vi "SpectrometerSpinCoater_v14.vi"() -> ()   [LabVIEW 2020]
uses:
  TypDef/TabControl_InSitu_Type.ctl
  <instrlib>/Classes/CCD/Abstract_CCD/Abstract_CCD.lvclass
  <instrlib>/Classes/SpinCoater/SpinCoater.lvclass
  TypDef/Preset_Save_v14_1.ctl
  TypDef/DeviceQueue_TypeDef.ctl
  TypDef/DeviceQueue_Action.ctl
  TypDef/TabControl.ctl
  TypDef/DataQueue_TypeDef.ctl
  TypDef/DataQueue_Action.ctl
  <vilib>/Utility/error.llb/DialogType.ctl
  <instrlib>/Classes/CCD/Avantes/Avantes.lvclass
  C:/Program Files/National Instruments/LabVIEW 2020/instr.lib/Classes/CCD/Abstract_CCD/Abstract_CCD.lvclass
  <vilib>/Analysis/baseanly.llb/A x Vector.vi
  <vilib>/Utility/xml.llb/Write to XML File(string).vi
  <vilib>/Utility/xml.llb/Read From XML File(string).vi
  <vilib>/Analysis/NI_AALBase.lvlib
panel:
  out "fName_Temp":string
  out "x-y":dbl
  in  "Reference\nValue":dbl=1.0
  out "WL-Det\nPos":i32
  in  "Motor_ShortStop":bool
  out "UpperWLLimit":i32=1065
  out "LowerWLLimit":i32=149
  out "Nr After Spin":u16
  out "Action":string="TimeOut"
  out "Time.spin":refnum<file>
  out "Meas.spin":refnum<file>
  in  "Abort Button":bool
  in  "Stop Button":bool=TRUE
  in  "Tab Control":T1(tab)=enum."Settings"
  in  "MeasureOpenPreset":bool
  in  "MeasureSavePreset":bool
  in  "Cell":string
  in  "TrimSpec":bool=TRUE caption="Trim\nSpec"
  in  "WlUp":dbl[unit]=9.102385253906251e-07 caption="Wl \nUp"
  in  "WlLow":dbl[unit]=3.7998095703125003e-07 caption="Wl \nLow"
  in  "Frames for Ref/Dark":dbl=10000.0
  in  "Shutter Toggle":bool
  in  "Program Spin Coater":T2(array[cluster])=[{"Speed (rpm)"=1430.0, "Time (s)"=45.0, "Acc (rpm/s)"=0.0}]
  in  "Spectra Count":u16
  in  "Measure_MeasureSpectrum":bool
  out "Overall Time":dbl=47.0
  in  "Frames":i32=123685
  in  "StartMeasurement_Button":bool
  in  "Measure_Preview":bool
  out "Measure_Graph":T3(graph) caption="XY Graph"
  in  "Measure_FramesSpectrometer":dbl=200.0 caption="Frames for Spectrometer"
  in  "StartSpin_Button":bool
  in  "Record RefSpec":bool
  in  "Measure:\nRecord_Darkspec":bool
  in  "Measure_Comments":string="Just for testing" caption="Comments"
  in  "Measure_FileName":string="Testing" caption="File Name"
  in  "Measure_SavePath":path=path "C:/Users/Cerberus/Desktop/Test/v12Test" caption="Save Path"
  out "Measure_FrameRate":dbl[unit]=2631.5791015625 caption="Frame Rate"
  in  "Measure_IntegrationTime":dbl[unit]=3e-05 caption="Integration Time"
  in  "Tab Control SpinType":T4
  in  "Seconds after Spin":dbl[unit]=1.0
  in  "Calculate Frames_Normal":bool=TRUE caption="Calculate Frames"
  in  "periodic time":dbl[unit]=2.0
  in  "Duration after":dbl[unit]
  in  "Spin at end":bool
  in  "Seconds to Spin_Normal":dbl[unit]=1.0 caption="Seconds to Spin"
  in  "Threshold":dbl=0.3
  in  "Time Detect":dbl[unit]=2.0
  in  "Seconds to Spin_Short":dbl[unit]=1.0 caption="Seconds to Spin"
  in  "Spin Time":dbl[unit]=2.0
  in  "Calculate Frames_Short":bool=TRUE caption="Calculate Frames"
  in  "Wavelenght Detect":dbl[unit]=6.000000000000001e-07
  out "SS_StepsLeft":dbl
  out "SS_TimePrediction":dbl[unit]=-6.0
  out "Horizontal Progress Bar":u8(slide) scale=0.0..100.0
  in  "SpectralStability:\nRecord_Darkspec":bool
  in  "SpectralStability_Record":bool
  in  "SpectralStability_\nMeasurementNumber":u32 caption="Measurement Number"
  in  "SpectralStability_Duration":dbl[unit] caption="Duration"
  in  "Duration/Times":bool
  in  "SpectralStability_\nPeriodicTime":dbl[unit] caption="Periodic Time"
  in  "SpectralStability_MeasureSpectrum":bool
  in  "SpectralStability_Preview":bool
  out "SpectralStability_Graph":T3(graph) caption="XY Graph"
  in  "SpectralStability_FramesSpectrometer":dbl=200.0 caption="Frames for Spectrometer"
  in  "SpectralStability_Comments":string="Just for testing" caption="Comments"
  in  "SpectralStability_FileName":string="TestingAfter" caption="File Name"
  in  "SpectralStability_SavePath":path=path "C:/Users/Timo/Desktop/Test/180824" caption="Save Path"
  out "SpectralStability_FrameRate":dbl[unit]=2631.5791015625 caption="Frame Rate"
  in  "SpectralStability_IntegrationTime":dbl[unit]=3e-05 caption="Integration Time"
  in  "Shutter Close":bool
  in  "Shutter Open":bool
  in  "SHUTTER DEBUG":bool
  in  "Shutter Position":u16=1000
  in  "Dividider Get Spectra":u32=1 min=1
  in  "Automatically \nadjust count":bool=TRUE
  in  "Reset Count\nafter Spin Coating":bool=TRUE
  in  "ESC_Speed":dbl
  in  "ESC_Milliseconds":dbl
  in  "ESC DEBUG":bool
  in  "Port Arduino":refnum<visa-resource-name>="COM7"
  out "Error Arduino":bool caption="Error"
  in  "Init_Arduino":bool caption="Init"
  out "Caption_Settings_Arduino":string="Arduino"
  out "Caption_Settings_NKT":string="NKT Laser"
  out "Error_Spectromter":bool caption="Error"
  in  "Init_Spectrometer":bool caption="Init"
  out "Caption_Settings_Spectrometer":string="Spectromter"
  out "Arduino":bool
  out "NKT":bool
  out "Spectromter":bool
  # "Speed (rpm)   Time (s)        Acceleration \n                                               (rpm/s)"
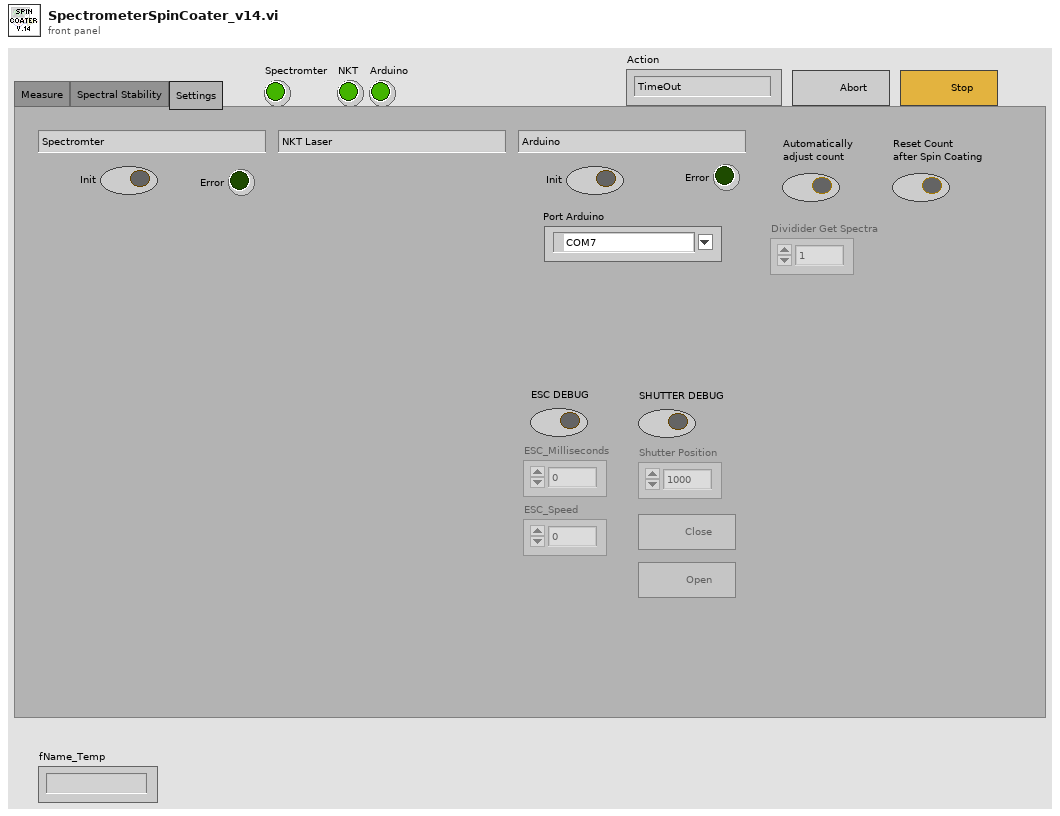
[diagram p1: front panel]
types:
  T1 = enum32{"Measure", "Spectral Stability", "Settings"}
  T2 = cluster{"Speed (rpm)":dbl, "Time (s)":dbl, "Acc (rpm/s)":dbl}[]
  T3 = cluster{"Wavlength":dbl[unit][], "Image":dbl[]}[]
  T4 = typedef "TabControl_InSitu_Type.ctl" = enum32{"Normal", "Short"}
  T5 = cluster{"Dark":cluster{"Image":dbl[][][], "Frame Size":cluster{"F":i32, "Y":i32, "X":i32}}[], "Ref":cluster{"Image":dbl[][][], "Frame Size":cluster{"F":i32, "Y":i32, "X":i32}}[], "Wavlength":dbl[unit][], "Wavlength Trim":dbl[unit][], "spec":dbl[][]}
  T6 = cluster{"Abstract_CCD.lvclass":refnum<class "Abstract_CCD.lvclass">, "SpinCoater.lvclass":refnum<class "SpinCoater.lvclass">}
  T7 = enum8{"Enabled", "Disabled", "Disabled and Grayed Out"}
  T8 = typedef "DataQueue_TypeDef.ctl" = cluster{"QueueAction":T9, "Data":cluster{"Image":dbl[][][], "Frame Size":cluster{"F":i32, "Y":i32, "X":i32}}[], "Data_Raw":cluster{"Image":dbl[][][], "Frame Size":cluster{"F":i32, "Y":i32, "X":i32}}[], "Data_Dark":cluster{"Image":dbl[][][], "Frame Size":cluster{"F":i32, "Y":i32, "X":i32}}[], "Data_Ref":cluster{"Image":dbl[][][], "Frame Size":cluster{"F":i32, "Y":i32, "X":i32}}[], "Device Information":string[], "Numeric Control":dbl, "Boolean":bool, "Wavelength":dbl[unit][], "Time":dbl[], "Time Stamp":timestamp, "Numeric Control 2":dbl, "TabControl":T10, "Numeric Control 3":dbl}
  T9 = typedef "DataQueue_Action.ctl" = enum16{"TimeOut", "Close_Program", "Abort", "Stop_Measurement", "Measure_InSituSpinCoating", "Measure_InSituSpinCoating_Short", "Measure_Spectrum", "Measure_SpectrumAdvanced", "Measure_SpectralStability", "Save_InSitu", "Save_SpectralStability", "Set_Ref", "Set_Dark", "Set_Wavelength", "Spectrometer_Measure", "Spectrometer_Preview", "Transfer_Settings", "Change_TrimSettings"}
  T10 = typedef "TabControl.ctl" = enum16{"Measure", "Spectral Stability", "Settings"}
  T11 = typedef "DeviceQueue_TypeDef.ctl" = cluster{"QueueAction":T12, "Numeric 1":dbl, "Numeric 2":dbl, "Boolean 1":bool, "Boolean 2":bool, "Spin Program":dbl[][], "Spin Prg v07":cluster{"Speed (rpm)":dbl, "Time (s)":dbl, "Acc (rpm/s)":dbl}[], "Time Stamp":timestamp, "TabControl":T10}
  T12 = typedef "DeviceQueue_Action.ctl" = enum16{"TimeOut", "Wait", "Close_Program", "Abort", "Spectrometer_Init", "Spectrometer_Close", "Spectrometer_DeviceInformation", "Spectrometer_Measure", "Spectrometer_MeasureAdvanced", "Spectrometer_Preview", "Spectrometer_Abort", "Spectrometer_StartMeasurement", "Spectrometer_GetData", "Spectrometer_GetData_Short", "Spectrometer_StopMeasurement", "Spectrometer_SetIntegrationTime", "Spectrometer_SetFrames", "Spectrometer_SetDarkspec", "Spectrometer_SetReference", "Spectrometer_SetTriggerMode", "Laser_Init", "Laser_Close", "Arduino_Init", "Arduino_Close", "Arduino_LoadProgram", "Arduino_StartProgram", "Arduino_SetSpeed", "Arduino_SetMillis", "Arduino_StopSpin", "Arduino_ShortStop", "Arduino_Shutter_SetPosition", "Arduino_Shutter_Close", "Arduino_Shutter_Open", "Measure_InSitu", "Measure_Spectrum", "Measure_InSituAdvanced", "Measure_InSituAdvanced_Short", "Measure_SpectralStability", "Measure_Stop"}
  T13 = enum16{"open", "replace", "create", "open or create", "replace or create", "replace or create with confirmation"}
  T14 = cluster{"Image":dbl[][][], "Frame Size":cluster{"F":i32, "Y":i32, "X":i32}}[]
  T15 = cluster{"Image":dbl[][][], "Frame Size":cluster{"F":i32, "Y":i32, "X":i32}}
  T16 = cluster{"Wavlength":dbl[unit][], "A x Vector":dbl[]}
  T17 = cluster{"Wavlength":dbl[unit][], "A x Vector":dbl[]}[]
  T18 = cluster{u16[][][], u16[][][], dbl[], "Numeric Control":dbl, "Numeric Control 2":dbl}
  T19 = typedef "DialogType.ctl" = u16
  T20 = typedef "Preset_Save_v14_1.ctl" = cluster{"Measure_IntegrationTime":dbl, "Measure_FramesSpec":dbl, "Frames_ForRef/Dark":dbl, "Program Spin Coater":cluster{"Speed (rpm)":dbl, "Time (s)":dbl, "Acc (rpm/s)":dbl}[], "TabControlSpinType":u32, "Seconds2Spin_Norm":dbl, "SecondsAftSpin_Norm":dbl, "CalcFrames_Norm":bool, "PeriodicTime":dbl, "DurationAfter":dbl, "SpinAtEnd":bool, "Seconds2Spin_Short":dbl, "SpinTime":dbl, "CalculateFrames_Short":bool, "TimeDetect":dbl, "WavelengthDetect":dbl, "Threshold":dbl, "WlLow":dbl, "WlUp":dbl, "TrimSpec":bool}
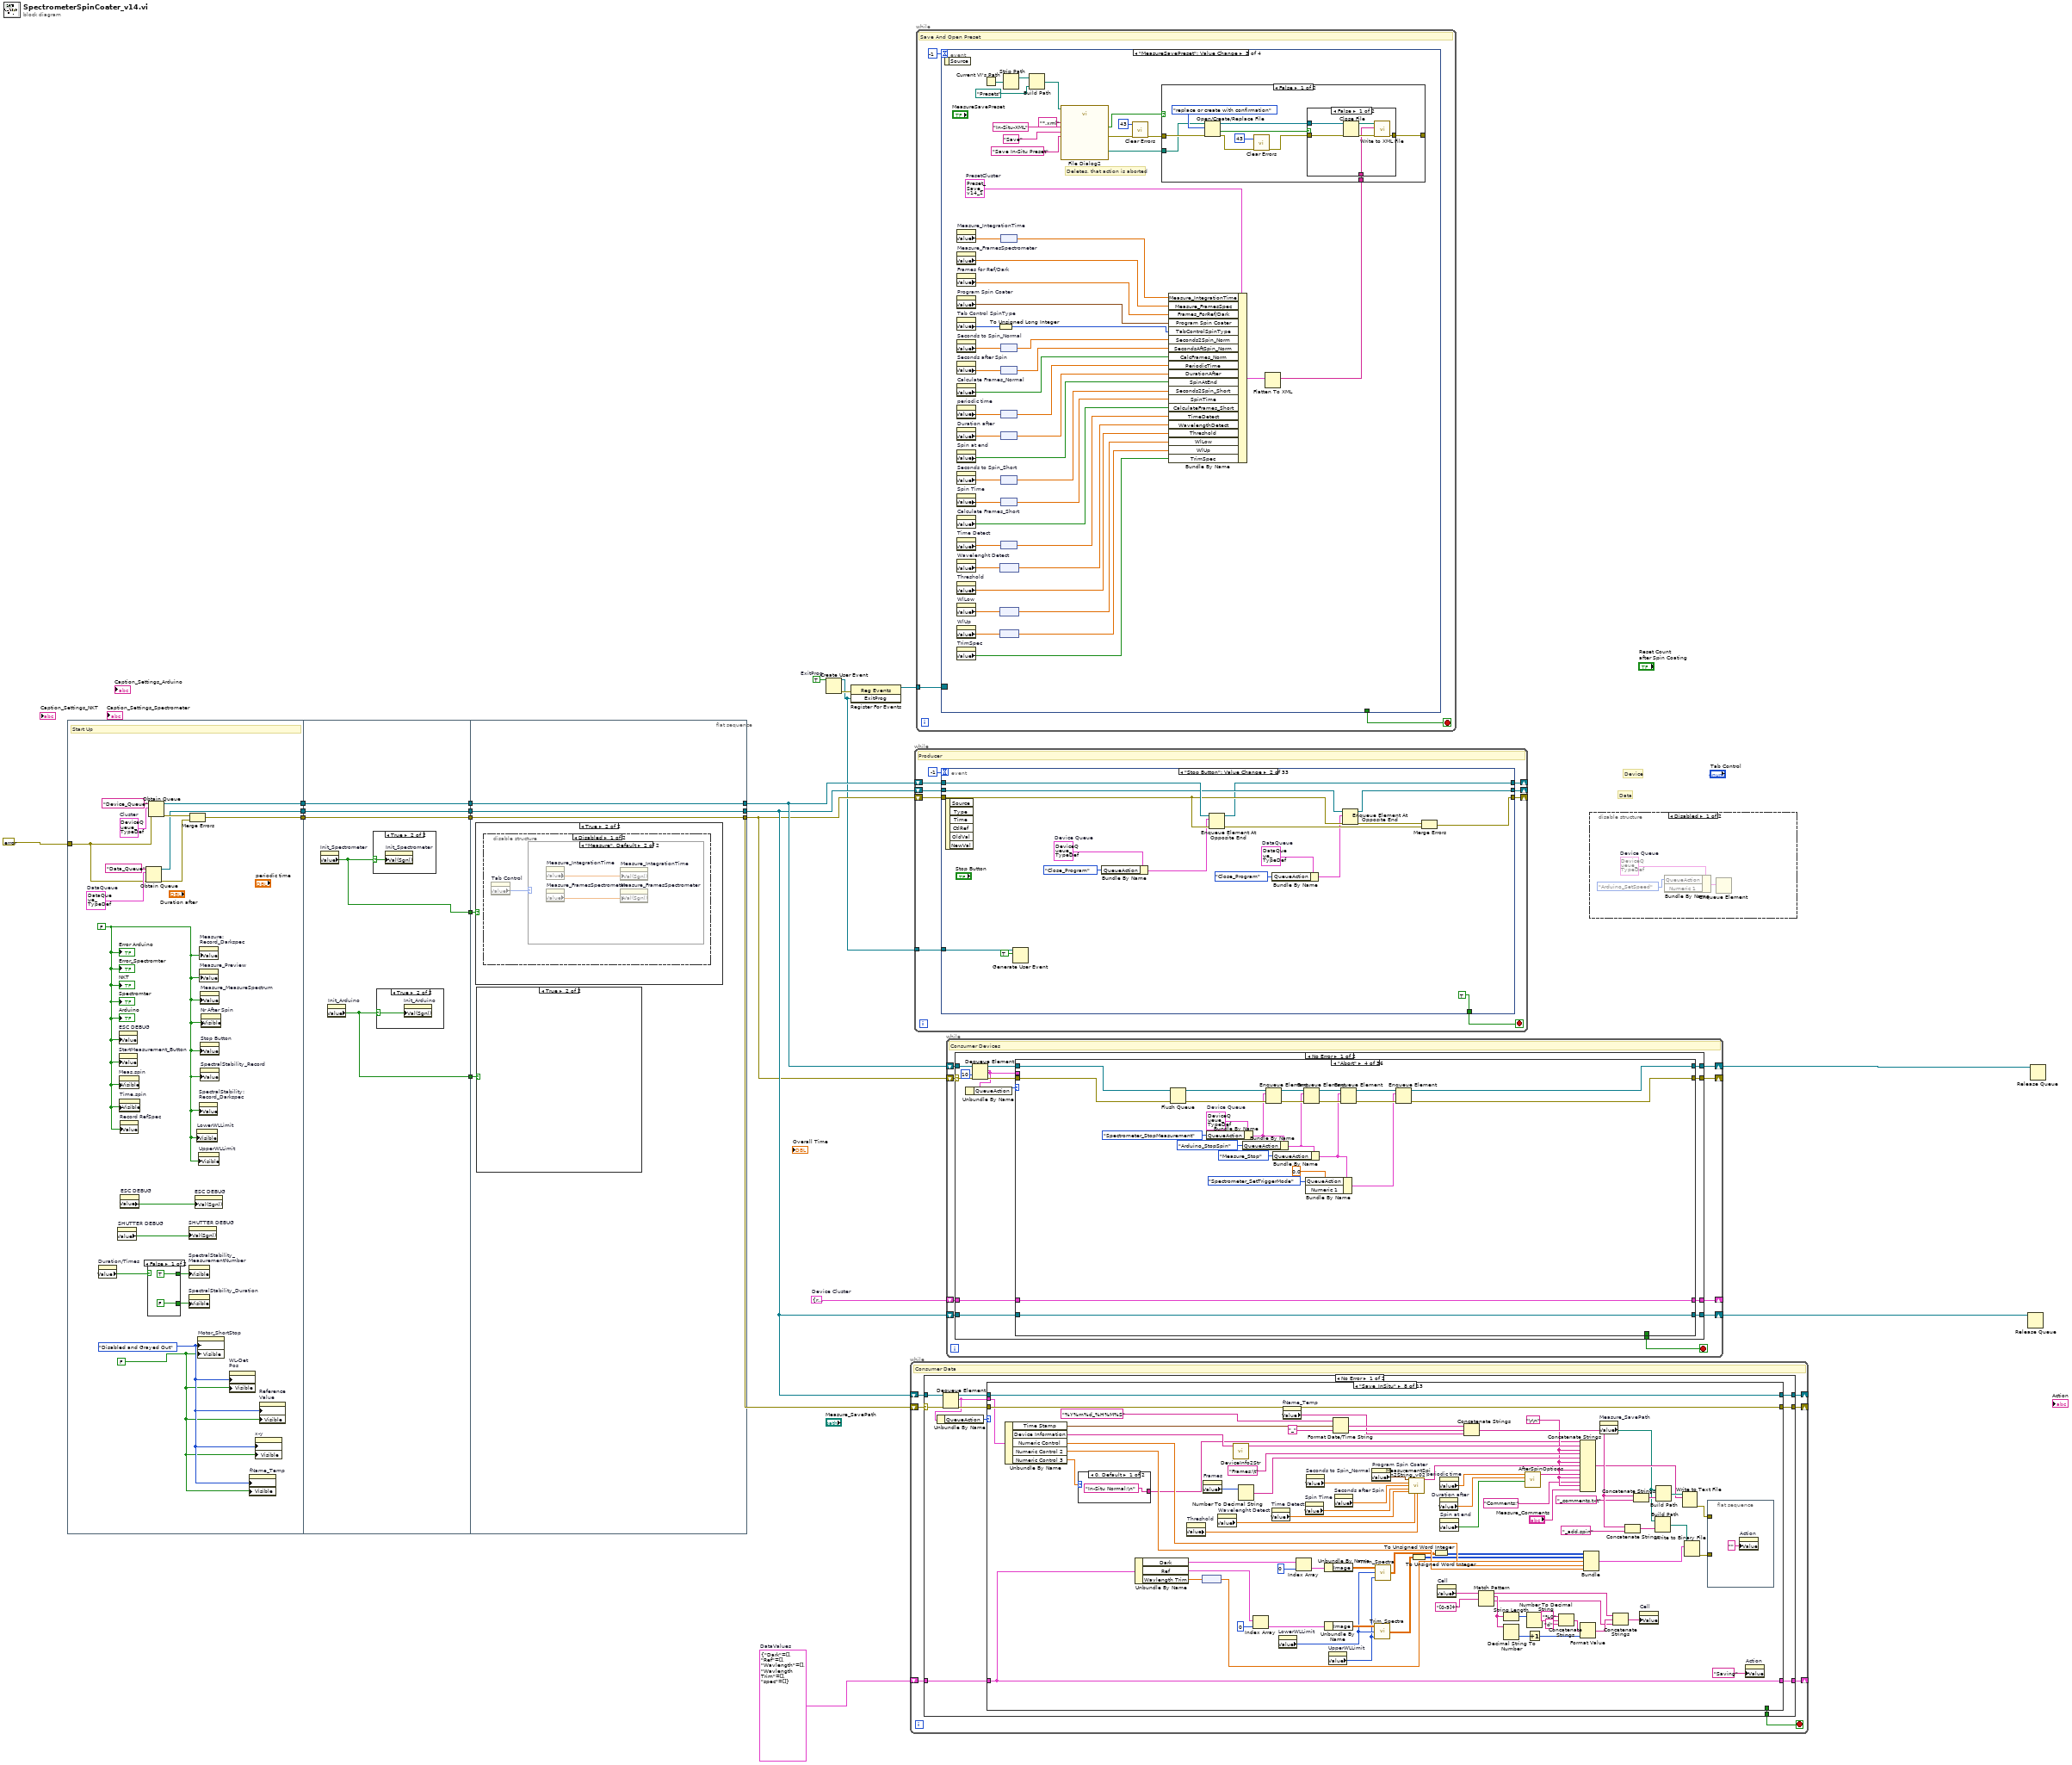
[diagram p0: block diagram]
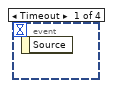
[diagram p2: hidden frame]
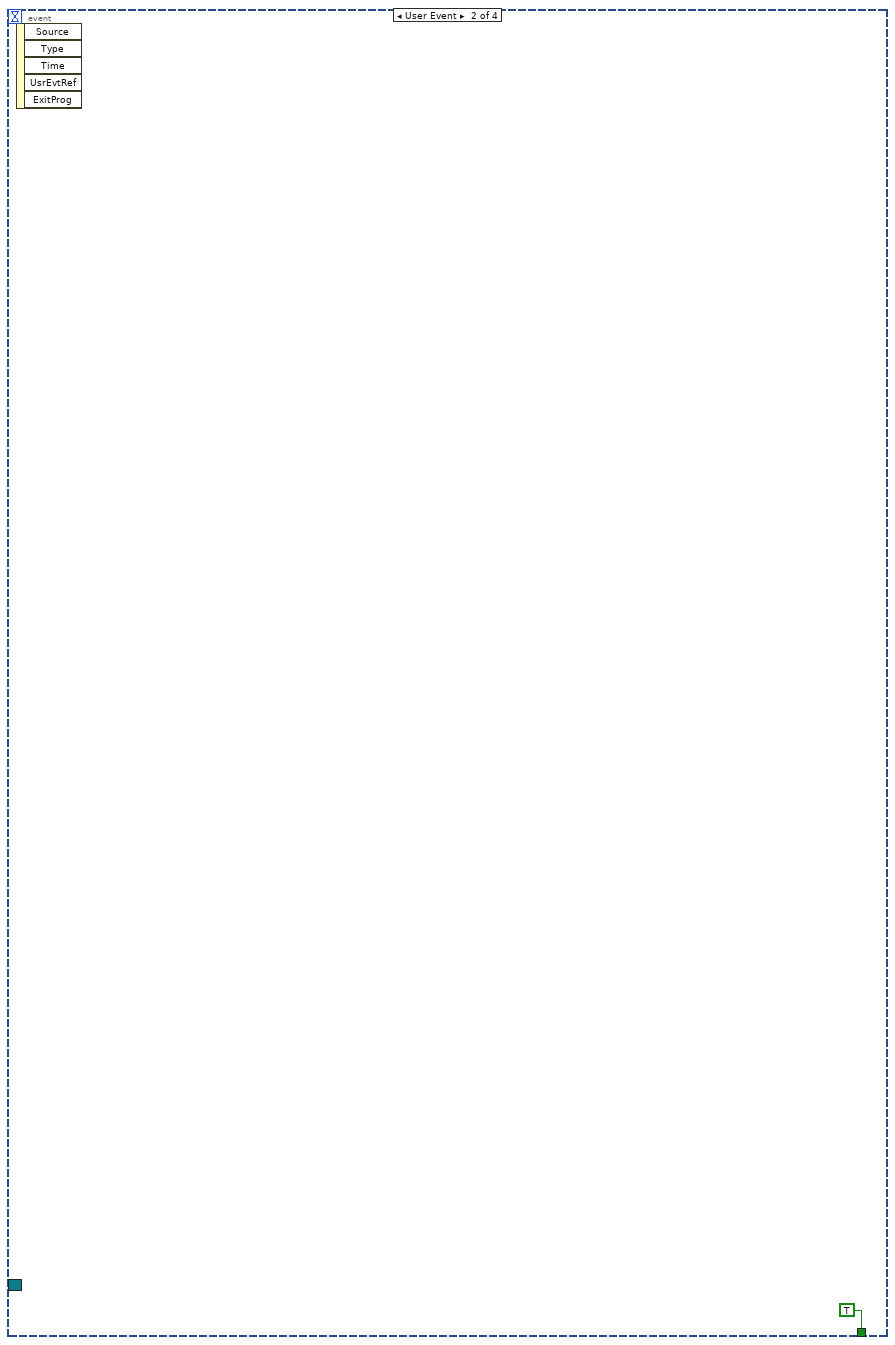
[diagram p3: hidden frame]
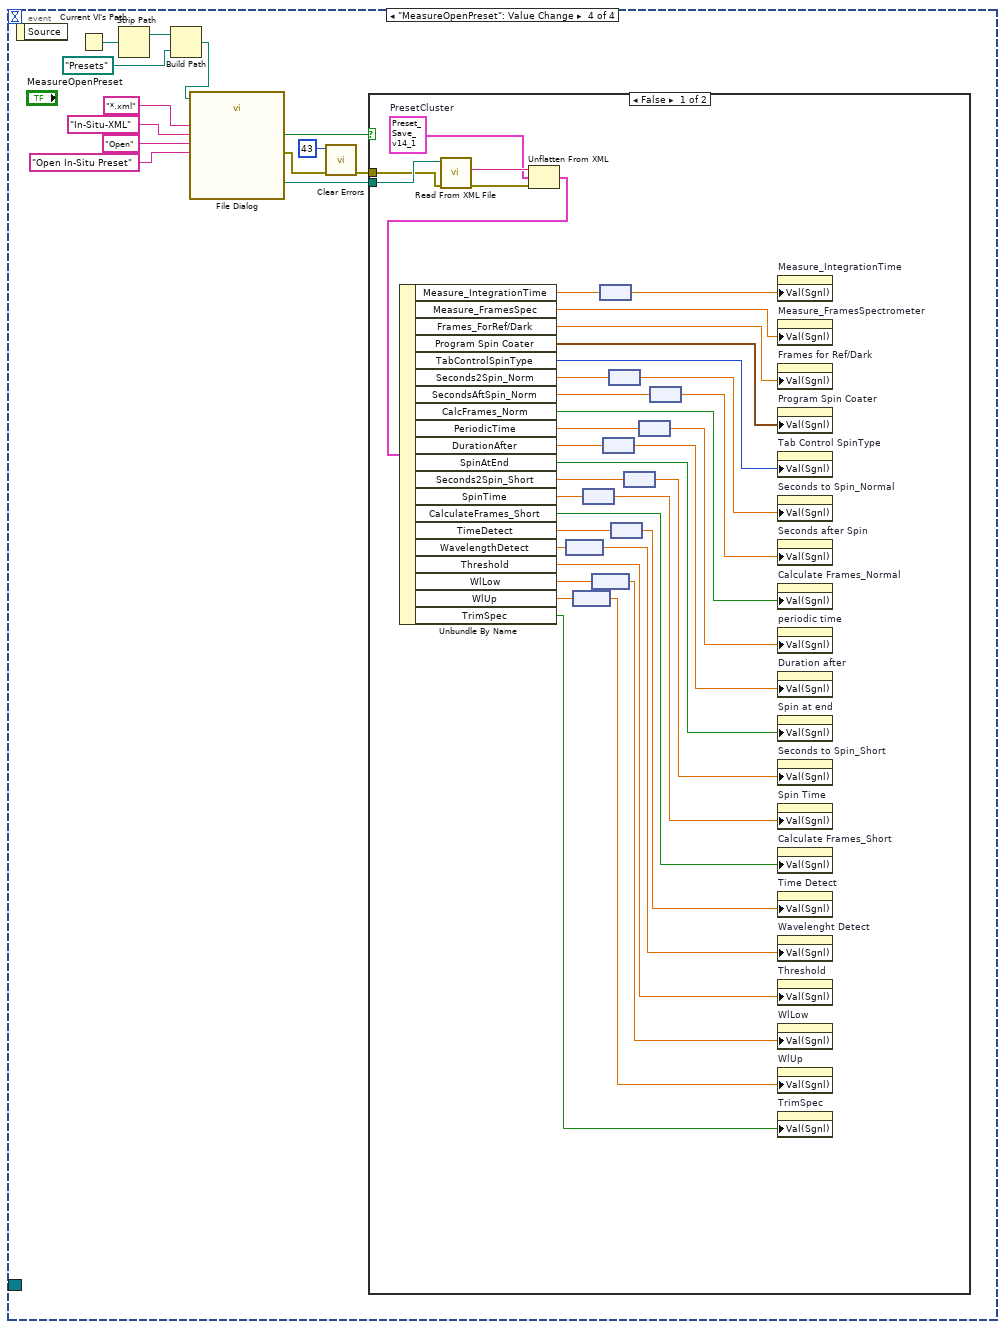
[diagram p6: hidden frame]
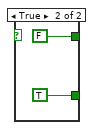
[diagram p9: hidden frame]
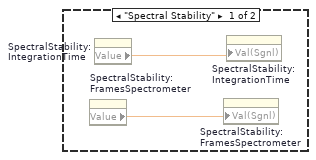
[diagram p14: hidden frame]
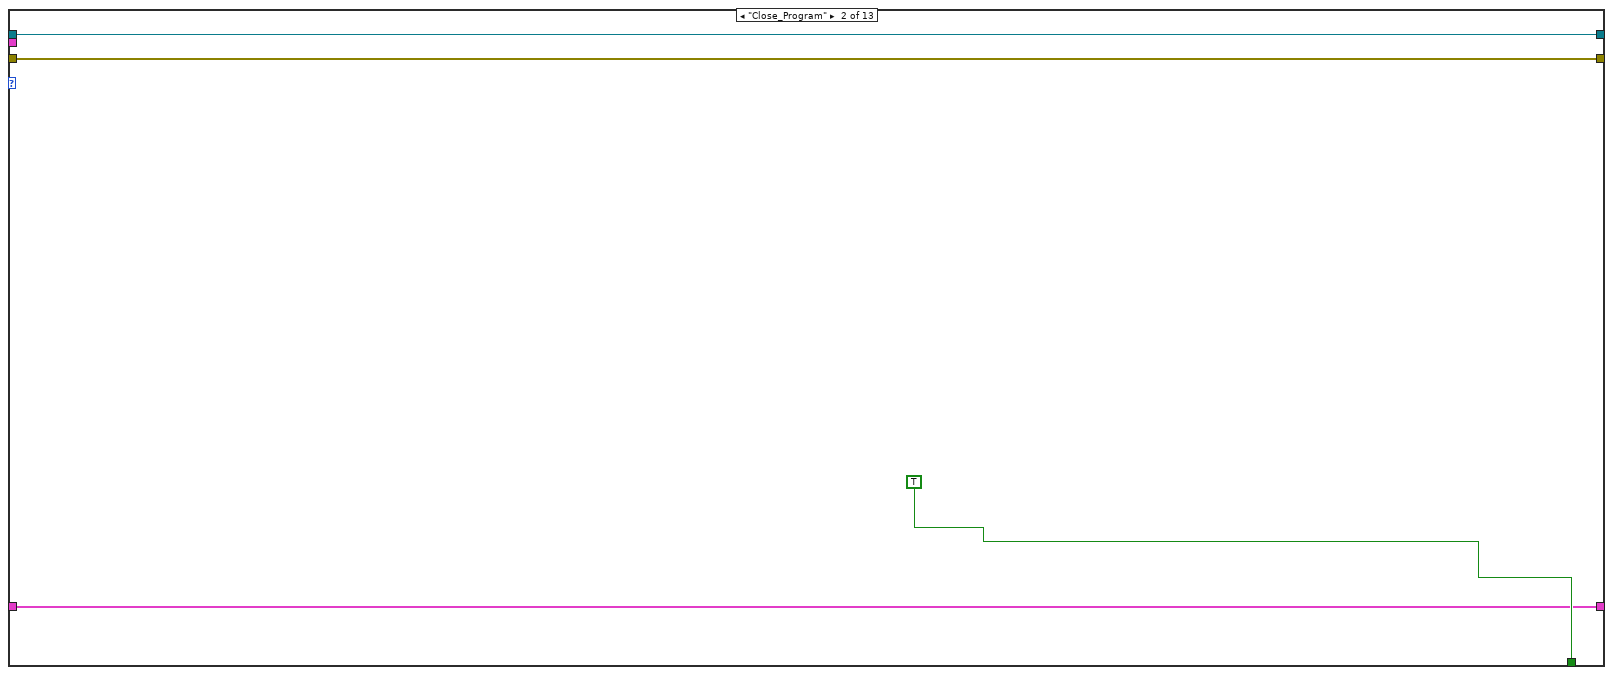
[diagram p17: hidden frame]
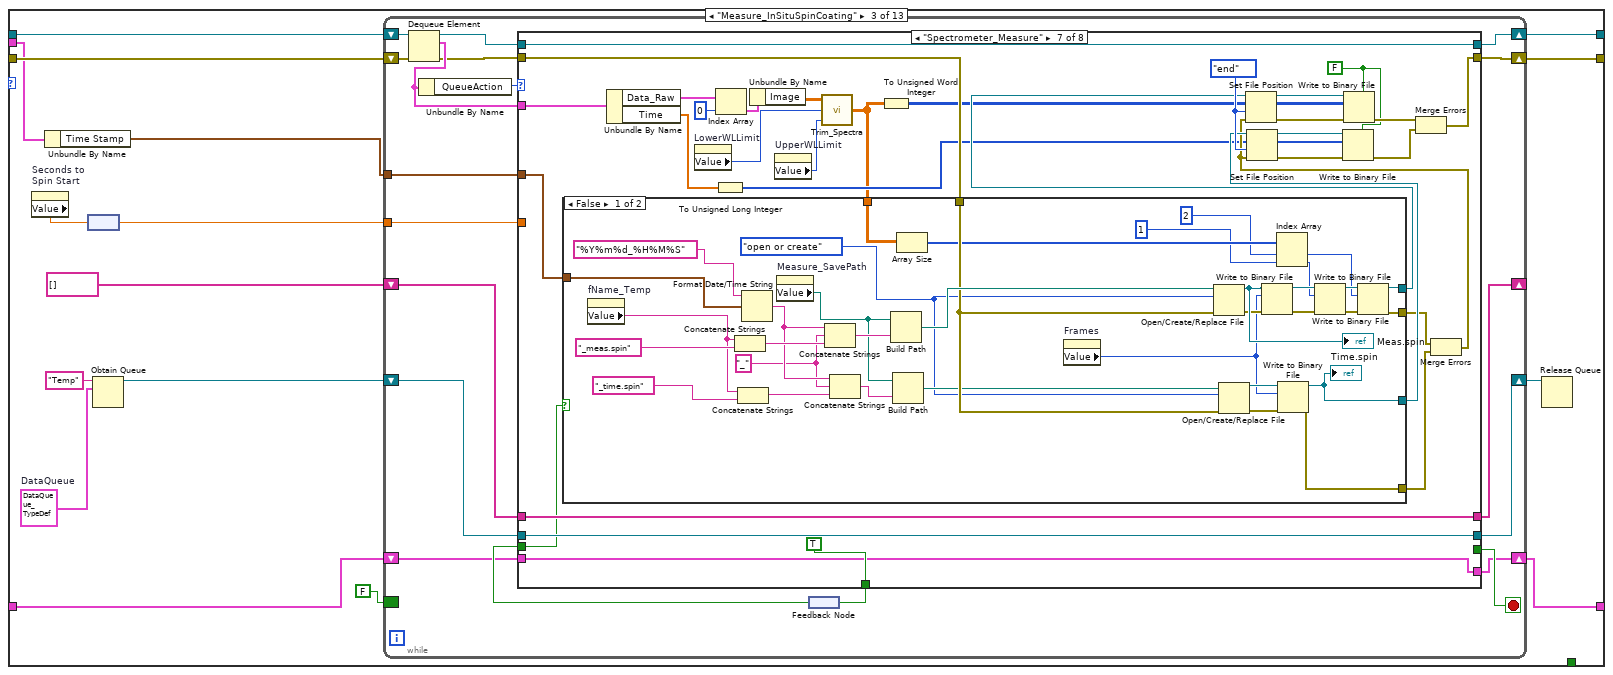
[diagram p18: hidden frame]
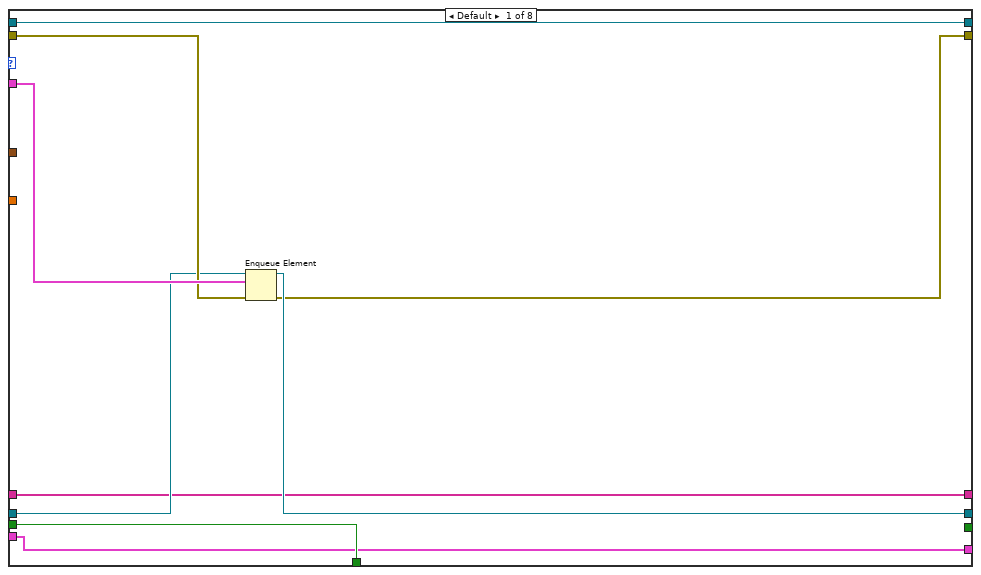
[diagram p19: hidden frame]
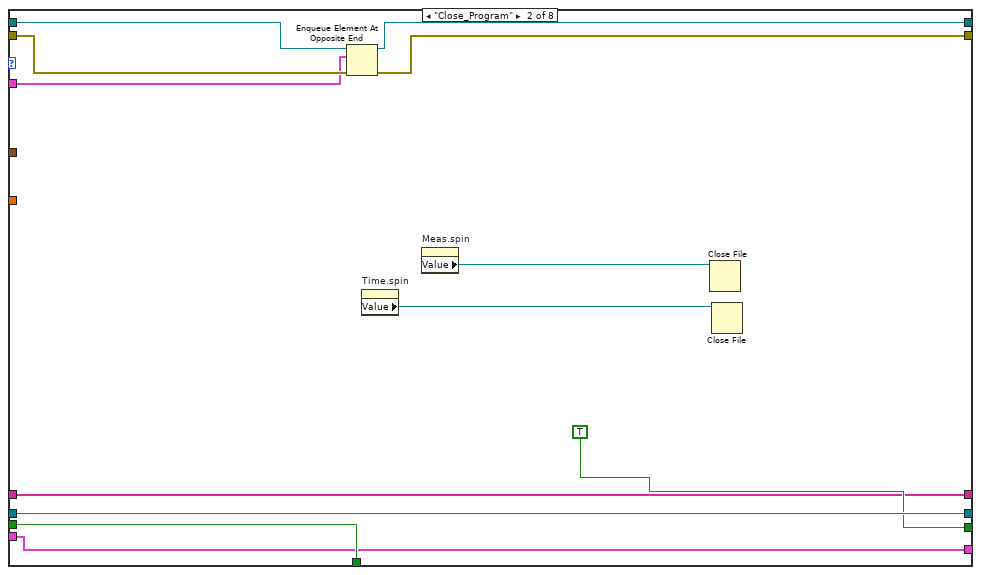
[diagram p20: hidden frame]
diagram:
  w4 = TRUE  # ExitProg
  w11 = T5 {"Dark"=[], "Ref"=[], "Wavlength"=[], "Wavlength Trim"=[], "spec"=[]}  # DataValues
  w15 = T6 {"Abstract_CCD.lvclass"=refnum, "SpinCoater.lvclass"=refnum}  # Device Cluster
  # "Data"
  # "Device"
  n1 = flat-sequence {
    tunnel: errorcluster {"status"=FALSE, "code"=0, "source"=""} ("error constant") -> [w33]
    tunnel: [w36] -> w19
    tunnel: [w30] -> w18
    tunnel: [w29] -> w17
    tunnel: w19 -> [w47]
    tunnel: w18 -> [w46]
    tunnel: w17 -> [w45]
    tunnel: [w47] -> w10
    tunnel: [w46] -> w9
    tunnel: [w45] -> w8
    tunnel: [w44] -> w7
    tunnel: [w43] -> w6
    tunnel: [w52] -> w5
    tunnel: [w53] -> w12
    tunnel: [w54] -> w16
    tunnel: w10 -> [w54]
    tunnel: w9 -> [w53]
    tunnel: w8 -> [w52]
    tunnel: w7 -> [w51]
    tunnel: w6 -> [w50]
    frame #0 {
      w22 = T7."Disabled and Grayed Out" ("Disabled")
      w21 = FALSE ("Visible")
      w34 = T8 {"QueueAction"=enum."TimeOut", "Data"=[], "Data_Raw"=[], "Data_Dark"=[], "Data_Ref"=[], "Device Information"=[], "Numeric Control"=0.0, "Boolean"=FALSE, "Wavelength"=[], "Time"=[], "Time Stamp"=timestamp(0 s since 1904-01-01), "Numeric Control 2"=0.0, "TabControl"=enum."Measure", "Numeric Control 3"=0.0}  # DataQueue
      w37 = T11 {"QueueAction"=enum."TimeOut", "Numeric 1"=0.0, "Numeric 2"=0.0, "Boolean 1"=FALSE, "Boolean 2"=FALSE, "Spin Program"=[], "Spin Prg v07"=[], "Time Stamp"=timestamp(0 s since 1904-01-01), "TabControl"=enum."Measure"}  # Cluster
      w23 = FALSE ("Error Arduino")
      # "Start Up"
      n2 = property on="Duration/Times" class="Bool (strict)"() -> ("Value"=w25:bool)  [unwired: 2 in, 2 out]
      n3 = property on="SHUTTER DEBUG" class="Bool (strict)"() -> ("Value"=w24:bool)  [unwired: 2 in, 2 out]
      n4 = property on="ESC DEBUG" class="Bool (strict)"("Value"=w23) -> ()  [unwired: 2 in, 2 out]
      n5 = property on="StartMeasurement_Button" class="Bool (strict)"("Value"=w23) -> ()  [unwired: 2 in, 2 out]
      n6 = property on="Meas.spin" class="Ref (strict)"("Visible"=w23) -> ()  [unwired: 2 in, 2 out]
      n7 = property on="Time.spin" class="Ref (strict)"("Visible"=w23) -> ()  [unwired: 2 in, 2 out]
      n8 = property on="Record RefSpec" class="Bool (strict)"("Value"=w23) -> ()  [unwired: 2 in, 2 out]
      n9 = property on="ESC DEBUG" class="Bool (strict)"() -> ("Value"=w28:bool)  [unwired: 2 in, 2 out]
      n10 = Obtain Queue(name (unnamed)="Data_Queue", element data type=w34, error in (no error)=w33) -> (queue out=w30:refnum<queue>, error out=w31:errorcluster)  [unwired: 2 in, 1 out]
      n11 = case shown="False" w25 {
        tunnel: [FALSE TRUE] -> w27
        tunnel: [TRUE FALSE] -> w26
        frame False {
        }
        frame True {
        }
      }
      n12 = Obtain Queue(name (unnamed)="Device_Queue", element data type=w37, error in (no error)=w33) -> (queue out=w36:refnum<queue>, error out=w32:errorcluster)  [unwired: 2 in, 1 out]
      n13 = property on="SHUTTER DEBUG" class="Bool (strict)"("Val(Sgnl)"=w24) -> ()  [unwired: 2 in, 2 out]
      n14 = property on="SpectralStability_\nMeasurementNumber" class="DigNum (strict)"("Visible"=w26) -> ()  [unwired: 2 in, 2 out]
      n15 = property on="SpectralStability_Duration" class="DigNum (strict)"("Visible"=w27) -> ()  [unwired: 2 in, 2 out]
      n16 = Merge Errors(w32, w31) -> (w29:errorcluster)
      n17 = property on="ESC DEBUG" class="Bool (strict)"("Val(Sgnl)"=w28) -> ()  [unwired: 2 in, 2 out]
      n18 = property on="LowerWLLimit" class="DigNum (strict)"("Visible"=w23) -> ()  [unwired: 2 in, 2 out]
      n19 = property on="Motor_ShortStop" class="Bool (strict)"("DisabledEnum"=w22, "Visible"=w21) -> ()  [unwired: 2 in, 2 out]
      n20 = property on="UpperWLLimit" class="DigNum (strict)"("Visible"=w23) -> ()  [unwired: 2 in, 2 out]
      n21 = property on="SpectralStability:\nRecord_Darkspec" class="Bool (strict)"("Value"=w23) -> ()  [unwired: 2 in, 2 out]
      n22 = property on="Measure:\nRecord_Darkspec" class="Bool (strict)"("Value"=w23) -> ()  [unwired: 2 in, 2 out]
      n23 = property on="Measure_Preview" class="Bool (strict)"("Value"=w23) -> ()  [unwired: 2 in, 2 out]
      n24 = property on="Measure_MeasureSpectrum" class="Bool (strict)"("Value"=w23) -> ()  [unwired: 2 in, 2 out]
      n25 = property on="Stop Button" class="Bool (strict)"("Value"=w23) -> ()  [unwired: 2 in, 2 out]
      n26 = property on="SpectralStability_Record" class="Bool (strict)"("Value"=w23) -> ()  [unwired: 2 in, 2 out]
      n27 = property on="Nr After Spin" class="DigNum (strict)"("Visible"=w23) -> ()  [unwired: 2 in, 2 out]
      n28 = property on="WL-Det\nPos" class="DigNum (strict)"("DisabledEnum"=w22, "Visible"=w21) -> ()  [unwired: 2 in, 2 out]
      n29 = property on="fName_Temp" class="Str"("DisabledEnum"=w22, "Visible"=w21) -> ()  [unwired: 2 in, 2 out]
      n30 = property on="x-y" class="DigNum (strict)"("DisabledEnum"=w22, "Visible"=w21) -> ()  [unwired: 2 in, 2 out]
      n31 = property on="Reference\nValue" class="DigNum (strict)"("DisabledEnum"=w22, "Visible"=w21) -> ()  [unwired: 2 in, 2 out]
      "Error_Spectromter" <- w23
      "Error Arduino" <- w23
      "Spectromter" <- w23
      "NKT" <- w23
      "Arduino" <- w23
    }
    frame #1 {
      n32 = property on="Init_Spectrometer" class="Bool (strict)"() -> ("Value"=w44:bool)  [unwired: 2 in, 2 out]
      n33 = property on="Init_Arduino" class="Bool (strict)"() -> ("Value"=w43:bool)  [unwired: 2 in, 2 out]
      n34 = case shown="True" w44 {
        selector: w44 -> [_ w49]
        frame False {
        }
        frame True {
          n35 = property on="Init_Spectrometer" class="Bool (strict)"("Val(Sgnl)"=w49) -> ()  [unwired: 2 in, 2 out]
        }
      }
      n36 = case shown="True" w43 {
        selector: w43 -> [_ w48]
        frame False {
        }
        frame True {
          n37 = property on="Init_Arduino" class="Bool (strict)"("Val(Sgnl)"=w48) -> ()  [unwired: 2 in, 2 out]
        }
      }
    }
    frame #2 {
      n38 = case shown="True" w51 {
        frame False {
        }
        frame True {
          n39 = disable-structure shown="Disabled" {
            frame Disabled {
              n40 = property on="Tab Control" class="TabCtl (strict)"() -> ("Value"=w55:T1)  [unwired: 2 in, 2 out]
              n41 = case shown="\"Measure\", Default" w55 {
                frame "Spectral Stability" {
                  n42 = property on="SpectralStability:\nFramesSpectrometer" class="DigNum (strict)"() -> ("Value"=w56:dbl)  [unwired: 2 in, 2 out]
                  n43 = property on="SpectralStability:\nIntegrationTime" class="DigNum (strict)"() -> ("Value"=w57:dbl[unit])  [unwired: 2 in, 2 out]
                  n44 = property on="SpectralStability:\nFramesSpectrometer" class="DigNum (strict)"("Val(Sgnl)"=w56) -> ()  [unwired: 2 in, 2 out]
                  n45 = property on="SpectralStability:\nIntegrationTime" class="DigNum (strict)"("Val(Sgnl)"=w57) -> ()  [unwired: 2 in, 2 out]
                }
                frame "Measure", Default {
                  n46 = property on="Measure_IntegrationTime" class="DigNum (strict)"() -> ("Value"=w58:dbl[unit])  [unwired: 2 in, 2 out]
                  n47 = property on="Measure_FramesSpectrometer" class="DigNum (strict)"() -> ("Value"=w59:dbl)  [unwired: 2 in, 2 out]
                  n48 = property on="Measure_IntegrationTime" class="DigNum (strict)"("Val(Sgnl)"=w58) -> ()  [unwired: 2 in, 2 out]
                  n49 = property on="Measure_FramesSpectrometer" class="DigNum (strict)"("Val(Sgnl)"=w59) -> ()  [unwired: 2 in, 2 out]
                }
              }
            }
            frame Enabled {
            }
          }
        }
      }
      n50 = case shown="True" w50 {
        frame False {
        }
        frame True {
        }
      }
    }
  }
  n51 = Create User Event(user event datatype=w4) -> (user event=w2:refnum<user-event>, error out=w3:errorcluster)  [unwired: 1 in]
  n52 = register-events(error in=w3, w2) -> (reference out=w1:refnum<event-registration>)  [unwired: 1 in, 1 out]
  n53 = while {
    shift-right: [w60] -> _
    shift-left: w5 -> [w66]
    shift-right: [w61] -> _
    shift-left: w12 -> [w65]
    shift-right: [w62] -> _
    shift-left: w11 -> [w64]
    stop <- w63 stop-if-true
    # "Consumer Data"
    n54 = case shown="No Error" w66 {
      selector: w66 -> [w77 w1071]
      tunnel: w65 -> [w76 w1072]
      tunnel: w64 -> [w74 w1069]
      tunnel: [w73 _] -> w63
      tunnel: [w72 w1069] -> w62
      tunnel: [w71 w1072] -> w61
      tunnel: [w69 w1070] -> w60
      frame No Error {
        n55 = Dequeue Element(queue=w76, error in (no error)=w77) -> (queue out=w70:refnum<queue>, element=w67:T8, error out=w68:errorcluster)  [unwired: 1 in, 1 out]
        n56 = Unbundle By Name(w67) -> ("QueueAction"=w75:T9)
        n57 = case shown="\"Save_InSitu\"" w75 {
          tunnel: w74 -> [w78 w83 w85 w298 w506 w613 w717 w950 w987 w996 w1019 w1032 w1039]
          tunnel: [_ TRUE _ _ _ _ _ _ _ _ _ _ _] -> w73
          tunnel: [w78 w83 w87 w300 w506 w613 w708 w950 w991 w1010 w1018 w1032 w1038] -> w72
          tunnel: [w80 w82 w100 w313 w512 w619 w701 w972 w992 w1011 w1015 w1034 w1045] -> w71
          tunnel: w70 -> [w80 w82 w98 w311 w513 w620 w712 w972 w992 w1011 w1015 w1034 w1045]
          tunnel: [w79 w81 w99 w312 w511 w618 w702 w971 w993 w1012 w1016 w1033 w1042] -> w69
          tunnel: w68 -> [w79 w81 w97 w310 w514 w621 w711 w971 w993 w1012 w1016 w1033 w1042]
          tunnel: w67 -> [_ _ w92 w305 _ _ w704 w962 w994 w1013 w1017 w1023 w1044]
          frame "TimeOut", Default {
          }
          frame "Close_Program" {
          }
          frame "Measure_InSituSpinCoating" {
            w95 = T8 {"QueueAction"=enum."TimeOut", "Data"=[], "Data_Raw"=[], "Data_Dark"=[], "Data_Ref"=[], "Device Information"=[], "Numeric Control"=0.0, "Boolean"=FALSE, "Wavelength"=[], "Time"=[], "Time Stamp"=timestamp(0 s since 1904-01-01), "Numeric Control 2"=0.0, "TabControl"=enum."Measure", "Numeric Control 3"=0.0}  # DataQueue
            n58 = property on="Seconds to\nSpin Start" class="DigNum (strict)"() -> ("Value"=w89:dbl[unit])  [unwired: 2 in, 2 out]
            n59 = Unbundle By Name(w92) -> ("Time Stamp"=w91:timestamp)
            n60 = node(w89) -> (w88:dbl)
            n61 = Obtain Queue(name (unnamed)="Temp", element data type=w95) -> (queue out=w94:refnum<queue>)  [unwired: 3 in, 2 out]
            n62 = while {
              shift-right: [w110] -> w100
              shift-left: w98 -> [w119]
              shift-right: [w111] -> w99
              shift-left: w97 -> [w118]
              shift-right: [w112] -> w93
              shift-left: w94 -> [w113]
              tunnel: w91 -> [w106]
              shift-right: [w107] -> _
              shift-left: string[] [] ("Device Information") -> [w108]
              border: FALSE -> [_]
              tunnel: w88 -> [w103]
              shift-right: [w101] -> w87
              shift-left: w85 -> [w102]
              stop <- w109 stop-if-true
              n63 = Dequeue Element(queue=w119, error in (no error)=w118) -> (queue out=w114:refnum<queue>, element=w116:T8, error out=w115:errorcluster)  [unwired: 1 in, 1 out]
              n64 = Unbundle By Name(w116) -> ("QueueAction"=w117:T9)
              n65 = feedback #1() -> (w105:bool)
              n66 = case shown="\"Spectrometer_Measure\"" w117 {
                tunnel: w116 -> [w128 w138 _ w187 w205 w214 w246 w291]
                tunnel: w115 -> [w127 w139 w146 w184 w203 w212 w237 w288]
                tunnel: w114 -> [w123 w140 w145 w183 w204 w213 w245 w289]
                tunnel: w113 -> [w126 w135 w147 w178 w201 w210 w234 w292]
                tunnel: [w125 w135 w142 w175 w201 w210 w234 w292] -> w112
                tunnel: [w124 w136 w144 w174 w203 w212 w235 w288] -> w111
                tunnel: [w123 w137 w143 w173 w204 w213 w245 w289] -> w110
                tunnel: [_ TRUE TRUE TRUE _ _ _ _] -> w109
                tunnel: w108 -> [w122 w133 w154 w185 w202 w211 w232 _]
                tunnel: [w122 w133 w154 w185 w202 w211 w232 w290] -> w107
                tunnel: w106 -> [_ _ _ w186 _ _ w247 _]
                tunnel: w105 -> [w121 w132 w153 w172 w197 w206 w230 w287]
                tunnel: [w121 w132 w153 w172 w197 w206 TRUE w287] -> w104
                tunnel: w103 -> [_ _ _ w169 _ _ _ _]
                tunnel: w102 -> [w120 w129 w141 w164 w200 w209 w215 w286]
                tunnel: [w120 w129 w141 w164 w198 w207 w215 w286] -> w101
                frame Default {
                  n67 = Enqueue Element(queue=w126, element=w128, error in (no error)=w127) -> (queue out=w125:refnum<queue>, error out=w124:errorcluster)  [unwired: 1 in, 1 out]
                }
                frame "Close_Program" {
                  n68 = Enqueue Element At Opposite End(queue=w140, element=w138, error in (no error)=w139) -> (queue out=w137:refnum<queue>, error out=w136:errorcluster)  [unwired: 1 in, 1 out]
                  n69 = property on="Time.spin" class="Ref (strict)"() -> ("Value"=w130:refnum<file>)  [unwired: 2 in, 2 out]
                  n70 = property on="Meas.spin" class="Ref (strict)"() -> ("Value"=w131:refnum<file>)  [unwired: 2 in, 2 out]
                  n71 = Close File(refnum=w131) -> ()  [unwired: 1 in, 2 out]
                  n72 = Close File(refnum=w130) -> ()  [unwired: 1 in, 2 out]
                }
                frame "Abort" {
                  n73 = property on="Time.spin" class="Ref (strict)"() -> ("Value"=w151:refnum<file>)  [unwired: 2 in, 2 out]
                  n74 = Get Queue Status(queue=w147) -> (queue out=w148:refnum<queue>, # elements in queue=w149:i32)  [unwired: 2 in, 6 out]
                  n75 = property on="Meas.spin" class="Ref (strict)"() -> ("Value"=w152:refnum<file>)  [unwired: 2 in, 2 out]
                  n76 = Close File(refnum=w152) -> ()  [unwired: 1 in, 2 out]
                  n77 = Close File(refnum=w151) -> ()  [unwired: 1 in, 2 out]
                  n78 = for {
                    N: w149 -> [_]
                    shift-right: [w161] -> w142
                    shift-left: w148 -> [w162]
                    shift-right: [w158] -> w143
                    shift-left: w145 -> [w159]
                    shift-right: [w156] -> w144
                    shift-left: w146 -> [w157]
                    n79 = Dequeue Element(queue=w162) -> (queue out=w161:refnum<queue>, element=w160:T8)  [unwired: 2 in, 2 out]
                    n80 = Enqueue Element(queue=w159, element=w160, error in (no error)=w157) -> (queue out=w158:refnum<queue>, error out=w156:errorcluster)  [unwired: 1 in, 1 out]
                  }
                  n81 = property on="StartMeasurement_Button" class="Bool (strict)"("Value"=FALSE ("StartMeasurement_Button")) -> ()  [unwired: 2 in, 2 out]
                }
                frame "Stop_Measurement" {
                  n82 = property on="Automatically \nadjust count" class="Bool (strict)"() -> ("Value"=w166:bool)  [unwired: 2 in, 2 out]
                  n83 = property on="Reset Count\nafter Spin Coating" class="Bool (strict)"() -> ("Value"=w167:bool)  [unwired: 2 in, 2 out]
                  n84 = Or(x=w166, y=w167) -> (x .or. y?=w165:bool)
                  n85 = Bundle By Name(cluster=w187, "QueueAction"=DataQueue_Action."Save_InSitu", "Time Stamp"=w186, "Device Information"=w185, "Numeric Control"=w169, "Numeric Control 3"=0.0) -> (w182:T8)
                  n86 = case shown="True" w165 {
                    frame False {
                    }
                    frame True {
                      n87 = property on="Spectra \nCount" class="DigNum (strict)"("Value"=u16 0 ("Spectra Count")) -> ()  [unwired: 2 in, 2 out]
                    }
                  }
                  n88 = Enqueue Element(queue=w183, element=w182, error in (no error)=w184) -> (queue out=w180:refnum<queue>, error out=w179:errorcluster)  [unwired: 1 in, 1 out]
                  n89 = Get Queue Status(queue=w178) -> (queue out=w176:refnum<queue>, # elements in queue=w177:i32)  [unwired: 2 in, 6 out]
                  n90 = property on="Time.spin" class="Ref (strict)"() -> ("Value"=w170:refnum<file>)  [unwired: 2 in, 2 out]
                  n91 = property on="StartMeasurement_Button" class="Bool (strict)"("Value"=FALSE ("StartMeasurement_Button")) -> ()  [unwired: 2 in, 2 out]
                  n92 = property on="Meas.spin" class="Ref (strict)"() -> ("Value"=w171:refnum<file>)  [unwired: 2 in, 2 out]
                  n93 = for {
                    N: w177 -> [_]
                    shift-right: [w195] -> w175
                    shift-left: w176 -> [w196]
                    shift-right: [w192] -> w173
                    shift-left: w180 -> [w193]
                    shift-right: [w190] -> w174
                    shift-left: w179 -> [w191]
                    n94 = Dequeue Element(queue=w196) -> (queue out=w195:refnum<queue>, element=w194:T8)  [unwired: 2 in, 2 out]
                    n95 = Enqueue Element(queue=w193, element=w194, error in (no error)=w191) -> (queue out=w192:refnum<queue>, error out=w190:errorcluster)  [unwired: 1 in, 1 out]
                  }
                  n96 = Close File(refnum=w171) -> ()  [unwired: 1 in, 2 out]
                  n97 = Close File(refnum=w170) -> ()  [unwired: 1 in, 2 out]
                }
                frame "Set_Ref" {
                  n98 = Unbundle By Name(w205) -> ("Data_Ref"=w199:T14)
                  n99 = Bundle By Name(cluster=w200, "Ref"=w199) -> (w198:T5)
                }
                frame "Set_Dark" {
                  n100 = Unbundle By Name(w214) -> ("Data_Dark"=w208:T14)
                  n101 = Bundle By Name(cluster=w209, "Dark"=w208) -> (w207:T5)
                }
                frame "Spectrometer_Measure" {
                  w220 = FALSE ("prepend array or string size? (T)")
                  w233 = enum16{"start", "end", "current"}."end" ("from (0:start)")
                  n102 = Unbundle By Name(w246) -> ("Data_Raw"=w242:T14, "Time"=w236:dbl[])
                  n103 = property on="LowerWLLimit" class="DigNum (strict)"() -> ("Value"=w217:i32)  [unwired: 2 in, 2 out]
                  n104 = To Unsigned Long Integer(number=w236) -> (unsigned 32bit integer=w222:u32[])
                  n105 = Index Array(array=w242, index=0) -> (element=w241:T15)
                  n106 = Unbundle By Name(w241) -> ("Image"=w219:dbl[][][])
                  n107 = property on="UpperWLLimit" class="DigNum (strict)"() -> ("Value"=w216:i32)  [unwired: 2 in, 2 out]
                  n108 = call "Trim_Spectra.vi"("WL_UpperIndex"=w216, "WL_LowerIndex"=w217, "Image"=w219) -> ("ImageCut"=w218:dbl[][][])
                  n109 = case shown="False" w230 {
                    tunnel: w247 -> [w279 _]
                    tunnel: w237 -> [w275 w283]
                    tunnel: [w261 w283] -> w224
                    tunnel: [w249 _] -> w225
                    tunnel: [w260 w285] -> w227
                    tunnel: [w250 w284] -> w226
                    tunnel: w218 -> [w258 _]
                    frame False {
                      w270 = T13."open or create" ("operation (0:open)")
                      w269 = "_" ("string")
                      n110 = property on="fName_Temp" class="Str"() -> ("Value"=w248:string)  [unwired: 2 in, 2 out]
                      n111 = Concatenate Strings(w248, "_meas.spin" ("string")) -> (w280:string)
                      n112 = Concatenate Strings(w248, "_time.spin" ("string")) -> (w273:string)
                      n113 = Format Date/Time String(time format string (%c)="%Y%m%d_%H%M%S", seconds (now)=w279) -> (date/time string=w274:string)  [unwired: 1 in]
                      n114 = property on="Measure_SavePath" class="Path"() -> ("Value"=w252:path)  [unwired: 2 in, 2 out]
                      n115 = Concatenate Strings(w274, w269, w280) -> (w278:string)
                      n116 = Concatenate Strings(w274, w269, w273) -> (w272:string)
                      n117 = Build Path(base path=w252, name or relative path=w278) -> (appended path=w276:path)
                      n118 = Build Path(base path=w252, name or relative path=w272) -> (appended path=w271:path)
                      n119 = Array Size(array=w258) -> (size(s)=w257:i32[])
                      n120 = property on="Frames" class="DigNum (strict)"() -> ("Value"=w251:i32)  [unwired: 2 in, 2 out]
                      n121 = Open/Create/Replace File(file path (use dialog)=w276, error in=w275, operation (0:open)=w270) -> (refnum out=w268:refnum<file>, error out=w267:errorcluster)  [unwired: 3 in, 1 out]
                      "Meas.spin" <- w268
                      n122 = Open/Create/Replace File(file path (use dialog)=w271, error in=w275, operation (0:open)=w270) -> (refnum out=w266:refnum<file>, error out=w265:errorcluster)  [unwired: 3 in, 1 out]
                      n123 = Write to Binary File(file (use dialog)=w268, data=w251, error in=w267) -> (refnum out=w264:refnum<file>, error out=w263:errorcluster)  [unwired: 3 in, 1 out]
                      n124 = Index Array(array=w257, index #1=2 ("index"), index #2=1 ("index")) -> (element #1=w253:i32, element #2=w254:i32)
                      n125 = Write to Binary File(file (use dialog)=w266, data=w251, error in=w265) -> (refnum out=w250:refnum<file>, error out=w249:errorcluster)  [unwired: 3 in, 1 out]
                      "Time.spin" <- w250
                      n126 = Write to Binary File(file (use dialog)=w264, data=w254, error in=w263) -> (refnum out=w259:refnum<file>, error out=w262:errorcluster)  [unwired: 3 in, 1 out]
                      n127 = Write to Binary File(file (use dialog)=w259, data=w253, error in=w262) -> (refnum out=w260:refnum<file>, error out=w261:errorcluster)  [unwired: 3 in, 1 out]
                    }
                    frame True {
                      n128 = property on="Time.spin" class="Ref (strict)"() -> ("Value"=w284:refnum<file>)  [unwired: 2 in, 2 out]
                      n129 = property on="Meas.spin" class="Ref (strict)"() -> ("Value"=w285:refnum<file>)  [unwired: 2 in, 2 out]
                    }
                  }
                  n130 = To Unsigned Word Integer(number=w218) -> (unsigned 16bit integer=w221:u16[][][])
                  n131 = Merge Errors(w224, w225) -> (w223:errorcluster)
                  n132 = Set File Position(refnum=w227, from (0:start)=w233, error in=w223) -> (refnum out=w239:refnum<file>, error out=w238:errorcluster)  [unwired: 1 in]
                  n133 = Set File Position(refnum=w226, from (0:start)=w233, error in=w223) -> (refnum out=w244:refnum<file>, error out=w243:errorcluster)  [unwired: 1 in]
                  n134 = Write to Binary File(file (use dialog)=w244, data=w222, error in=w243, 5:w220) -> (error out=w228:errorcluster)  [unwired: 2 in, 2 out]
                  n135 = Write to Binary File(file (use dialog)=w239, data=w221, error in=w238, 5:w220) -> (error out=w229:errorcluster)  [unwired: 2 in, 2 out]
                  n136 = Merge Errors(w229, w228) -> (w235:errorcluster)
                }
                frame "Transfer_Settings" {
                  n137 = Unbundle By Name(w291) -> ("Device Information"=w290:string[])
                }
              }
              n138 = feedback-in #1(w104) -> ()
            }
            n139 = Release Queue(queue=w93) -> ()  [unwired: 2 in, 3 out]
          }
          frame "Measure_InSituSpinCoating_Short" {
            w308 = T8 {"QueueAction"=enum."TimeOut", "Data"=[], "Data_Raw"=[], "Data_Dark"=[], "Data_Ref"=[], "Device Information"=[], "Numeric Control"=0.0, "Boolean"=FALSE, "Wavelength"=[], "Time"=[], "Time Stamp"=timestamp(0 s since 1904-01-01), "Numeric Control 2"=0.0, "TabControl"=enum."Measure", "Numeric Control 3"=0.0}  # DataQueue
            n140 = property on="Seconds to\nSpin Start" class="DigNum (strict)"() -> ("Value"=w302:dbl[unit])  [unwired: 2 in, 2 out]
            n141 = Unbundle By Name(w305) -> ("Time Stamp"=w304:timestamp)
            n142 = node(w302) -> (w301:dbl)
            n143 = Obtain Queue(name (unnamed)="Temp", element data type=w308) -> (queue out=w307:refnum<queue>)  [unwired: 3 in, 2 out]
            n144 = Unbundle By Name(w298) -> ("Wavlength"=w296:dbl[unit][])
            n145 = Subtract(x=w296, y="Wavelenght Detect") -> (x-y=w297:dbl[unit][])
            n146 = Absolute Value(x=w297) -> (abs(x)=w295:dbl[unit][])
            n147 = Array Max & Min(array=w295) -> (min index (indices)=→"WL-Det\nPos":i32)  [unwired: 3 out]
            n148 = while {
              shift-right: [w323] -> w313
              shift-left: w311 -> [w332]
              shift-right: [w324] -> w312
              shift-left: w310 -> [w331]
              shift-right: [w325] -> w306
              shift-left: w307 -> [w326]
              tunnel: w304 -> [w319]
              shift-right: [w320] -> _
              shift-left: string[] [] ("Device Information") -> [w321]
              border: FALSE -> [_]
              tunnel: w301 -> [w316]
              shift-right: [w314] -> w300
              shift-left: w298 -> [w315]
              stop <- w322 stop-if-true
              n149 = Dequeue Element(queue=w332, error in (no error)=w331) -> (queue out=w327:refnum<queue>, element=w329:T8, error out=w328:errorcluster)  [unwired: 1 in, 1 out]
              n150 = Unbundle By Name(w329) -> ("QueueAction"=w330:T9)
              n151 = feedback #2() -> (w318:bool)
              n152 = case shown="\"Spectrometer_Measure\"" w330 {
                tunnel: w329 -> [w341 w351 _ w400 w418 w427 w459 w504]
                tunnel: w328 -> [w340 w352 w361 w397 w416 w425 w450 w501]
                tunnel: w327 -> [w336 w353 w360 w396 w417 w426 w458 w502]
                tunnel: w326 -> [w339 w348 w362 w391 w414 w423 w447 w505]
                tunnel: [w338 w348 w357 w388 w414 w423 w447 w505] -> w325
                tunnel: [w337 w349 w359 w387 w416 w425 w448 w501] -> w324
                tunnel: [w336 w350 w358 w386 w417 w426 w458 w502] -> w323
                tunnel: [_ TRUE TRUE TRUE _ _ _ _] -> w322
                tunnel: w321 -> [w335 w346 w367 w398 w415 w424 w445 _]
                tunnel: [w335 w346 w367 w398 w415 w424 w445 w503] -> w320
                tunnel: w319 -> [_ _ _ w399 _ _ w460 _]
                tunnel: w318 -> [w334 w345 w366 w385 w410 w419 w443 w500]
                tunnel: [w334 w345 w366 w385 w410 w419 TRUE w500] -> w317
                tunnel: w316 -> [_ _ _ w384 _ _ _ _]
                tunnel: w315 -> [w333 w344 w356 w379 w413 w422 w428 w499]
                tunnel: [w333 w344 w356 w379 w411 w420 w428 w499] -> w314
                frame Default {
                  n153 = Enqueue Element(queue=w339, element=w341, error in (no error)=w340) -> (queue out=w338:refnum<queue>, error out=w337:errorcluster)  [unwired: 1 in, 1 out]
                }
                frame "Close_Program" {
                  n154 = property on="Meas.spin" class="Ref (strict)"() -> ("Value"=w343:refnum<file>)  [unwired: 2 in, 2 out]
                  n155 = property on="Time.spin" class="Ref (strict)"() -> ("Value"=w342:refnum<file>)  [unwired: 2 in, 2 out]
                  n156 = Enqueue Element At Opposite End(queue=w353, element=w351, error in (no error)=w352) -> (queue out=w350:refnum<queue>, error out=w349:errorcluster)  [unwired: 1 in, 1 out]
                  n157 = Close File(refnum=w343) -> ()  [unwired: 1 in, 2 out]
                  n158 = Close File(refnum=w342) -> ()  [unwired: 1 in, 2 out]
                }
                frame "Abort" {
                  n159 = property on="Time.spin" class="Ref (strict)"() -> ("Value"=w354:refnum<file>)  [unwired: 2 in, 2 out]
                  n160 = property on="Meas.spin" class="Ref (strict)"() -> ("Value"=w355:refnum<file>)  [unwired: 2 in, 2 out]
                  n161 = Get Queue Status(queue=w362) -> (queue out=w363:refnum<queue>, # elements in queue=w364:i32)  [unwired: 2 in, 6 out]
                  n162 = Close File(refnum=w355) -> ()  [unwired: 1 in, 2 out]
                  n163 = Close File(refnum=w354) -> ()  [unwired: 1 in, 2 out]
                  n164 = for {
                    N: w364 -> [_]
                    shift-right: [w374] -> w357
                    shift-left: w363 -> [w375]
                    shift-right: [w371] -> w358
                    shift-left: w360 -> [w372]
                    shift-right: [w369] -> w359
                    shift-left: w361 -> [w370]
                    n165 = Dequeue Element(queue=w375) -> (queue out=w374:refnum<queue>, element=w373:T8)  [unwired: 2 in, 2 out]
                    n166 = Enqueue Element(queue=w372, element=w373, error in (no error)=w370) -> (queue out=w371:refnum<queue>, error out=w369:errorcluster)  [unwired: 1 in, 1 out]
                  }
                  n167 = property on="StartMeasurement_Button" class="Bool (strict)"("Value"=FALSE ("StartMeasurement_Button")) -> ()  [unwired: 2 in, 2 out]
                }
                frame "Stop_Measurement" {
                  n168 = property on="Automatically \nadjust count" class="Bool (strict)"() -> ("Value"=w381:bool)  [unwired: 2 in, 2 out]
                  n169 = property on="Reset Count\nafter Spin Coating" class="Bool (strict)"() -> ("Value"=w382:bool)  [unwired: 2 in, 2 out]
                  n170 = Or(x=w381, y=w382) -> (x .or. y?=w380:bool)
                  n171 = Bundle By Name(cluster=w400, "QueueAction"=DataQueue_Action."Save_InSitu", "Time Stamp"=w399, "Device Information"=w398, "Numeric Control"=w384, "Numeric Control 3"=1.0) -> (w395:T8)
                  n172 = case shown="True" w380 {
                    frame False {
                    }
                    frame True {
                      n173 = property on="Spectra \nCount" class="DigNum (strict)"("Value"=u16 0 ("Spectra Count")) -> ()  [unwired: 2 in, 2 out]
                    }
                  }
                  n174 = Enqueue Element(queue=w396, element=w395, error in (no error)=w397) -> (queue out=w393:refnum<queue>, error out=w392:errorcluster)  [unwired: 1 in, 1 out]
                  n175 = Get Queue Status(queue=w391) -> (queue out=w389:refnum<queue>, # elements in queue=w390:i32)  [unwired: 2 in, 6 out]
                  n176 = property on="StartMeasurement_Button" class="Bool (strict)"("Value"=FALSE ("StartMeasurement_Button")) -> ()  [unwired: 2 in, 2 out]
                  n177 = property on="Time.spin" class="Ref (strict)"() -> ("Value"=w377:refnum<file>)  [unwired: 2 in, 2 out]
                  n178 = property on="Meas.spin" class="Ref (strict)"() -> ("Value"=w378:refnum<file>)  [unwired: 2 in, 2 out]
                  n179 = for {
                    N: w390 -> [_]
                    shift-right: [w408] -> w388
                    shift-left: w389 -> [w409]
                    shift-right: [w405] -> w386
                    shift-left: w393 -> [w406]
                    shift-right: [w403] -> w387
                    shift-left: w392 -> [w404]
                    n180 = Dequeue Element(queue=w409) -> (queue out=w408:refnum<queue>, element=w407:T8)  [unwired: 2 in, 2 out]
                    n181 = Enqueue Element(queue=w406, element=w407, error in (no error)=w404) -> (queue out=w405:refnum<queue>, error out=w403:errorcluster)  [unwired: 1 in, 1 out]
                  }
                  n182 = Close File(refnum=w378) -> ()  [unwired: 1 in, 2 out]
                  n183 = Close File(refnum=w377) -> ()  [unwired: 1 in, 2 out]
                }
                frame "Set_Ref" {
                  n184 = Unbundle By Name(w418) -> ("Data_Ref"=w412:T14)
                  n185 = Bundle By Name(cluster=w413, "Ref"=w412) -> (w411:T5)
                }
                frame "Set_Dark" {
                  n186 = Unbundle By Name(w427) -> ("Data_Dark"=w421:T14)
                  n187 = Bundle By Name(cluster=w422, "Dark"=w421) -> (w420:T5)
                }
                frame "Spectrometer_Measure" {
                  w433 = FALSE ("prepend array or string size? (T)")
                  w446 = enum16{"start", "end", "current"}."end" ("from (0:start)")
                  n188 = Unbundle By Name(w459) -> ("Data_Raw"=w455:T14, "Time"=w449:dbl[])
                  n189 = property on="LowerWLLimit" class="DigNum (strict)"() -> ("Value"=w430:i32)  [unwired: 2 in, 2 out]
                  n190 = To Unsigned Long Integer(number=w449) -> (unsigned 32bit integer=w435:u32[])
                  n191 = Index Array(array=w455, index=0) -> (element=w454:T15)
                  n192 = Unbundle By Name(w454) -> ("Image"=w432:dbl[][][])
                  n193 = property on="UpperWLLimit" class="DigNum (strict)"() -> ("Value"=w429:i32)  [unwired: 2 in, 2 out]
                  n194 = call "Trim_Spectra.vi"("WL_UpperIndex"=w429, "WL_LowerIndex"=w430, "Image"=w432) -> ("ImageCut"=w431:dbl[][][])
                  n195 = case shown="False" w443 {
                    tunnel: w460 -> [w492 _]
                    tunnel: w450 -> [w488 w498]
                    tunnel: [w475 w498] -> w437
                    tunnel: [w464 _] -> w438
                    tunnel: [w474 w497] -> w440
                    tunnel: [w463 w496] -> w439
                    tunnel: w431 -> [w472 _]
                    frame False {
                      w483 = T13."open or create" ("operation (0:open)")
                      w482 = "_" ("string")
                      n196 = property on="fName_Temp" class="Str"() -> ("Value"=w461:string)  [unwired: 2 in, 2 out]
                      n197 = Concatenate Strings(w461, "_meas.spin" ("string")) -> (w493:string)
                      n198 = Concatenate Strings(w461, "_time.spin" ("string")) -> (w486:string)
                      n199 = Format Date/Time String(time format string (%c)="%Y%m%d_%H%M%S", seconds (now)=w492) -> (date/time string=w487:string)  [unwired: 1 in]
                      n200 = property on="Measure_SavePath" class="Path"() -> ("Value"=w466:path)  [unwired: 2 in, 2 out]
                      n201 = Concatenate Strings(w487, w482, w493) -> (w491:string)
                      n202 = Concatenate Strings(w487, w482, w486) -> (w485:string)
                      n203 = Build Path(base path=w466, name or relative path=w491) -> (appended path=w489:path)
                      n204 = Build Path(base path=w466, name or relative path=w485) -> (appended path=w484:path)
                      n205 = Array Size(array=w472) -> (size(s)=w471:i32[])
                      n206 = property on="Frames" class="DigNum (strict)"() -> ("Value"=w465:i32)  [unwired: 2 in, 2 out]
                      n207 = Open/Create/Replace File(file path (use dialog)=w489, error in=w488, operation (0:open)=w483) -> (refnum out=w462:refnum<file>, error out=w481:errorcluster)  [unwired: 3 in, 1 out]
                      n208 = Open/Create/Replace File(file path (use dialog)=w484, error in=w488, operation (0:open)=w483) -> (refnum out=w480:refnum<file>, error out=w479:errorcluster)  [unwired: 3 in, 1 out]
                      n209 = Write to Binary File(file (use dialog)=w462, data=w465, error in=w481) -> (refnum out=w478:refnum<file>, error out=w477:errorcluster)  [unwired: 3 in, 1 out]
                      n210 = Index Array(array=w471, index #1=2 ("index"), index #2=1 ("index")) -> (element #1=w467:i32, element #2=w468:i32)
                      n211 = Write to Binary File(file (use dialog)=w480, data=w465, error in=w479) -> (refnum out=w463:refnum<file>, error out=w464:errorcluster)  [unwired: 3 in, 1 out]
                      n212 = property on="Meas.spin" class="Ref (strict)"("Value"=w462) -> ()  [unwired: 2 in, 2 out]
                      n213 = Write to Binary File(file (use dialog)=w478, data=w468, error in=w477) -> (refnum out=w473:refnum<file>, error out=w476:errorcluster)  [unwired: 3 in, 1 out]
                      n214 = property on="Time.spin" class="Ref (strict)"("Value"=w463) -> ()  [unwired: 2 in, 2 out]
                      n215 = Write to Binary File(file (use dialog)=w473, data=w467, error in=w476) -> (refnum out=w474:refnum<file>, error out=w475:errorcluster)  [unwired: 3 in, 1 out]
                    }
                    frame True {
                      n216 = property on="Meas.spin" class="Ref (strict)"() -> ("Value"=w497:refnum<file>)  [unwired: 2 in, 2 out]
                      n217 = property on="Time.spin" class="Ref (strict)"() -> ("Value"=w496:refnum<file>)  [unwired: 2 in, 2 out]
                    }
                  }
                  n218 = To Unsigned Word Integer(number=w431) -> (unsigned 16bit integer=w434:u16[][][])
                  n219 = Merge Errors(w437, w438) -> (w436:errorcluster)
                  n220 = Set File Position(refnum=w440, from (0:start)=w446, error in=w436) -> (refnum out=w452:refnum<file>, error out=w451:errorcluster)  [unwired: 1 in]
                  n221 = Set File Position(refnum=w439, from (0:start)=w446, error in=w436) -> (refnum out=w457:refnum<file>, error out=w456:errorcluster)  [unwired: 1 in]
                  n222 = Write to Binary File(file (use dialog)=w457, data=w435, error in=w456, 5:w433) -> (error out=w441:errorcluster)  [unwired: 2 in, 2 out]
                  n223 = Write to Binary File(file (use dialog)=w452, data=w434, error in=w451, 5:w433) -> (error out=w442:errorcluster)  [unwired: 2 in, 2 out]
                  n224 = Merge Errors(w442, w441) -> (w448:errorcluster)
                }
                frame "Transfer_Settings" {
                  n225 = Unbundle By Name(w504) -> ("Device Information"=w503:string[])
                }
              }
              n226 = feedback-in #2(w317) -> ()
            }
            n227 = Release Queue(queue=w306) -> ()  [unwired: 2 in, 3 out]
          }
          frame "Measure_Spectrum" {
            w509 = T8 {"QueueAction"=enum."TimeOut", "Data"=[], "Data_Raw"=[], "Data_Dark"=[], "Data_Ref"=[], "Device Information"=[], "Numeric Control"=0.0, "Boolean"=FALSE, "Wavelength"=[], "Time"=[], "Time Stamp"=timestamp(0 s since 1904-01-01), "Numeric Control 2"=0.0, "TabControl"=enum."Measure", "Numeric Control 3"=0.0}  # DataQueue
            n228 = Obtain Queue(name (unnamed)="Temp", element data type=w509) -> (queue out=w508:refnum<queue>)  [unwired: 3 in, 2 out]
            n229 = while {
              shift-right: [w518] -> w512
              shift-left: w513 -> [w526]
              shift-right: [w519] -> w511
              shift-left: w514 -> [w527]
              shift-right: [w520] -> w507
              shift-left: w508 -> [w522]
              tunnel: w506 -> [w516]
              stop <- w517 stop-if-true
              n230 = Dequeue Element(queue=w526, error in (no error)=w527) -> (queue out=w524:refnum<queue>, element=w521:T8, error out=w523:errorcluster)  [unwired: 1 in, 1 out]
              n231 = Unbundle By Name(w521) -> ("QueueAction"=w525:T9, "TabControl"=w515:T10)
              n232 = case shown="\"Spectrometer_Measure\"" w525 {
                tunnel: w524 -> [w528 w560 w598]
                tunnel: w523 -> [w531 w568 w597]
                tunnel: w522 -> [w533 w574 w600]
                tunnel: w521 -> [w529 w550 _]
                tunnel: [w532 w574 w596] -> w520
                tunnel: [w530 w561 w594] -> w519
                tunnel: [w528 w560 w595] -> w518
                tunnel: [_ _ TRUE] -> w517
                tunnel: w516 -> [_ w553 _]
                tunnel: w515 -> [_ w548 w592]
                frame Default {
                  n233 = Enqueue Element(queue=w533, element=w529, error in (no error)=w531) -> (queue out=w532:refnum<queue>, error out=w530:errorcluster)  [unwired: 1 in, 1 out]
                }
                frame "Spectrometer_Measure" {
                  n234 = Unbundle By Name(w550) -> ("Data_Raw"=w567:T14)
                  n235 = case shown="\"Measure\", Default" w548 {
                    tunnel: [w587 "SpectralStability_SavePath"] -> w541
                    tunnel: [w586 "SpectralStability_FileName"] -> w539
                    tunnel: [w583 "SpectralStability_Comments"] -> w542
                    frame "Measure", Default {
                      n236 = property on="Spectra Count" class="DigNum (strict)"() -> ("Value"=w588:u16)  [unwired: 2 in, 2 out]
                      n237 = property on="Measure_SavePath" class="Path"() -> ("Value"=w587:path)  [unwired: 2 in, 2 out]
                      n238 = property on="Measure_Comments" class="Str"() -> ("Value"=w583:string)  [unwired: 2 in, 2 out]
                      n239 = property on="fName_Temp" class="Str"() -> ("Value"=w582:string)  [unwired: 2 in, 2 out]
                      n240 = Number To Decimal String(number=w588) -> (decimal integer string=w584:string)  [unwired: 1 in]
                      n241 = Concatenate Strings(w582, "_", w584) -> (w586:string)
                    }
                    frame "Spectral Stability" {
                    }
                  }
                  n242 = Index Array(array=w567, index=0) -> (element=w565:T15)
                  n243 = Unbundle By Name(w550) -> ("Time Stamp"=w549:timestamp)
                  n244 = Unbundle By Name(w565) -> ("Image"=w544:dbl[][][])
                  n245 = Index Array(array=w544, index (dim 1)=0 ("disabled index (row)")) -> (element=w559:dbl[][])  [unwired: 2 in]
                  n246 = Transpose 2D Array(2D array=w559) -> (transposed array=w556:dbl[][])
                  n247 = Format Date/Time String(time format string (%c)="%Y%m%d_%H%M%S", seconds (now)=w549) -> (date/time string=w572:string)  [unwired: 1 in]
                  n248 = Matrix Size(0:w556) -> (2:w557:i32)  [unwired: 1 out]
                  n249 = Empty String/Path?(string/path=w542) -> (empty?=w543:bool)
                  n250 = Reciprocal(x=w557) -> (1/x=w558:dbl)
                  n251 = Concatenate Strings(w572, "_") -> (w540:string)
                  n252 = case shown="False" w543 {
                    tunnel: w542 -> [w581 _]
                    tunnel: w541 -> [w580 _]
                    tunnel: w540 -> [w579 _]
                    tunnel: w539 -> [w578 _]
                    frame False {
                      n253 = Concatenate Strings(w579, w578, "_comments.txt" ("string")) -> (w575:string)
                      n254 = Build Path(base path=w580, name or relative path=w575) -> (appended path=w576:path)
                      n255 = Write to Text File(file (use dialog)=w576, text=w581) -> ()  [unwired: 2 in, 3 out]
                    }
                    frame True {
                    }
                  }
                  n256 = Initialize Array(w558, w557) -> (w555:dbl[])
                  n257 = Concatenate Strings(w540, w539, ".spectra" ("string")) -> (w546:string)
                  n258 = Unbundle By Name(w553) -> ("Wavlength"=w534:dbl[unit][])
                  n259 = call-poly <vilib>:"A x B.vi"("Vector"=w555, "A"=w556) -> ("A x Vector"=w545:dbl[])  [unwired: 1 out]
                  n260 = Build Path(base path=w541, name or relative path=w546) -> (appended path=w570:path)
                  n261 = Bundle("Wavlength"=w534, "A x Vector"=w545) -> (w552:T16)  [unwired: 1 in]
                  n262 = Open/Create/Replace File(file path (use dialog)=w570, error in=w568, operation (0:open)=T13."open or create") -> (refnum out=w535:refnum<file>, error out=w538:errorcluster)  [unwired: 3 in, 1 out]
                  n263 = Build Array(w552) -> (w551:T17)
                  n264 = property on="Measure_Graph" class="XYGraph (strict)"("Value"=w551) -> ()  [unwired: 2 in, 2 out]
                  n265 = Write to Binary File(file (use dialog)=w535, data=w534, error in=w538) -> (refnum out=w536:refnum<file>, error out=w537:errorcluster)  [unwired: 3 in, 1 out]
                  n266 = To Unsigned Word Integer(number=w544) -> (unsigned 16bit integer=w564:u16[][][])
                  n267 = Write to Binary File(file (use dialog)=w536, data=w564, error in=w537) -> (refnum out=w562:refnum<file>, error out=w563:errorcluster)  [unwired: 3 in, 1 out]
                  n268 = Close File(refnum=w562, error in=w563) -> (error out=w561:errorcluster)  [unwired: 1 out]
                }
                frame "Stop_Measurement" {
                  w593 = FALSE ("Measure Spectrum")
                  n269 = case shown="\"Measure\"" w592 {
                    frame Default {
                    }
                    frame "Measure" {
                      n270 = property on="Automatically \nadjust count" class="Bool (strict)"() -> ("Value"=w603:bool)  [unwired: 2 in, 2 out]
                      n271 = case shown="True" w603 {
                        frame False {
                        }
                        frame True {
                          n272 = Increment(x="Spectra Count") -> (x+1=w604:u16)
                          n273 = property on="Spectra Count" class="DigNum (strict)"("Value"=w604) -> ()  [unwired: 2 in, 2 out]
                        }
                      }
                    }
                  }
                  n274 = Get Queue Status(queue=w600) -> (queue out=w601:refnum<queue>, # elements in queue=w599:i32)  [unwired: 2 in, 6 out]
                  n275 = property on="SpectralStability_MeasureSpectrum" class="Bool (strict)"("Value"=w593) -> ()  [unwired: 2 in, 2 out]
                  n276 = property on="Measure_MeasureSpectrum" class="Bool (strict)"("Value"=w593) -> ()  [unwired: 2 in, 2 out]
                  n277 = for {
                    N: w599 -> [_]
                    shift-right: [w611] -> w596
                    shift-left: w601 -> [w612]
                    shift-right: [w608] -> w595
                    shift-left: w598 -> [w609]
                    shift-right: [w606] -> w594
                    shift-left: w597 -> [w607]
                    n278 = Dequeue Element(queue=w612) -> (queue out=w611:refnum<queue>, element=w610:T8)  [unwired: 2 in, 2 out]
                    n279 = Enqueue Element(queue=w609, element=w610, error in (no error)=w607) -> (queue out=w608:refnum<queue>, error out=w606:errorcluster)  [unwired: 1 in, 1 out]
                  }
                }
              }
            }
            n280 = Release Queue(queue=w507) -> ()  [unwired: 2 in, 3 out]
          }
          frame "Measure_SpectrumAdvanced" {
            w616 = T8 {"QueueAction"=enum."TimeOut", "Data"=[], "Data_Raw"=[], "Data_Dark"=[], "Data_Ref"=[], "Device Information"=[], "Numeric Control"=0.0, "Boolean"=FALSE, "Wavelength"=[], "Time"=[], "Time Stamp"=timestamp(0 s since 1904-01-01), "Numeric Control 2"=0.0, "TabControl"=enum."Measure", "Numeric Control 3"=0.0}  # DataQueue
            n281 = Obtain Queue(name (unnamed)="Temp", element data type=w616) -> (queue out=w615:refnum<queue>)  [unwired: 3 in, 2 out]
            n282 = while {
              shift-right: [w624] -> w619
              shift-left: w620 -> [w632]
              shift-right: [w625] -> w618
              shift-left: w621 -> [w633]
              shift-right: [w626] -> w614
              shift-left: w615 -> [w628]
              tunnel: w613 -> [w622]
              stop <- w623 stop-if-true
              n283 = Dequeue Element(queue=w632, error in (no error)=w633) -> (queue out=w630:refnum<queue>, element=w627:T8, error out=w629:errorcluster)  [unwired: 1 in, 1 out]
              n284 = Unbundle By Name(w627) -> ("QueueAction"=w631:T9)
              n285 = case shown="\"Spectrometer_Measure\"" w631 {
                tunnel: w630 -> [w634 w663 w686]
                tunnel: w629 -> [w637 w671 w685]
                tunnel: w628 -> [w639 w679 w688]
                tunnel: w627 -> [w635 w651 _]
                tunnel: [w638 w679 w684] -> w626
                tunnel: [w636 w664 w682] -> w625
                tunnel: [w634 w663 w683] -> w624
                tunnel: [_ _ TRUE] -> w623
                tunnel: w622 -> [_ w655 _]
                frame Default {
                  n286 = Enqueue Element(queue=w639, element=w635, error in (no error)=w637) -> (queue out=w638:refnum<queue>, error out=w636:errorcluster)  [unwired: 1 in, 1 out]
                }
                frame "Spectrometer_Measure" {
                  w676 = "_"
                  n287 = Unbundle By Name(w651) -> ("Time Stamp"=w650:timestamp)
                  n288 = property on="fName_Temp" class="Str"() -> ("Value"=w640:string)  [unwired: 2 in, 2 out]
                  n289 = property on="Nr After Spin" class="DigNum (strict)"() -> ("Value"=w649:u16)  [unwired: 2 in, 2 out]
                  n290 = Unbundle By Name(w655) -> ("Wavlength"=w641:dbl[unit][])
                  n291 = Number To Decimal String(number=w649) -> (decimal integer string=w647:string)  [unwired: 1 in]
                  n292 = Format Date/Time String(time format string (%c)="%Y%m%d_%H%M%S", seconds (now)=w650) -> (date/time string=w677:string)  [unwired: 1 in]
                  n293 = Concatenate Strings(w677, w676, w640, w676, "a" ("string"), w647, ".spectra" ("string")) -> (w675:string)
                  n294 = property on="Measure_SavePath" class="Path"() -> ("Value"=w674:path)  [unwired: 2 in, 2 out]
                  n295 = Build Path(base path=w674, name or relative path=w675) -> (appended path=w673:path)
                  n296 = Unbundle By Name(w651) -> ("Data_Raw"=w670:T14)
                  n297 = Open/Create/Replace File(file path (use dialog)=w673, error in=w671, operation (0:open)=T13."open or create") -> (refnum out=w642:refnum<file>, error out=w643:errorcluster)  [unwired: 3 in, 1 out]
                  n298 = Index Array(array=w670, index=0) -> (element=w668:T15)
                  n299 = Write to Binary File(file (use dialog)=w642, data=w641, error in=w643) -> (refnum out=w645:refnum<file>, error out=w644:errorcluster)  [unwired: 3 in, 1 out]
                  n300 = Unbundle By Name(w668) -> ("Image"=w656:dbl[][][])
                  n301 = Index Array(array=w656, index (dim 1)=0 ("disabled index (row)")) -> (element=w662:dbl[][])  [unwired: 2 in]
                  n302 = Transpose 2D Array(2D array=w662) -> (transposed array=w659:dbl[][])
                  n303 = Matrix Size(0:w659) -> (2:w660:i32)  [unwired: 1 out]
                  n304 = Reciprocal(x=w660) -> (1/x=w661:dbl)
                  n305 = To Unsigned Word Integer(number=w656) -> (unsigned 16bit integer=w667:u16[][][])
                  n306 = Initialize Array(w661, w660) -> (w658:dbl[])
                  n307 = Write to Binary File(file (use dialog)=w645, data=w667, error in=w644) -> (refnum out=w665:refnum<file>, error out=w666:errorcluster)  [unwired: 3 in, 1 out]
                  n308 = call-poly <vilib>:"A x B.vi"("Vector"=w658, "A"=w659) -> ("A x Vector"=w652:dbl[])  [unwired: 1 out]
                  n309 = Bundle("Wavlength"=w641, "A x Vector"=w652) -> (w654:T16)  [unwired: 1 in]
                  n310 = Build Array(w654) -> (w653:T17)
                  n311 = property on="Measure_Graph" class="XYGraph (strict)"("Value"=w653) -> ()  [unwired: 2 in, 2 out]
                  n312 = Close File(refnum=w665, error in=w666) -> (error out=w664:errorcluster)  [unwired: 1 out]
                }
                frame "Stop_Measurement" {
                  n313 = property on="Automatically \nadjust count" class="Bool (strict)"() -> ("Value"=w680:bool)  [unwired: 2 in, 2 out]
                  n314 = case shown="True" w680 {
                    frame False {
                    }
                    frame True {
                      n315 = property on="Nr After Spin" class="DigNum (strict)"() -> ("Value"=w692:u16)  [unwired: 2 in, 2 out]
                      n316 = Increment(x=w692) -> (x+1=w691:u16)
                      n317 = property on="Nr After Spin" class="DigNum (strict)"("Value"=w691) -> ()  [unwired: 2 in, 2 out]
                    }
                  }
                  n318 = Get Queue Status(queue=w688) -> (queue out=w689:refnum<queue>, # elements in queue=w687:i32)  [unwired: 2 in, 6 out]
                  n319 = property on="Measure_MeasureSpectrum" class="Bool (strict)"("Value"=FALSE ("Measure Spectrum")) -> ()  [unwired: 2 in, 2 out]
                  n320 = for {
                    N: w687 -> [_]
                    shift-right: [w698] -> w684
                    shift-left: w689 -> [w699]
                    shift-right: [w695] -> w683
                    shift-left: w686 -> [w696]
                    shift-right: [w693] -> w682
                    shift-left: w685 -> [w694]
                    n321 = Dequeue Element(queue=w699) -> (queue out=w698:refnum<queue>, element=w697:T8)  [unwired: 2 in, 2 out]
                    n322 = Enqueue Element(queue=w696, element=w697, error in (no error)=w694) -> (queue out=w695:refnum<queue>, error out=w693:errorcluster)  [unwired: 1 in, 1 out]
                  }
                }
              }
            }
            n323 = Release Queue(queue=w614) -> ()  [unwired: 2 in, 3 out]
          }
          frame "Measure_SpectralStability" {
            w715 = T8 {"QueueAction"=enum."TimeOut", "Data"=[], "Data_Raw"=[], "Data_Dark"=[], "Data_Ref"=[], "Device Information"=[], "Numeric Control"=0.0, "Boolean"=FALSE, "Wavelength"=[], "Time"=[], "Time Stamp"=timestamp(0 s since 1904-01-01), "Numeric Control 2"=0.0, "TabControl"=enum."Measure", "Numeric Control 3"=0.0}  # DataQueue
            n324 = Unbundle By Name(w704) -> ("Time Stamp"=w710:timestamp)
            n325 = Unbundle By Name(w704) -> ("Numeric Control"=w700:dbl)
            n326 = property on="SpectralStability\n_SavePath" class="Path"() -> ("Value"=w706:path)  [unwired: 2 in, 2 out]
            n327 = property on="SpectralStability\n_FileName" class="Str"() -> ("Value"=w705:string)  [unwired: 2 in, 2 out]
            n328 = Obtain Queue(name (unnamed)="Temp", element data type=w715) -> (queue out=w714:refnum<queue>)  [unwired: 3 in, 2 out]
            n329 = call "Num2Str_TrailingZero.vi"("Numeric Control"=w700) -> ("format string"=w703:string)  [unwired: 10 in]
            n330 = Format Date/Time String(time format string (%c)="%Y%m%d_%H%M%S", seconds (now)=w710) -> (date/time string=w707:string)  [unwired: 1 in]
            n331 = while {
              shift-right: [w720] -> w708
              shift-left: w717 -> [w720]
              shift-right: [w726] -> _
              shift-left: w714 -> [w728]
              border: 0 -> [_]
              shift-right: [w727] -> w701
              shift-left: w712 -> [w736]
              shift-right: [w725] -> w702
              shift-left: w711 -> [w735]
              tunnel: w707 -> [w723]
              tunnel: w706 -> [w722]
              tunnel: w705 -> [w721]
              tunnel: w703 -> [w719]
              tunnel: w700 -> [w718]
              stop <- w724 stop-if-true
              n332 = Dequeue Element(queue=w736, error in (no error)=w735) -> (queue out=w734:refnum<queue>, element=w732:T8, error out=w733:errorcluster)  [unwired: 1 in, 1 out]
              n333 = Unbundle By Name(w732) -> ("QueueAction"=w731:T9)
              n334 = feedback #3() -> (w729:i32)
              n335 = case shown="\"Spectrometer_Measure\"" w731 {
                tunnel: w734 -> [w740 w749 w755 w773 w856 w863]
                tunnel: w733 -> [w739 w746 w756 w774 _ w864]
                tunnel: w732 -> [w741 w745 _ _ w810 w895]
                tunnel: [w743 w751 w762 w780 w794 w896] -> w730
                tunnel: w729 -> [w743 w751 w762 w780 w854 w896]
                tunnel: w728 -> [w742 w750 w758 w776 w855 w873]
                tunnel: [w740 w748 w753 w771 w856 w863] -> w727
                tunnel: [w738 w750 w757 w775 w855 w873] -> w726
                tunnel: [w737 w747 w754 w772 w799 w864] -> w725
                tunnel: [_ TRUE TRUE TRUE _ _] -> w724
                tunnel: w723 -> [_ _ _ _ w852 w893]
                tunnel: w722 -> [_ _ _ _ w819 w861]
                tunnel: w721 -> [_ _ _ _ w851 w891]
                tunnel: w720 -> [_ _ _ _ w826 w890]
                tunnel: w719 -> [_ _ _ _ w853 _]
                tunnel: w718 -> [_ _ _ _ w795 _]
                frame Default {
                  n336 = Enqueue Element(queue=w742, element=w741, error in (no error)=w739) -> (queue out=w738:refnum<queue>, error out=w737:errorcluster)  [unwired: 1 in, 1 out]
                }
                frame "Close_Program" {
                  n337 = Enqueue Element At Opposite End(queue=w749, element=w745, error in (no error)=w746) -> (queue out=w748:refnum<queue>, error out=w747:errorcluster)  [unwired: 1 in, 1 out]
                }
                frame "Abort" {
                  n338 = Get Queue Status(queue=w758) -> (queue out=w760:refnum<queue>, # elements in queue=w761:i32)  [unwired: 2 in, 6 out]
                  n339 = for {
                    N: w761 -> [_]
                    shift-right: [w768] -> w757
                    shift-left: w760 -> [w769]
                    shift-right: [w765] -> w753
                    shift-left: w755 -> [w766]
                    shift-right: [w763] -> w754
                    shift-left: w756 -> [w764]
                    n340 = Dequeue Element(queue=w769) -> (queue out=w768:refnum<queue>, element=w767:T8)  [unwired: 2 in, 2 out]
                    n341 = Enqueue Element(queue=w766, element=w767, error in (no error)=w764) -> (queue out=w765:refnum<queue>, error out=w763:errorcluster)  [unwired: 1 in, 1 out]
                  }
                  n342 = property on="SpectralStability_Record" class="Bool (strict)"("Value"=FALSE ("SpectralStability_Record")) -> ()  [unwired: 2 in, 2 out]
                }
                frame "Stop_Measurement" {
                  n343 = Get Queue Status(queue=w776) -> (queue out=w778:refnum<queue>, # elements in queue=w779:i32)  [unwired: 2 in, 6 out]
                  n344 = for {
                    N: w779 -> [_]
                    shift-right: [w786] -> w775
                    shift-left: w778 -> [w787]
                    shift-right: [w783] -> w771
                    shift-left: w773 -> [w784]
                    shift-right: [w781] -> w772
                    shift-left: w774 -> [w782]
                    n345 = Dequeue Element(queue=w787) -> (queue out=w786:refnum<queue>, element=w785:T8)  [unwired: 2 in, 2 out]
                    n346 = Enqueue Element(queue=w784, element=w785, error in (no error)=w782) -> (queue out=w783:refnum<queue>, error out=w781:errorcluster)  [unwired: 1 in, 1 out]
                  }
                  n347 = property on="SpectralStability_Record" class="Bool (strict)"("Value"=FALSE ("SpectralStability_Record")) -> ()  [unwired: 2 in, 2 out]
                }
                frame "Spectrometer_Measure" {
                  w850 = "_"
                  n348 = Increment(x=w854) -> (x+1=w794:i32)
                  n349 = Unbundle By Name(w810) -> ("Numeric Control 2"=w809:dbl)
                  n350 = Unbundle By Name(w810) -> ("Data_Raw"=w848:T14)
                  n351 = Format Into String(format string=w853, w854) -> (resulting string=w808:string)  [unwired: 2 in, 1 out]
                  n352 = Concatenate Strings(w852, w850, w851, w850) -> (w821:string)
                  n353 = Unbundle By Name(w826) -> ("Wavlength"=w824:dbl[unit][])
                  n354 = Index Array(array=w848, index=0) -> (element=w846:T15)
                  n355 = Divide(x=w794, y=w795) -> (x/y=w798:dbl)
                  n356 = Concatenate Strings(w821, "s" ("string"), w808, ".smean" ("string")) -> (w830:string)
                  n357 = Concatenate Strings(w821, "raw" ("string"), w808, ".spectra" ("string")) -> (w838:string)
                  n358 = Unbundle By Name(w846) -> ("Image"=w834:dbl[][][])
                  n359 = Concatenate Strings(w821, "timing.txt" ("string")) -> (w818:string)
                  n360 = Subtract(x=w795, y=w794) -> (x-y=w790:dbl)
                  "SS_StepsLeft" <- w790
                  n361 = Number To Exponential String(number=w809, 1:FALSE ("use system decimal point (T)")) -> (E-format string=w806:string)  [unwired: 2 in]
                  n362 = Build Path(base path=w819, name or relative path=w830) -> (appended path=w827:path)
                  n363 = Build Path(base path=w819, name or relative path=w818) -> (appended path=w817:path)
                  n364 = Multiply(x=w798, y=100.0) -> (x*y=w797:dbl)
                  n365 = property on="SS:PeriodicTime" class="DigNum (strict)"() -> ("Value"=w792:dbl[unit])  [unwired: 2 in, 2 out]
                  n366 = Build Path(base path=w819, name or relative path=w838) -> (appended path=w835:path)
                  n367 = Index Array(array=w834, index (dim 1)=0 ("disabled index (row)")) -> (element=w845:dbl[][])  [unwired: 2 in]
                  n368 = To Unsigned Byte Integer(number=w797) -> (unsigned 8bit integer=→"Horizontal Progress Bar":u8)
                  n369 = To Unsigned Word Integer(number=w834) -> (unsigned 16bit integer=w833:u16[][][])
                  n370 = Open/Create/Replace File(file path (use dialog)=w817, operation (0:open)=T13."open or create") -> (refnum out=w815:refnum<file>, error out=w812:errorcluster)  [unwired: 4 in, 1 out]
                  n371 = Concatenate Strings(w808, "\t", w806, "\r\n") -> (w805:string)
                  n372 = Transpose 2D Array(2D array=w845) -> (transposed array=w842:dbl[][])
                  n373 = Write to Binary File(file (use dialog)=w835, data=w833) -> (refnum out=w831:refnum<file>, error out=w832:errorcluster)  [unwired: 4 in, 1 out]
                  n374 = Multiply(x=w792, y=w790) -> (x*y=→"SS_TimePrediction":dbl[unit])
                  n375 = Set File Position(refnum=w815, from (0:start)=enum16{"start", "end", "current"}."end", error in=w812) -> (refnum out=w813:refnum<file>, error out=w811:errorcluster)  [unwired: 1 in]
                  n376 = Matrix Size(0:w842) -> (2:w843:i32)  [unwired: 1 out]
                  n377 = Close File(refnum=w831, error in=w832) -> (error out=w802:errorcluster)  [unwired: 1 out]
                  n378 = Reciprocal(x=w843) -> (1/x=w844:dbl)
                  n379 = Write to Text File(file (use dialog)=w813, text=w805, error in=w811) -> (refnum out=w804:refnum<file>, error out=w803:errorcluster)  [unwired: 1 in, 1 out]
                  n380 = Initialize Array(w844, w843) -> (w841:dbl[])
                  n381 = call-poly <vilib>:"A x B.vi"("Vector"=w841, "A"=w842) -> ("A x Vector"=w823:dbl[])  [unwired: 1 out]
                  n382 = Bundle("Wavlength"=w824, "A x Vector"=w823) -> (w825:T16)  [unwired: 1 in]
                  n383 = Close File(refnum=w804, error in=w803) -> (error out=w800:errorcluster)  [unwired: 1 out]
                  n384 = Write to Binary File(file (use dialog)=w827, data=w823) -> (refnum out=w829:refnum<file>, error out=w828:errorcluster)  [unwired: 4 in, 1 out]
                  n385 = Build Array(w825) -> (w822:T17)
                  n386 = Close File(refnum=w829, error in=w828) -> (error out=w801:errorcluster)  [unwired: 1 out]
                  n387 = property on="SpectralStability:\nGraph" class="XYGraph (strict)"("Value"=w822) -> ()  [unwired: 2 in, 2 out]
                  n388 = Merge Errors(w802, w801, w800) -> (w799:errorcluster)
                }
                frame "Transfer_Settings" {
                  w866 = "\r\n"
                  w880 = 0.0
                  w886 = 0 ("index")
                  n389 = Unbundle By Name(w890) -> ("Dark"=w887:T14, "Ref"=w888:T14, "Wavlength"=w889:dbl[unit][])
                  n390 = Concatenate Strings(w893, "_", w891) -> (w879:string)
                  n391 = property on="SpectralStability_\nPeriodicTime" class="DigNum (strict)"() -> ("Value"=w872:dbl[unit])  [unwired: 2 in, 2 out]
                  n392 = Unbundle By Name(w895) -> ("Device Information"=w894:string[])
                  n393 = property on="SpectralStability_Duration" class="DigNum (strict)"() -> ("Value"=w871:dbl[unit])  [unwired: 2 in, 2 out]
                  n394 = Index Array(array=w887, index=w886) -> (element=w884:T15)
                  n395 = Index Array(array=w888, index=w886) -> (element=w885:T15)
                  n396 = Concatenate Strings(w879, "_add.spin" ("string")) -> (w876:string)
                  n397 = Concatenate Strings(w879, "_comments.txt" ("string")) -> (w862:string)
                  n398 = Unbundle By Name(w884) -> ("Image"=w858:dbl[][][])
                  n399 = Unbundle By Name(w885) -> ("Image"=w857:dbl[][][])
                  n400 = property on="SpectralStability_\nMeasurementNumber" class="DigNum (strict)"() -> ("Value"=w870:u32)  [unwired: 2 in, 2 out]
                  n401 = Build Path(base path=w861, name or relative path=w876) -> (appended path=w875:path)
                  n402 = Build Path(base path=w861, name or relative path=w862) -> (appended path=w860:path)
                  n403 = node(w889) -> (w881:dbl[])
                  n404 = property on="Duration/Times" class="Bool (strict)"() -> ("Value"=w869:bool)  [unwired: 2 in, 2 out]
                  n405 = To Unsigned Word Integer(number=w858) -> (unsigned 16bit integer=w883:u16[][][])
                  n406 = To Unsigned Word Integer(number=w857) -> (unsigned 16bit integer=w882:u16[][][])
                  n407 = call "DeviceInfo2Str.vi"("Device Information"=w894) -> ("String"=w868:string)  [unwired: 10 in]
                  n408 = property on="SpectralStability:\nComments" class="Str"() -> ("Value"=w865:string)  [unwired: 2 in, 2 out]
                  n409 = Bundle(w883, w882, w881, w880, w880) -> (w874:cluster{u16[][][], u16[][][], dbl[], dbl, dbl})  [unwired: 1 in]
                  n410 = call "String_SpectralStabilitySettings.vi"("Duration/Times"=w869, "Measurement Number"=w870, "Duration"=w871, "Periodic Time"=w872) -> ("String"=w867:string)  [unwired: 7 in]
                  n411 = Concatenate Strings(w868, w866, w867, w866, w865) -> (w859:string)
                  n412 = Write to Binary File(file (use dialog)=w875, data=w874) -> ()  [unwired: 4 in, 3 out]
                  n413 = Write to Text File(file (use dialog)=w860, text=w859) -> ()  [unwired: 2 in, 3 out]
                }
              }
              n414 = feedback-in #3(w730) -> ()
            }
          }
          frame "Save_InSitu" {
            w929 = "\r\n"
            n415 = Unbundle By Name(w962) -> ("Time Stamp"=w960:timestamp, "Device Information"=w952:string[], "Numeric Control"=w949:dbl, "Numeric Control 2"=w948:dbl, "Numeric Control 3"=w913:dbl)
            n416 = case shown="0, Default" w913 {
              tunnel: ["In-Situ Normal:\n" ("string") "In-Situ Short\n" ("string")] -> w912
              frame 0, Default {
              }
              frame 1 {
              }
            }
            n417 = Unbundle By Name(w950) -> ("Dark"=w968:T14, "Ref"=w966:T14, "Wavlength Trim"=w970:dbl[unit][])
            n418 = property on="Threshold" class="DigNum (strict)"() -> ("Value"=w914:dbl)  [unwired: 2 in, 2 out]
            n419 = node(w970) -> (w963:dbl[])
            n420 = property on="Frames" class="DigNum (strict)"() -> ("Value"=w937:i32)  [unwired: 2 in, 2 out]
            n421 = property on="Wavelenght Detect" class="DigNum (strict)"() -> ("Value"=w915:dbl[unit])  [unwired: 2 in, 2 out]
            n422 = call "DeviceInfo2Str.vi"("Device Information"=w952) -> ("String"=w951:string)  [unwired: 10 in]
            n423 = Number To Decimal String(number=w937) -> (decimal integer string=w936:string)  [unwired: 1 in]
            n424 = Index Array(array=w966, index=0) -> (element=w964:T15)
            n425 = property on="Time Detect" class="DigNum (strict)"() -> ("Value"=w916:dbl[unit])  [unwired: 2 in, 2 out]
            n426 = property on="LowerWLLimit" class="DigNum (strict)"() -> ("Value"=w925:i32)  [unwired: 2 in, 2 out]
            n427 = property on="fName_Temp" class="Str"() -> ("Value"=w911:string)  [unwired: 2 in, 2 out]
            n428 = Index Array(array=w968, index=0) -> (element=w965:T15)
            n429 = property on="Spin Time" class="DigNum (strict)"() -> ("Value"=w917:dbl[unit])  [unwired: 2 in, 2 out]
            n430 = property on="Seconds to Spin_Normal" class="DigNum (strict)"() -> ("Value"=w919:dbl[unit])  [unwired: 2 in, 2 out]
            n431 = Unbundle By Name(w965) -> ("Image"=w926:dbl[][][])
            n432 = Unbundle By Name(w964) -> ("Image"=w927:dbl[][][])
            n433 = property on="UpperWLLimit" class="DigNum (strict)"() -> ("Value"=w924:i32)  [unwired: 2 in, 2 out]
            n434 = Format Date/Time String(time format string (%c)="%Y%m%d_%H%M%S", seconds (now)=w960) -> (date/time string=w959:string)  [unwired: 1 in]
            n435 = property on="Seconds after Spin" class="DigNum (strict)"() -> ("Value"=w918:dbl[unit])  [unwired: 2 in, 2 out]
            n436 = property on="Program Spin Coater" class="Arr (strict)"() -> ("Value"=w935:T2)  [unwired: 2 in, 2 out]
            n437 = call "Trim_Spectra.vi"("WL_UpperIndex"=w924, "WL_LowerIndex"=w925, "Image"=w927) -> ("ImageCut"=w922:dbl[][][])
            n438 = call "Trim_Spectra.vi"("WL_UpperIndex"=w924, "WL_LowerIndex"=w925, "Image"=w926) -> ("ImageCut"=w923:dbl[][][])
            n439 = call "MeasurementSpin2String_v02.vi"("Program Spin Coater"=w935, "Seconds to Spin Start"=w919, "Seconds after Spin Stop"=w918, "Spin Time"=w917, "Time Detect"=w916, "Wavelength Detect"=w915, "Threshold"=w914) -> ("concatenated string"=w934:string)  [unwired: 8 in]
            n440 = To Unsigned Word Integer(number=w922) -> (unsigned 16bit integer=w939:u16[][][])
            n441 = To Unsigned Word Integer(number=w923) -> (unsigned 16bit integer=w940:u16[][][])
            n442 = property on="Cell" class="Str"() -> ("Value"=w910:string)  [unwired: 2 in, 2 out]
            n443 = property on="Duration after" class="DigNum (strict)"() -> ("Value"=w931:dbl[unit])  [unwired: 2 in, 2 out]
            n444 = property on="periodic time" class="DigNum (strict)"() -> ("Value"=w932:dbl[unit])  [unwired: 2 in, 2 out]
            n445 = property on="Spin at end" class="Bool (strict)"() -> ("Value"=w930:bool)  [unwired: 2 in, 2 out]
            n446 = Concatenate Strings(w959, "_" ("string"), w911) -> (w957:string)
            n447 = Match Pattern(string=w910, regular expression="[0-9]+") -> (before substring=w898:string, match substring=w908:string, after substring=w899:string)  [unwired: 1 in, 1 out]
            n448 = String Length(string=w908) -> (length=w907:i32)
            n449 = Decimal String To Number(string=w908) -> (number=w906:i32)  [unwired: 2 in, 1 out]
            n450 = call "AfterSpinOptions.vi"("Spin at end"=w930, "Duration after"=w931, "periodic time"=w932) -> ("concatenated string"=w933:string)  [unwired: 8 in]
            n451 = Number To Decimal String(number=w907) -> (decimal integer string=w904:string)  [unwired: 1 in]
            n452 = Increment(x=w906) -> (x+1=w905:i32)
            n453 = Concatenate Strings("%0" ("string"), w904, "d" ("string")) -> (w901:string)
            n454 = Concatenate Strings(w912, w951, w929, "Frames:\t" ("string"), w936, w929, w934, w929, w933, w929, "Comments:" ("string"), w929, "Measure_Comments") -> (w947:string)
            n455 = Format Value(format string=w901, value (0)=w905) -> (output string=w900:string)  [unwired: 1 in]
            n456 = Bundle(w940, w939, w963, "Numeric Control"=w949, "Numeric Control 2"=w948) -> (w943:T18)  [unwired: 1 in]
            n457 = property on="Measure_SavePath" class="Path"() -> ("Value"=w945:path)  [unwired: 2 in, 2 out]
            n458 = Concatenate Strings(w898, w900, w899) -> (w897:string)
            n459 = Concatenate Strings(w957, "_add.spin" ("string")) -> (w956:string)
            n460 = Concatenate Strings(w957, "_comments.txt" ("string")) -> (w955:string)
            n461 = property on="Cell" class="Str"("Value"=w897) -> ()  [unwired: 2 in, 2 out]
            n462 = Build Path(base path=w945, name or relative path=w956) -> (appended path=w944:path)
            n463 = Build Path(base path=w945, name or relative path=w955) -> (appended path=w954:path)
            n464 = Write to Text File(file (use dialog)=w954, text=w947) -> (error out=w942:errorcluster)  [unwired: 2 in, 2 out]
            n465 = Write to Binary File(file (use dialog)=w944, data=w943) -> (error out=w941:errorcluster)  [unwired: 4 in, 2 out]
            n466 = flat-sequence {
              tunnel: w942 -> [_]
              tunnel: w941 -> [_]
              frame #0 {
                n467 = property on="Action" class="Str"("Value"="" ("Action")) -> ()  [unwired: 2 in, 2 out]
              }
            }
            n468 = property on="Action" class="Str"("Value"="Saving" ("Action")) -> ()  [unwired: 2 in, 2 out]
          }
          frame "Set_Dark" {
            # "Averaging"
            n469 = Unbundle By Name(w987) -> ("Wavlength"=w986:dbl[unit][])
            n470 = Unbundle By Name(w994) -> ("Data_Dark"=w984:T14)
            n471 = Index Array(array=w984, index=0) -> (element=w989:T15)
            n472 = Unbundle By Name(w989) -> ("Image"=w983:dbl[][][])
            n473 = Index Array(array=w983, index (dim 1)=0 ("disabled index (row)")) -> (element=w981:dbl[][])  [unwired: 2 in]
            n474 = Transpose 2D Array(2D array=w981) -> (transposed array=w978:dbl[][])
            n475 = Matrix Size(0:w978) -> (2:w979:i32)  [unwired: 1 out]
            n476 = Reciprocal(x=w979) -> (1/x=w980:dbl)
            n477 = Initialize Array(w980, w979) -> (w977:dbl[])
            n478 = call-poly <vilib>:"A x B.vi"("Vector"=w977, "A"=w978) -> ("A x Vector"=w976:dbl[])  [unwired: 1 out]
            n479 = Bundle("Wavlength"=w986, "A x Vector"=w976) -> (w988:T16)  [unwired: 1 in]
            n480 = Build Array(w988) -> (w985:T17)
            n481 = property on="Measure_Graph" class="XYGraph (strict)"("Value"=w985) -> ()  [unwired: 2 in, 2 out]
            n482 = Bundle By Name(cluster=w987, "Dark"=w984) -> (w991:T5)
          }
          frame "Set_Ref" {
            # "Averaging"
            n483 = Unbundle By Name(w996) -> ("Wavlength"=w995:dbl[unit][])
            n484 = Unbundle By Name(w1013) -> ("Data_Ref"=w1000:T14)
            n485 = Index Array(array=w1000, index=0) -> (element=w1008:T15)
            n486 = Unbundle By Name(w1008) -> ("Image"=w1007:dbl[][][])
            n487 = Index Array(array=w1007, index (dim 1)=0 ("disabled index (row)")) -> (element=w1005:dbl[][])  [unwired: 2 in]
            n488 = Transpose 2D Array(2D array=w1005) -> (transposed array=w1002:dbl[][])
            n489 = Matrix Size(0:w1002) -> (2:w1003:i32)  [unwired: 1 out]
            n490 = Reciprocal(x=w1003) -> (1/x=w1004:dbl)
            n491 = Initialize Array(w1004, w1003) -> (w1001:dbl[])
            n492 = call-poly <vilib>:"A x B.vi"("Vector"=w1001, "A"=w1002) -> ("A x Vector"=w997:dbl[])  [unwired: 1 out]
            n493 = Bundle("Wavlength"=w995, "A x Vector"=w997) -> (w999:T16)  [unwired: 1 in]
            n494 = Build Array(w999) -> (w998:T17)
            n495 = Bundle By Name(cluster=w996, "Ref"=w1000) -> (w1010:T5)
            n496 = property on="Measure_Graph" class="XYGraph (strict)"("Value"=w998) -> ()  [unwired: 2 in, 2 out]
          }
          frame "Set_Wavelength" {
            n497 = Unbundle By Name(w1017) -> ("Wavelength"=w1020:dbl[unit][])
            n498 = Bundle By Name(cluster=w1019, "Wavlength"=w1020) -> (w1018:T5)
            n499 = property on="TrimSpec" class="Bool (strict)"() -> ("Value"=w1014:bool)  [unwired: 2 in, 2 out]
            n500 = property on="TrimSpec" class="Bool (strict)"("Val(Sgnl)"=w1014) -> ()  [unwired: 2 in, 2 out]
          }
          frame "Spectrometer_Preview" {
            w1027 = 0 ("index (page)")
            n501 = Unbundle By Name(w1023) -> ("Data_Raw"=w1031:T14)
            n502 = Unbundle By Name(w1032) -> ("Wavlength"=w1026:dbl[unit][])
            n503 = Unbundle By Name(w1023) -> ("TabControl"=w1022:T10)
            n504 = Index Array(array=w1031, index=0) -> (element=w1029:T15)
            n505 = Unbundle By Name(w1029) -> ("Image"=w1028:dbl[][][])
            n506 = Index Array(array=w1028, index (dim 0)=w1027, index (dim 1)=w1027) -> (element=w1025:dbl[])  [unwired: 1 in]
            n507 = Bundle("Wavlength"=w1026, "Image"=w1025) -> (w1024:cluster{"Wavlength":dbl[unit][], "Image":dbl[]})  [unwired: 1 in]
            n508 = Build Array(w1024) -> (w1021:T3)
            n509 = case shown="Default" w1022 {
              tunnel: w1021 -> [w1035 w1036 _]
              frame "Measure" {
                "Measure_Graph" <- w1035
              }
              frame "Spectral Stability" {
                "SpectralStability_Graph" <- w1036
              }
              frame Default {
              }
            }
          }
          frame "Change_TrimSettings" {
            n510 = Unbundle By Name(w1044) -> ("Boolean"=w1043:bool)
            n511 = case shown="True" w1043 {
              tunnel: w1039 -> [w1050 w1068]
              tunnel: w1044 -> [_ w1063]
              tunnel: [0 w1054] -> w1041
              tunnel: [w1048 w1055] -> w1040
              tunnel: [w1046 w1051] -> w1037
              frame False {
                n512 = Unbundle By Name(w1050) -> ("Wavlength"=w1046:dbl[unit][])
                n513 = Array Size(array=w1046) -> (size(s)=w1049:i32)
                n514 = Decrement(x=w1049) -> (x-1=w1048:i32)
              }
              frame True {
                n515 = Unbundle By Name(w1063) -> ("Numeric Control"=w1067:dbl, "Numeric Control 2"=w1061:dbl)
                n516 = Unbundle By Name(w1068) -> ("Wavlength"=w1056:dbl[unit][])
                n517 = node(w1067) -> (w1066:dbl[unit])
                n518 = node(w1061) -> (w1060:dbl[unit])
                n519 = Subtract(x=w1056, y=w1060) -> (x-y=w1059:dbl[unit][])
                n520 = Subtract(x=w1056, y=w1066) -> (x-y=w1065:dbl[unit][])
                n521 = Absolute Value(x=w1059) -> (abs(x)=w1058:dbl[unit][])
                n522 = Absolute Value(x=w1065) -> (abs(x)=w1064:dbl[unit][])
                n523 = Array Max & Min(array=w1058) -> (min index (indices)=w1055:i32)  [unwired: 3 out]
                n524 = Array Max & Min(array=w1064) -> (min index (indices)=w1054:i32)  [unwired: 3 out]
                n525 = Subtract(x=w1055, y=w1054) -> (x-y=w1053:i32)
                n526 = Index Array(array=w1056, index=w1055) -> (element=w1057:dbl[unit])
                n527 = Index Array(array=w1056, index=w1054) -> (element=w1062:dbl[unit])
                n528 = Increment(x=w1053) -> (x+1=w1052:i32)
                n529 = Array Subset(array=w1056, index=w1054, length=w1052) -> (w1051:dbl[unit][])
                n530 = property on="WlLow" class="DigNum (strict)"("Value"=w1062) -> ()  [unwired: 2 in, 2 out]
                n531 = property on="WlUp" class="DigNum (strict)"("Value"=w1057) -> ()  [unwired: 2 in, 2 out]
              }
            }
            "LowerWLLimit" <- w1041
            "UpperWLLimit" <- w1040
            n532 = Bundle By Name(cluster=w1039, "Wavlength Trim"=w1037) -> (w1038:T5)
          }
        }
      }
      frame Error {
        w1074 = T19 4 items=["no dialog", "OK message", "continue or stop message", "OK message + warnings", "continue/stop + warnings"] ("type of dialog (OK msg:1)")
        n533 = call <vilib>:"General Error Handler.vi"("type of dialog (OK msg:1)"=w1074, "error in (no error)"=w1071) -> ("error out"=w1073:errorcluster)  [unwired: 9 in, 4 out]
        n534 = call <vilib>:"Clear Errors.vi"("error in (no error)"=w1073) -> ("error out"=w1070:errorcluster)  [unwired: 5 in, 1 out]
      }
    }
  }
  n535 = while {
    shift-right: [w1078] -> _
    shift-left: w16 -> [w1076]
    shift-right: [w1081] -> _
    shift-left: w12 -> [w1082]
    shift-right: [w1079] -> _
    shift-left: w5 -> [w1080]
    tunnel: w2 -> [w1075]
    stop <- w1077 stop-if-true
    # "Producer"
    n536 = event shown="[1] \"Stop Button\": Value Change" {
      selector: _ -> [_ _ _ _ _ _ _ _ _ _ _ _ _ _ _ _ _ _ _ _ _ _ _ _ _ _ _ _ _ _ _ _ _]
      dyn-events: _ -> [_ _ _ _ _ _ _ _ _ _ _ _ _ _ _ _ _ _ _ _ _ _ _ _ _ _ _ _ _ _ _ _ _]
      timeout: -1 -> [_ _ _ _ _ _ _ _ _ _ _ _ _ _ _ _ _ _ _ _ _ _ _ _ _ _ _ _ _ _ _ _ _]
      tunnel: w1082 -> [w1085 w1102 w1110 w1123 w1138 w1155 w1160 w1175 w1179 w1188 w1200 w1215 w1239 w1243 w1246 w1250 w1259 w1309 w1314 w1358 w1371 w1396 w1405 w1414 w1422 w1428 w1446 w1473 w1490 w1496 w1511 w1552 w1558]
      tunnel: [w1085 w1099 w1109 w1123 w1138 w1155 w1160 w1175 w1179 w1188 w1200 w1215 w1239 w1243 w1246 w1250 w1259 w1309 w1314 w1358 w1370 w1396 w1405 w1414 w1422 w1428 w1444 w1471 w1490 w1496 w1511 w1551 w1558] -> w1081
      tunnel: w1080 -> [w1084 w1101 w1113 w1121 w1135 w1154 w1159 w1172 w1180 w1189 w1201 w1213 w1234 w1242 w1247 w1249 w1256 w1274 w1313 w1350 w1375 w1395 w1404 w1413 w1421 w1427 w1449 w1477 w1491 w1495 w1509 w1544 w1557]
      tunnel: [w1084 w1095 w1104 w1117 w1134 w1152 w1159 w1171 w1181 w1190 w1202 w1211 w1233 w1242 w1247 w1249 w1254 w1291 w1311 w1334 w1369 w1390 w1401 w1410 w1421 w1427 w1449 w1477 w1491 w1495 w1506 w1544 w1556] -> w1079
      tunnel: w1076 -> [w1086 w1103 w1114 w1122 w1137 w1156 w1161 w1174 w1183 w1192 w1204 w1214 w1236 w1244 w1245 w1251 w1257 w1297 w1315 w1351 w1377 w1397 w1406 w1415 w1423 w1429 w1442 w1478 w1489 w1497 w1510 w1555 w1560]
      tunnel: [w1086 w1100 w1112 w1118 w1136 w1153 w1161 w1173 w1182 w1191 w1203 w1212 w1235 w1244 w1245 w1251 w1258 w1290 w1312 w1333 w1376 w1391 w1402 w1411 w1423 w1426 w1437 w1476 w1489 w1497 w1507 w1555 w1559] -> w1078
      tunnel: [_ TRUE _ _ _ _ _ _ _ _ _ _ _ _ _ _ _ _ _ _ _ _ _ _ _ _ _ _ _ _ _ _ _] -> w1077
      tunnel: w1075 -> [_ w1088 _ _ _ _ _ _ _ _ _ _ _ _ _ _ _ _ _ _ _ _ _ _ _ _ _ _ _ _ _ _ _]
      event Timeout {
        n537 = event-data() -> ()  [unwired: 1 in, 3 out]
      }
      event "Stop Button": Value Change {
        w1091 = T8 {"QueueAction"=enum."TimeOut", "Data"=[], "Data_Raw"=[], "Data_Dark"=[], "Data_Ref"=[], "Device Information"=[], "Numeric Control"=0.0, "Boolean"=FALSE, "Wavelength"=[], "Time"=[], "Time Stamp"=timestamp(0 s since 1904-01-01), "Numeric Control 2"=0.0, "TabControl"=enum."Measure", "Numeric Control 3"=0.0}  # DataQueue
        w1094 = T11 {"QueueAction"=enum."TimeOut", "Numeric 1"=0.0, "Numeric 2"=0.0, "Boolean 1"=FALSE, "Boolean 2"=FALSE, "Spin Program"=[], "Spin Prg v07"=[], "Time Stamp"=timestamp(0 s since 1904-01-01), "TabControl"=enum."Measure"}  # Device Queue
        n538 = event-data() -> ()  [unwired: 1 in, 6 out]
        n539 = Generate User Event(user event=w1088, event data cluster=TRUE ("event data")) -> ()  [unwired: 2 in, 2 out]
        n540 = Bundle By Name(cluster=w1094, "QueueAction"=DeviceQueue_Action."Close_Program") -> (w1092:T11)
        n541 = Enqueue Element At Opposite End(queue=w1103, element=w1092, error in (no error)=w1101) -> (queue out=w1100:refnum<queue>, error out=w1096:errorcluster)  [unwired: 1 in, 1 out]
        n542 = Bundle By Name(cluster=w1091, "QueueAction"=DataQueue_Action."Close_Program") -> (w1089:T8)
        n543 = Enqueue Element At Opposite End(queue=w1102, element=w1089, error in (no error)=w1101) -> (queue out=w1099:refnum<queue>, error out=w1097:errorcluster)  [unwired: 1 in, 1 out]
        n544 = Merge Errors(w1097, w1096) -> (w1095:errorcluster)
      }
      event "Abort Button": Value Change {
        w1108 = T8 {"QueueAction"=enum."TimeOut", "Data"=[], "Data_Raw"=[], "Data_Dark"=[], "Data_Ref"=[], "Device Information"=[], "Numeric Control"=0.0, "Boolean"=FALSE, "Wavelength"=[], "Time"=[], "Time Stamp"=timestamp(0 s since 1904-01-01), "Numeric Control 2"=0.0, "TabControl"=enum."Measure", "Numeric Control 3"=0.0}  # DataQueue
        w1116 = T11 {"QueueAction"=enum."TimeOut", "Numeric 1"=0.0, "Numeric 2"=0.0, "Boolean 1"=FALSE, "Boolean 2"=FALSE, "Spin Program"=[], "Spin Prg v07"=[], "Time Stamp"=timestamp(0 s since 1904-01-01), "TabControl"=enum."Measure"}  # Device Queue
        n545 = event-data() -> ()  [unwired: 1 in, 6 out]
        n546 = Bundle By Name(cluster=w1116, "QueueAction"=DeviceQueue_Action."Abort") -> (w1115:T11)
        n547 = Bundle By Name(cluster=w1108, "QueueAction"=DataQueue_Action."Abort") -> (w1106:T8)
        n548 = Enqueue Element At Opposite End(queue=w1114, element=w1115, error in (no error)=w1113) -> (queue out=w1112:refnum<queue>, error out=w1105:errorcluster)  [unwired: 1 in, 1 out]
        n549 = Enqueue Element At Opposite End(queue=w1110, element=w1106, error in (no error)=w1105) -> (queue out=w1109:refnum<queue>, error out=w1104:errorcluster)  [unwired: 1 in, 1 out]
      }
      event "Init_Spectrometer": Value Change {
        n550 = event-data() -> ()  [unwired: 1 in, 6 out]
        n551 = case shown="False" "Init_Spectrometer" {
          tunnel: [w1125 w1128] -> w1119
          frame True {
            n552 = property on="Tab Control" class="TabCtl (strict)"() -> ("Value"=w1124:T1)  [unwired: 2 in, 2 out]
            n553 = Bundle By Name(cluster=T11 {"QueueAction"=enum."TimeOut", "Numeric 1"=0.0, "Numeric 2"=0.0, "Boolean 1"=FALSE, "Boolean 2"=FALSE, "Spin Program"=[], "Spin Prg v07"=[], "Time Stamp"=timestamp(0 s since 1904-01-01), "TabControl"=enum."Measure"} ("element"), "QueueAction"=DeviceQueue_Action."Spectrometer_Init", "TabControl"=w1124) -> (w1125:T11)
          }
          frame False {
            n554 = Bundle By Name(cluster=T11 {"QueueAction"=enum."TimeOut", "Numeric 1"=0.0, "Numeric 2"=0.0, "Boolean 1"=FALSE, "Boolean 2"=FALSE, "Spin Program"=[], "Spin Prg v07"=[], "Time Stamp"=timestamp(0 s since 1904-01-01), "TabControl"=enum."Measure"} ("element"), "QueueAction"=DeviceQueue_Action."Spectrometer_Close") -> (w1128:T11)
          }
        }
        n555 = Enqueue Element(queue=w1122, element=w1119, error in (no error)=w1121) -> (queue out=w1118:refnum<queue>, error out=w1117:errorcluster)  [unwired: 1 in, 1 out]
      }
      event "Init_Arduino": Value Change {
        # "Shutter is closed after init"
        n556 = event-data() -> ("NewVal"=w1133:bool)  [unwired: 1 in, 5 out]
        n557 = case shown="True" w1133 {
          tunnel: [w1139 w1142] -> w1132
          frame False {
            w1141 = T11 {"QueueAction"=enum."TimeOut", "Numeric 1"=0.0, "Numeric 2"=0.0, "Boolean 1"=FALSE, "Boolean 2"=FALSE, "Spin Program"=[], "Spin Prg v07"=[], "Time Stamp"=timestamp(0 s since 1904-01-01), "TabControl"=enum."Measure"}  # Device Queue
            n558 = Bundle By Name(cluster=w1141, "QueueAction"=DeviceQueue_Action."Arduino_Close") -> (w1139:T11)
          }
          frame True {
            w1144 = T11 {"QueueAction"=enum."TimeOut", "Numeric 1"=0.0, "Numeric 2"=0.0, "Boolean 1"=FALSE, "Boolean 2"=FALSE, "Spin Program"=[], "Spin Prg v07"=[], "Time Stamp"=timestamp(0 s since 1904-01-01), "TabControl"=enum."Measure"}  # Device Queue
            n559 = Bundle By Name(cluster=w1144, "QueueAction"=DeviceQueue_Action."Arduino_Init") -> (w1142:T11)
          }
        }
        n560 = property on="Shutter Toggle" class="Bool (strict)"("Value"=FALSE ("Shutter Toggle")) -> ()  [unwired: 2 in, 2 out]
        n561 = Enqueue Element(queue=w1137, element=w1132, error in (no error)=w1135) -> (queue out=w1136:refnum<queue>, error out=w1134:errorcluster)  [unwired: 1 in, 1 out]
      }
      event "Program Spin Coater": Value Change {
        w1158 = T11 {"QueueAction"=enum."TimeOut", "Numeric 1"=0.0, "Numeric 2"=0.0, "Boolean 1"=FALSE, "Boolean 2"=FALSE, "Spin Program"=[], "Spin Prg v07"=[], "Time Stamp"=timestamp(0 s since 1904-01-01), "TabControl"=enum."Measure"}  # Device Queue
        n562 = event-data() -> ("NewVal"=w1147:T2)  [unwired: 1 in, 5 out]
        n563 = property on="Seconds to Spin_Normal" class="DigNum (strict)"() -> ("Value"=w1149:dbl[unit])  [unwired: 2 in, 2 out]
        n564 = property on="Spin Time" class="DigNum (strict)"() -> ("Value"=w1146:dbl[unit])  [unwired: 2 in, 2 out]
        n565 = node(w1146) -> (w1145:dbl)
        n566 = node(w1149) -> (w1148:dbl)
        n567 = Bundle By Name(cluster=w1158, "QueueAction"=DeviceQueue_Action."Arduino_LoadProgram", "Spin Prg v07"=w1147, "Numeric 1"=w1148, "Numeric 2"=w1145) -> (w1157:T11)
        n568 = Enqueue Element(queue=w1156, element=w1157, error in (no error)=w1154) -> (queue out=w1153:refnum<queue>, error out=w1152:errorcluster)  [unwired: 1 in, 1 out]
        n569 = property on="Measure_IntegrationTime" class="DigNum (strict)"() -> ("Value"=w1150:dbl[unit])  [unwired: 2 in, 2 out]
        n570 = property on="Measure_IntegrationTime" class="DigNum (strict)"("Val(Sgnl)"=w1150) -> ()  [unwired: 2 in, 2 out]
      }
      event "SHUTTER DEBUG": Value Change {
        n571 = event-data() -> ("NewVal"=w1163:bool)  [unwired: 1 in, 5 out]
        n572 = Select(t=u8 0, s=w1163, f=u8 2) -> (s? t:f=w1162:u8)
        n573 = property on="Shutter Position" class="DigNum (strict)"("DisabledEnum"=w1162) -> ()  [unwired: 2 in, 2 out]
        n574 = property on="Shutter Close" class="Bool (strict)"("DisabledEnum"=w1162) -> ()  [unwired: 2 in, 2 out]
        n575 = property on="Shutter Open" class="Bool (strict)"("DisabledEnum"=w1162) -> ()  [unwired: 2 in, 2 out]
      }
      event "Shutter Position": Value Change {
        w1170 = FALSE ("Shutter Close")
        w1168 = T11 {"QueueAction"=enum."TimeOut", "Numeric 1"=0.0, "Numeric 2"=0.0, "Boolean 1"=FALSE, "Boolean 2"=FALSE, "Spin Program"=[], "Spin Prg v07"=[], "Time Stamp"=timestamp(0 s since 1904-01-01), "TabControl"=enum."Measure"}  # Device Queue
        (unwired) DeviceQueue_Action."Arduino_SetSpeed" ("QueueAction")
        (unwired) T11 {"QueueAction"=enum."TimeOut", "Numeric 1"=0.0, "Numeric 2"=0.0, "Boolean 1"=FALSE, "Boolean 2"=FALSE, "Spin Program"=[], "Spin Prg v07"=[], "Time Stamp"=timestamp(0 s since 1904-01-01), "TabControl"=enum."Measure"}  # Device Queue
        n576 = event-data() -> ("NewVal"=w1166:u16)  [unwired: 1 in, 5 out]
        n577 = property on="Shutter Close" class="Bool (strict)"("Value"=w1170) -> ()  [unwired: 2 in, 2 out]
        n578 = property on="Shutter Open" class="Bool (strict)"("Value"=w1170) -> ()  [unwired: 2 in, 2 out]
        n579 = Bundle By Name(cluster=w1168, "QueueAction"=DeviceQueue_Action."Arduino_Shutter_SetPosition", "Numeric 1"=w1166) -> (w1169:T11)
        n580 = Enqueue Element(queue=w1174, element=w1169, error in (no error)=w1172) -> (queue out=w1173:refnum<queue>, error out=w1171:errorcluster)  [unwired: 1 in, 1 out]
      }
      event "Shutter Close": Value Change {
        w1178 = T11 {"QueueAction"=enum."TimeOut", "Numeric 1"=0.0, "Numeric 2"=0.0, "Boolean 1"=FALSE, "Boolean 2"=FALSE, "Spin Program"=[], "Spin Prg v07"=[], "Time Stamp"=timestamp(0 s since 1904-01-01), "TabControl"=enum."Measure"}  # Device Queue
        (unwired) DeviceQueue_Action."Arduino_SetSpeed" ("QueueAction")
        (unwired) T11 {"QueueAction"=enum."TimeOut", "Numeric 1"=0.0, "Numeric 2"=0.0, "Boolean 1"=FALSE, "Boolean 2"=FALSE, "Spin Program"=[], "Spin Prg v07"=[], "Time Stamp"=timestamp(0 s since 1904-01-01), "TabControl"=enum."Measure"}  # Device Queue
        n581 = event-data() -> ()  [unwired: 1 in, 6 out]
        n582 = property on="Shutter Open" class="Bool (strict)"("Value"=FALSE ("Shutter Open")) -> ()  [unwired: 2 in, 2 out]
        n583 = Bundle By Name(cluster=w1178, "QueueAction"=DeviceQueue_Action."Arduino_Shutter_Close") -> (w1177:T11)
        n584 = Enqueue Element(queue=w1183, element=w1177, error in (no error)=w1180) -> (queue out=w1182:refnum<queue>, error out=w1181:errorcluster)  [unwired: 1 in, 1 out]
      }
      event "Shutter Open": Value Change {
        w1187 = T11 {"QueueAction"=enum."TimeOut", "Numeric 1"=0.0, "Numeric 2"=0.0, "Boolean 1"=FALSE, "Boolean 2"=FALSE, "Spin Program"=[], "Spin Prg v07"=[], "Time Stamp"=timestamp(0 s since 1904-01-01), "TabControl"=enum."Measure"}  # Device Queue
        (unwired) DeviceQueue_Action."Arduino_SetSpeed" ("QueueAction")
        (unwired) T11 {"QueueAction"=enum."TimeOut", "Numeric 1"=0.0, "Numeric 2"=0.0, "Boolean 1"=FALSE, "Boolean 2"=FALSE, "Spin Program"=[], "Spin Prg v07"=[], "Time Stamp"=timestamp(0 s since 1904-01-01), "TabControl"=enum."Measure"}  # Device Queue
        n585 = event-data() -> ()  [unwired: 1 in, 6 out]
        n586 = property on="Shutter Close" class="Bool (strict)"("Value"=FALSE ("Shutter Open")) -> ()  [unwired: 2 in, 2 out]
        n587 = Bundle By Name(cluster=w1187, "QueueAction"=DeviceQueue_Action."Arduino_Shutter_Open") -> (w1186:T11)
        n588 = Enqueue Element(queue=w1192, element=w1186, error in (no error)=w1189) -> (queue out=w1191:refnum<queue>, error out=w1190:errorcluster)  [unwired: 1 in, 1 out]
      }
      event "Shutter Toggle": Value Change {
        w1199 = T11 {"QueueAction"=enum."TimeOut", "Numeric 1"=0.0, "Numeric 2"=0.0, "Boolean 1"=FALSE, "Boolean 2"=FALSE, "Spin Program"=[], "Spin Prg v07"=[], "Time Stamp"=timestamp(0 s since 1904-01-01), "TabControl"=enum."Measure"}  # Device Queue
        (unwired) T11 {"QueueAction"=enum."TimeOut", "Numeric 1"=0.0, "Numeric 2"=0.0, "Boolean 1"=FALSE, "Boolean 2"=FALSE, "Spin Program"=[], "Spin Prg v07"=[], "Time Stamp"=timestamp(0 s since 1904-01-01), "TabControl"=enum."Measure"}  # Device Queue
        n589 = event-data() -> ("NewVal"=w1197:bool)  [unwired: 1 in, 5 out]
        n590 = Select(t=DeviceQueue_Action."Arduino_Shutter_Open" ("QueueAction"), s=w1197, f=DeviceQueue_Action."Arduino_Shutter_Close" ("QueueAction")) -> (s? t:f=w1194:T12)
        n591 = Bundle By Name(cluster=w1199, "QueueAction"=w1194) -> (w1198:T11)
        n592 = Enqueue Element(queue=w1204, element=w1198, error in (no error)=w1201) -> (queue out=w1203:refnum<queue>, error out=w1202:errorcluster)  [unwired: 1 in, 1 out]
      }
      event "Measure_IntegrationTime", "SpectralStability_IntegrationTime": Value Change {
        w1217 = T11 {"QueueAction"=enum."TimeOut", "Numeric 1"=0.0, "Numeric 2"=0.0, "Boolean 1"=FALSE, "Boolean 2"=FALSE, "Spin Program"=[], "Spin Prg v07"=[], "Time Stamp"=timestamp(0 s since 1904-01-01), "TabControl"=enum."Measure"}  # Device Queue
        n593 = event-data() -> ("NewVal"=w1209:dbl[unit])  [unwired: 1 in, 5 out]
        n594 = property on="Calculate Frames_Normal" class="Bool (strict)"() -> ("Value"=w1205:bool)  [unwired: 2 in, 2 out]
        n595 = node(w1209) -> (w1208:dbl)
        n596 = property on="Tab Control" class="TabCtl (strict)"() -> ("Value"=w1207:T1)  [unwired: 2 in, 2 out]
        n597 = property on="Tab Control" class="TabCtl (strict)"() -> ("Value"=w1206:T1)  [unwired: 2 in, 2 out]
        n598 = case shown="\"Measure\"" w1207 {
          tunnel: w1217 -> [w1218 w1224 w1230]
          tunnel: [w1218 w1221 w1227] -> w1216
          tunnel: DeviceQueue_Action."Spectrometer_SetIntegrationTime" ("QueueAction") -> [_ w1223 w1229]
          tunnel: w1208 -> [_ w1222 w1228]
          tunnel: w1206 -> [_ w1220 w1225]
          tunnel: w1205 -> [_ w1219 _]
          frame Default {
          }
          frame "Measure" {
            n599 = Bundle By Name(cluster=w1224, "QueueAction"=w1223, "Numeric 1"=w1222, "Boolean 1"=w1219, "TabControl"=w1220) -> (w1221:T11)
          }
          frame "Spectral Stability" {
            n600 = Bundle By Name(cluster=w1230, "QueueAction"=w1229, "Numeric 1"=w1228, "Boolean 1"=FALSE, "TabControl"=w1225) -> (w1227:T11)
          }
        }
        n601 = Enqueue Element(queue=w1214, element=w1216, error in (no error)=w1213) -> (queue out=w1212:refnum<queue>, error out=w1211:errorcluster)  [unwired: 1 in, 1 out]
      }
      event "Frames": Value Change {
        w1238 = T11 {"QueueAction"=enum."TimeOut", "Numeric 1"=0.0, "Numeric 2"=0.0, "Boolean 1"=FALSE, "Boolean 2"=FALSE, "Spin Program"=[], "Spin Prg v07"=[], "Time Stamp"=timestamp(0 s since 1904-01-01), "TabControl"=enum."Measure"}  # Device Queue
        n602 = event-data() -> ()  [unwired: 1 in, 6 out]
        n603 = Bundle By Name(cluster=w1238, "QueueAction"=DeviceQueue_Action."Spectrometer_SetFrames", "Numeric 1"="Frames") -> (w1237:T11)
        n604 = Enqueue Element(queue=w1236, element=w1237, error in (no error)=w1234) -> (queue out=w1235:refnum<queue>, error out=w1233:errorcluster)  [unwired: 1 in, 1 out]
      }
      event "Seconds to Spin_Normal", "Seconds to Spin_Short": Value Change {
        n605 = event-data() -> ("NewVal"=w1240:dbl[unit])  [unwired: 1 in, 5 out]
        n606 = property on="Seconds to Spin_Short" class="DigNum (strict)"("Value"=w1240) -> ()  [unwired: 2 in, 2 out]
        n607 = property on="Seconds to Spin_Normal" class="DigNum (strict)"("Value"=w1240) -> ()  [unwired: 2 in, 2 out]
        n608 = property on="Program Spin Coater" class="Arr (strict)"() -> ("Value"=w1241:T2)  [unwired: 2 in, 2 out]
        n609 = property on="Program Spin Coater" class="Arr (strict)"("Val(Sgnl)"=w1241) -> ()  [unwired: 2 in, 2 out]
      }
      event "Spin Time": Value Change {
        n610 = event-data() -> ()  [unwired: 1 in, 6 out]
        n611 = property on="Program Spin Coater" class="Arr (strict)"() -> ("Value"=w1248:T2)  [unwired: 2 in, 2 out]
        n612 = property on="Program Spin Coater" class="Arr (strict)"("Val(Sgnl)"=w1248) -> ()  [unwired: 2 in, 2 out]
      }
      event "Seconds after Spin": Value Change {
        n613 = event-data() -> ()  [unwired: 1 in, 6 out]
        n614 = property on="Measure_IntegrationTime" class="DigNum (strict)"() -> ("Value"=w1252:dbl[unit])  [unwired: 2 in, 2 out]
        n615 = property on="Measure_IntegrationTime" class="DigNum (strict)"("Val(Sgnl)"=w1252) -> ()  [unwired: 2 in, 2 out]
      }
      event "Calculate Frames_Normal", "Calculate Frames_Short": Value Change {
        n616 = event-data() -> ("NewVal"=w1253:bool)  [unwired: 1 in, 5 out]
        n617 = case shown="False" w1253 {
          tunnel: [0 2] -> w1255
          tunnel: w1257 -> [w1261 w1270]
          tunnel: [w1261 w1268] -> w1258
          tunnel: w1256 -> [w1260 w1267]
          tunnel: [w1260 w1263] -> w1254
          frame False {
          }
          frame True {
            w1269 = T11 {"QueueAction"=enum."TimeOut", "Numeric 1"=0.0, "Numeric 2"=0.0, "Boolean 1"=FALSE, "Boolean 2"=FALSE, "Spin Program"=[], "Spin Prg v07"=[], "Time Stamp"=timestamp(0 s since 1904-01-01), "TabControl"=enum."Measure"}  # Device Queue
            n618 = property on="Measure_IntegrationTime" class="DigNum (strict)"() -> ("Value"=w1265:dbl[unit])  [unwired: 2 in, 2 out]
            n619 = node(w1265) -> (w1264:dbl)
            n620 = Bundle By Name(cluster=w1269, "QueueAction"=DeviceQueue_Action."Spectrometer_SetIntegrationTime", "Numeric 1"=w1264) -> (w1271:T11)
            n621 = Enqueue Element(queue=w1270, element=w1271, error in (no error)=w1267) -> (queue out=w1268:refnum<queue>, error out=w1263:errorcluster)  [unwired: 1 in, 1 out]
          }
        }
        n622 = property on="Calculate Frames_Short" class="Bool (strict)"("Value"=w1253) -> ()  [unwired: 2 in, 2 out]
        n623 = property on="Calculate Frames_Normal" class="Bool (strict)"("Value"=w1253) -> ()  [unwired: 2 in, 2 out]
        n624 = property on="Frames" class="DigNum (strict)"("DisabledEnum"=w1255) -> ()  [unwired: 2 in, 2 out]
      }
      event "Record RefSpec": Value Change {
        w1278 = T11 {"QueueAction"=enum."TimeOut", "Numeric 1"=0.0, "Numeric 2"=0.0, "Boolean 1"=FALSE, "Boolean 2"=FALSE, "Spin Program"=[], "Spin Prg v07"=[], "Time Stamp"=timestamp(0 s since 1904-01-01), "TabControl"=enum."Measure"}  # Device Queue
        n625 = event-data() -> ()  [unwired: 1 in, 6 out]
        n626 = property on="Shutter Toggle" class="Bool (strict)"("Value"=FALSE ("Shutter Toggle")) -> ()  [unwired: 2 in, 2 out]
        n627 = property on="Frames for Ref/Dark" class="DigNum (strict)"() -> ("Value"=w1287:dbl)  [unwired: 2 in, 2 out]
        n628 = property on="Measure_FramesSpectrometer" class="DigNum (strict)"() -> ("Value"=w1282:dbl)  [unwired: 2 in, 2 out]
        n629 = Bundle By Name(cluster=w1278, "QueueAction"=DeviceQueue_Action."Spectrometer_SetTriggerMode", "Numeric 1"=0.0) -> (w1277:T11)
        n630 = Bundle By Name(cluster=w1277, "QueueAction"=DeviceQueue_Action."Arduino_Shutter_Open") -> (w1273:T11)
        n631 = Bundle By Name(cluster=w1273, "QueueAction"=DeviceQueue_Action."Wait", "Numeric 1"=0.5) -> (w1288:T11)
        n632 = Enqueue Element(queue=w1297, element=w1277, error in (no error)=w1274) -> (queue out=w1279:refnum<queue>, error out=w1275:errorcluster)  [unwired: 1 in, 1 out]
        n633 = Bundle By Name(cluster=w1288, "QueueAction"=DeviceQueue_Action."Spectrometer_SetFrames", "Numeric 1"=w1287) -> (w1286:T11)
        n634 = Enqueue Element(queue=w1279, element=w1273, error in (no error)=w1275) -> (queue out=w1303:refnum<queue>, error out=w1300:errorcluster)  [unwired: 1 in, 1 out]
        n635 = Bundle By Name(cluster=w1286, "QueueAction"=DeviceQueue_Action."Spectrometer_SetReference") -> (w1285:T11)
        n636 = Enqueue Element(queue=w1303, element=w1288, error in (no error)=w1300) -> (queue out=w1302:refnum<queue>, error out=w1299:errorcluster)  [unwired: 1 in, 1 out]
        n637 = Bundle By Name(cluster=w1285, "QueueAction"=DeviceQueue_Action."Arduino_Shutter_Close") -> (w1283:T11)
        n638 = Enqueue Element(queue=w1302, element=w1286, error in (no error)=w1299) -> (queue out=w1301:refnum<queue>, error out=w1298:errorcluster)  [unwired: 1 in, 1 out]
        n639 = Bundle By Name(cluster=w1283, "QueueAction"=DeviceQueue_Action."Spectrometer_SetFrames", "Numeric 1"=w1282) -> (w1281:T11)
        n640 = Enqueue Element(queue=w1301, element=w1285, error in (no error)=w1298) -> (queue out=w1294:refnum<queue>, error out=w1295:errorcluster)  [unwired: 1 in, 1 out]
        n641 = Enqueue Element(queue=w1294, element=w1283, error in (no error)=w1295) -> (queue out=w1292:refnum<queue>, error out=w1293:errorcluster)  [unwired: 1 in, 1 out]
        n642 = Enqueue Element(queue=w1292, element=w1281, error in (no error)=w1293) -> (queue out=w1290:refnum<queue>, error out=w1291:errorcluster)  [unwired: 1 in, 1 out]
      }
      event "Measure_Preview", "SpectralStability_Preview": Value Change {
        n643 = event-data() -> ("NewVal"=w1310:bool)  [unwired: 1 in, 5 out]
        n644 = case shown="False" w1310 {
          tunnel: w1315 -> [w1317 w1322]
          tunnel: w1313 -> [w1316 w1321]
          tunnel: [w1317 w1320] -> w1312
          tunnel: [w1316 w1319] -> w1311
          frame False {
          }
          frame True {
            w1325 = T11 {"QueueAction"=enum."TimeOut", "Numeric 1"=0.0, "Numeric 2"=0.0, "Boolean 1"=FALSE, "Boolean 2"=FALSE, "Spin Program"=[], "Spin Prg v07"=[], "Time Stamp"=timestamp(0 s since 1904-01-01), "TabControl"=enum."Measure"}  # Device Queue
            n645 = property on="Tab Control" class="TabCtl (strict)"() -> ("Value"=w1318:T1)  [unwired: 2 in, 2 out]
            n646 = Bundle By Name(cluster=w1325, "QueueAction"=DeviceQueue_Action."Spectrometer_Preview", "TabControl"=w1318) -> (w1324:T11)
            n647 = Enqueue Element(queue=w1322, element=w1324, error in (no error)=w1321) -> (queue out=w1320:refnum<queue>, error out=w1319:errorcluster)  [unwired: 1 in, 1 out]
          }
        }
      }
      event "Measure:\nRecord_Darkspec", "SpectralStability:\nRecord_Darkspec": Value Change {
        w1356 = T11 {"QueueAction"=enum."TimeOut", "Numeric 1"=0.0, "Numeric 2"=0.0, "Boolean 1"=FALSE, "Boolean 2"=FALSE, "Spin Program"=[], "Spin Prg v07"=[], "Time Stamp"=timestamp(0 s since 1904-01-01), "TabControl"=enum."Measure"}  # Device Queue
        n648 = event-data() -> ()  [unwired: 1 in, 6 out]
        n649 = property on="Shutter Toggle" class="Bool (strict)"("Value"=FALSE ("Shutter Toggle")) -> ()  [unwired: 2 in, 2 out]
        n650 = property on="Frames for Ref/Dark" class="DigNum (strict)"() -> ("Value"=w1341:dbl)  [unwired: 2 in, 2 out]
        n651 = property on="Measure_FramesSpectrometer" class="DigNum (strict)"() -> ("Value"=w1335:dbl)  [unwired: 2 in, 2 out]
        n652 = Bundle By Name(cluster=w1356, "QueueAction"=DeviceQueue_Action."Arduino_Shutter_Close") -> (w1331:T11)
        n653 = Bundle By Name(cluster=w1331, "QueueAction"=DeviceQueue_Action."Spectrometer_SetTriggerMode", "Numeric 1"=0.0) -> (w1330:T11)
        n654 = Bundle By Name(cluster=w1330, "QueueAction"=DeviceQueue_Action."Wait", "Numeric 1"=0.5) -> (w1355:T11)
        n655 = Bundle By Name(cluster=w1355, "QueueAction"=DeviceQueue_Action."Spectrometer_SetFrames", "Numeric 1"=w1341) -> (w1339:T11)
        n656 = Enqueue Element(queue=w1351, element=w1331, error in (no error)=w1350) -> (queue out=w1349:refnum<queue>, error out=w1327:errorcluster)  [unwired: 1 in, 1 out]
        n657 = Bundle By Name(cluster=w1339, "QueueAction"=DeviceQueue_Action."Spectrometer_SetDarkspec") -> (w1337:T11)
        n658 = Enqueue Element(queue=w1349, element=w1330, error in (no error)=w1327) -> (queue out=w1332:refnum<queue>, error out=w1326:errorcluster)  [unwired: 1 in, 1 out]
        n659 = Bundle By Name(cluster=w1337, "QueueAction"=DeviceQueue_Action."Spectrometer_SetFrames", "Numeric 1"=w1335) -> (w1338:T11)
        n660 = Enqueue Element(queue=w1332, element=w1355, error in (no error)=w1326) -> (queue out=w1347:refnum<queue>, error out=w1348:errorcluster)  [unwired: 1 in, 1 out]
        n661 = Enqueue Element(queue=w1347, element=w1339, error in (no error)=w1348) -> (queue out=w1345:refnum<queue>, error out=w1344:errorcluster)  [unwired: 1 in, 1 out]
        n662 = Enqueue Element(queue=w1345, element=w1337, error in (no error)=w1344) -> (queue out=w1343:refnum<queue>, error out=w1342:errorcluster)  [unwired: 1 in, 1 out]
        n663 = Enqueue Element(queue=w1343, element=w1338, error in (no error)=w1342) -> (queue out=w1333:refnum<queue>, error out=w1334:errorcluster)  [unwired: 1 in, 1 out]
      }
      event "StartMeasurement_Button": Value Change {
        w1372 = T8 {"QueueAction"=enum."TimeOut", "Data"=[], "Data_Raw"=[], "Data_Dark"=[], "Data_Ref"=[], "Device Information"=[], "Numeric Control"=0.0, "Boolean"=FALSE, "Wavelength"=[], "Time"=[], "Time Stamp"=timestamp(0 s since 1904-01-01), "Numeric Control 2"=0.0, "TabControl"=enum."Measure", "Numeric Control 3"=0.0}  # DataQueue
        w1379 = T11 {"QueueAction"=enum."TimeOut", "Numeric 1"=0.0, "Numeric 2"=0.0, "Boolean 1"=FALSE, "Boolean 2"=FALSE, "Spin Program"=[], "Spin Prg v07"=[], "Time Stamp"=timestamp(0 s since 1904-01-01), "TabControl"=enum."Measure"}  # Device Queue
        n664 = event-data() -> ()  [unwired: 1 in, 6 out]
        n665 = property on="Measure_Preview" class="Bool (strict)"("Value"=FALSE ("Preview")) -> ()  [unwired: 2 in, 2 out]
        n666 = case shown="\"Normal\", Default" "Tab Control SpinType" {
          tunnel: [DeviceQueue_Action."Measure_InSituAdvanced" ("QueueAction") DeviceQueue_Action."Measure_InSituAdvanced_Short" ("QueueAction")] -> w1365
          tunnel: [DataQueue_Action."Measure_InSituSpinCoating" ("QueueAction") DataQueue_Action."Measure_InSituSpinCoating_Short" ("QueueAction")] -> w1364
          frame "Normal", Default {
            n667 = property on="Motor_ShortStop" class="Bool (strict)"("Value"=FALSE ("Motor_ShortStop")) -> ()  [unwired: 2 in, 2 out]
          }
          frame "Short" {
            n668 = property on="Motor_ShortStop" class="Bool (strict)"("Value"=TRUE ("Motor_ShortStop")) -> ()  [unwired: 2 in, 2 out]
          }
        }
        n669 = Get Date/Time In Seconds() -> (seconds since 1Jan1904=w1367:timestamp)
        n670 = Bundle By Name(cluster=w1379, "QueueAction"=w1365, "Time Stamp"=w1367) -> (w1378:T11)
        n671 = Enqueue Element(queue=w1377, element=w1378, error in (no error)=w1375) -> (queue out=w1376:refnum<queue>, error out=w1368:errorcluster)  [unwired: 1 in, 1 out]
        n672 = property on="Reference\nValue" class="DigNum (strict)"("Value"=1.0 ("Reference\nValue")) -> ()  [unwired: 2 in, 2 out]
        n673 = Bundle By Name(cluster=w1372, "QueueAction"=w1364, "Time Stamp"=w1367) -> (w1373:T8)
        n674 = Enqueue Element(queue=w1371, element=w1373, error in (no error)=w1368) -> (queue out=w1370:refnum<queue>, error out=w1369:errorcluster)  [unwired: 1 in, 1 out]
        n675 = Concatenate Strings("Measure_FileName", "_", "Cell") -> (→"fName_Temp":string)
      }
      event "StartSpin_Button": Value Change {
        w1398 = T11 {"QueueAction"=enum."TimeOut", "Numeric 1"=0.0, "Numeric 2"=0.0, "Boolean 1"=FALSE, "Boolean 2"=FALSE, "Spin Program"=[], "Spin Prg v07"=[], "Time Stamp"=timestamp(0 s since 1904-01-01), "TabControl"=enum."Measure"}  # Device Queue
        n676 = event-data() -> ()  [unwired: 1 in, 6 out]
        n677 = Bundle By Name(cluster=w1398, "QueueAction"=DeviceQueue_Action."Arduino_StartProgram", "Numeric 1"=1.0) -> (w1389:T11)
        n678 = Bundle By Name(cluster=w1389, "QueueAction"=DeviceQueue_Action."Arduino_Shutter_Close") -> (w1387:T11)
        n679 = Enqueue Element(queue=w1397, element=w1389, error in (no error)=w1395) -> (queue out=w1392:refnum<queue>, error out=w1393:errorcluster)  [unwired: 1 in, 1 out]
        n680 = Enqueue Element(queue=w1392, element=w1387, error in (no error)=w1393) -> (queue out=w1391:refnum<queue>, error out=w1390:errorcluster)  [unwired: 1 in, 1 out]
      }
      event "ESC_Milliseconds": Value Change {
        w1407 = T11 {"QueueAction"=enum."TimeOut", "Numeric 1"=0.0, "Numeric 2"=0.0, "Boolean 1"=FALSE, "Boolean 2"=FALSE, "Spin Program"=[], "Spin Prg v07"=[], "Time Stamp"=timestamp(0 s since 1904-01-01), "TabControl"=enum."Measure"}  # Device Queue
        n681 = event-data() -> ()  [unwired: 1 in, 6 out]
        n682 = Bundle By Name(cluster=w1407, "QueueAction"=DeviceQueue_Action."Arduino_SetMillis", "Numeric 1"="ESC_Milliseconds") -> (w1403:T11)
        n683 = Enqueue Element(queue=w1406, element=w1403, error in (no error)=w1404) -> (queue out=w1402:refnum<queue>, error out=w1401:errorcluster)  [unwired: 1 in, 1 out]
      }
      event "ESC_Speed": Value Change {
        w1416 = T11 {"QueueAction"=enum."TimeOut", "Numeric 1"=0.0, "Numeric 2"=0.0, "Boolean 1"=FALSE, "Boolean 2"=FALSE, "Spin Program"=[], "Spin Prg v07"=[], "Time Stamp"=timestamp(0 s since 1904-01-01), "TabControl"=enum."Measure"}  # Device Queue
        n684 = event-data() -> ()  [unwired: 1 in, 6 out]
        n685 = Bundle By Name(cluster=w1416, "QueueAction"=DeviceQueue_Action."Arduino_SetSpeed", "Numeric 1"="ESC_Speed") -> (w1412:T11)
        n686 = Enqueue Element(queue=w1415, element=w1412, error in (no error)=w1413) -> (queue out=w1411:refnum<queue>, error out=w1410:errorcluster)  [unwired: 1 in, 1 out]
      }
      event "ESC DEBUG": Value Change {
        n687 = event-data() -> ()  [unwired: 1 in, 6 out]
        n688 = Select(t=u8 0, s="ESC DEBUG", f=u8 2) -> (s? t:f=w1417:u8)
        n689 = property on="ESC_Milliseconds" class="DigNum (strict)"("DisabledEnum"=w1417) -> ()  [unwired: 2 in, 2 out]
        n690 = property on="ESC_Speed" class="DigNum (strict)"("DisabledEnum"=w1417) -> ()  [unwired: 2 in, 2 out]
      }
      event "Measure_FramesSpectrometer", "SpectralStability_FramesSpectrometer": Value Change {
        w1431 = T11 {"QueueAction"=enum."TimeOut", "Numeric 1"=0.0, "Numeric 2"=0.0, "Boolean 1"=FALSE, "Boolean 2"=FALSE, "Spin Program"=[], "Spin Prg v07"=[], "Time Stamp"=timestamp(0 s since 1904-01-01), "TabControl"=enum."Measure"}  # Device Queue
        n691 = event-data() -> ("NewVal"=w1425:dbl)  [unwired: 1 in, 5 out]
        n692 = property on="Tab Control" class="TabCtl (strict)"() -> ("Value"=w1424:T1)  [unwired: 2 in, 2 out]
        n693 = Bundle By Name(cluster=w1431, "QueueAction"=DeviceQueue_Action."Spectrometer_SetFrames", "Numeric 1"=w1425, "TabControl"=w1424) -> (w1432:T11)
        n694 = Enqueue Element(queue=w1429, element=w1432) -> (queue out=w1426:refnum<queue>)  [unwired: 2 in, 2 out]
      }
      event "Measure_MeasureSpectrum", "SpectralStability_MeasureSpectrum": Value Change {
        w1448 = T8 {"QueueAction"=enum."TimeOut", "Data"=[], "Data_Raw"=[], "Data_Dark"=[], "Data_Ref"=[], "Device Information"=[], "Numeric Control"=0.0, "Boolean"=FALSE, "Wavelength"=[], "Time"=[], "Time Stamp"=timestamp(0 s since 1904-01-01), "Numeric Control 2"=0.0, "TabControl"=enum."Measure", "Numeric Control 3"=0.0}  # DataQueue
        n695 = event-data() -> ()  [unwired: 1 in, 6 out]
        n696 = property on="Tab Control" class="TabCtl (strict)"() -> ("Value"=w1440:T1)  [unwired: 2 in, 2 out]
        n697 = case shown="\"Measure\"" w1440 {
          tunnel: w1442 -> [w1460 w1463]
          tunnel: [w1460 w1462] -> w1441
          tunnel: [w1459 w1461] -> w1439
          frame Default {
            w1459 = T11 {"QueueAction"=enum."TimeOut", "Numeric 1"=0.0, "Numeric 2"=0.0, "Boolean 1"=FALSE, "Boolean 2"=FALSE, "Spin Program"=[], "Spin Prg v07"=[], "Time Stamp"=timestamp(0 s since 1904-01-01), "TabControl"=enum."Measure"}  # Device Queue
          }
          frame "Measure" {
            w1466 = T11 {"QueueAction"=enum."TimeOut", "Numeric 1"=0.0, "Numeric 2"=0.0, "Boolean 1"=FALSE, "Boolean 2"=FALSE, "Spin Program"=[], "Spin Prg v07"=[], "Time Stamp"=timestamp(0 s since 1904-01-01), "TabControl"=enum."Measure"}  # Device Queue
            (unwired) T11 {"QueueAction"=enum."TimeOut", "Numeric 1"=0.0, "Numeric 2"=0.0, "Boolean 1"=FALSE, "Boolean 2"=FALSE, "Spin Program"=[], "Spin Prg v07"=[], "Time Stamp"=timestamp(0 s since 1904-01-01), "TabControl"=enum."Measure"}  # Device Queue
            n698 = Bundle By Name(cluster=w1466, "QueueAction"=DeviceQueue_Action."Spectrometer_SetFrames", "Numeric 1"="Frames for Ref/Dark") -> (w1461:T11)
            n699 = Enqueue Element(queue=w1463, element=w1461) -> (queue out=w1462:refnum<queue>)  [unwired: 2 in, 2 out]
          }
        }
        n700 = Get Date/Time In Seconds() -> (seconds since 1Jan1904=w1443:timestamp)
        n701 = Bundle By Name(cluster=w1439, "QueueAction"=DeviceQueue_Action."Measure_Spectrum", "Time Stamp"=w1443, "TabControl"=w1440) -> (w1451:T11)
        n702 = property on="Cell" class="Str"() -> ("Value"=w1433:string)  [unwired: 2 in, 2 out]
        n703 = property on="Measure_FileName" class="Str"() -> ("Value"=w1435:string)  [unwired: 2 in, 2 out]
        n704 = Concatenate Strings(w1435, "_", w1433) -> (w1436:string)
        n705 = Enqueue Element(queue=w1441, element=w1451) -> (queue out=w1438:refnum<queue>)  [unwired: 2 in, 2 out]
        n706 = property on="fName_Temp" class="Str"("Value"=w1436) -> ()  [unwired: 2 in, 2 out]
        n707 = case shown="Default" w1440 {
          tunnel: w1439 -> [_ w1457]
          tunnel: w1438 -> [w1452 w1456]
          tunnel: [w1452 w1455] -> w1437
          frame Default {
          }
          frame "Measure" {
            n708 = property on="Measure_FramesSpectrometer" class="DigNum (strict)"() -> ("Value"=w1454:dbl)  [unwired: 2 in, 2 out]
            n709 = Bundle By Name(cluster=w1457, "QueueAction"=DeviceQueue_Action."Spectrometer_SetFrames", "Numeric 1"=w1454) -> (w1453:T11)
            n710 = Enqueue Element(queue=w1456, element=w1453) -> (queue out=w1455:refnum<queue>)  [unwired: 2 in, 2 out]
          }
        }
        n711 = Bundle By Name(cluster=w1448, "QueueAction"=DataQueue_Action."Measure_Spectrum", "TabControl"=w1440) -> (w1445:T8)
        n712 = Enqueue Element(queue=w1446, element=w1445) -> (queue out=w1444:refnum<queue>)  [unwired: 2 in, 2 out]
      }
      event "SpectralStability_Record": Value Change {
        w1475 = T8 {"QueueAction"=enum."TimeOut", "Data"=[], "Data_Raw"=[], "Data_Dark"=[], "Data_Ref"=[], "Device Information"=[], "Numeric Control"=0.0, "Boolean"=FALSE, "Wavelength"=[], "Time"=[], "Time Stamp"=timestamp(0 s since 1904-01-01), "Numeric Control 2"=0.0, "TabControl"=enum."Measure", "Numeric Control 3"=0.0}  # DataQueue
        w1480 = T11 {"QueueAction"=enum."TimeOut", "Numeric 1"=0.0, "Numeric 2"=0.0, "Boolean 1"=FALSE, "Boolean 2"=FALSE, "Spin Program"=[], "Spin Prg v07"=[], "Time Stamp"=timestamp(0 s since 1904-01-01), "TabControl"=enum."Measure"}  # Device Queue
        n713 = event-data() -> ()  [unwired: 1 in, 6 out]
        n714 = property on="Duration/\nTimes" class="Bool (strict)"() -> ("Value"=w1468:bool)  [unwired: 2 in, 2 out]
        n715 = case shown="False" w1468 {
          tunnel: ["SpectralStability_\nMeasurementNumber" w1483] -> w1467
          frame False {
            # "Number"
          }
          frame True {
            # "Duration"
            n716 = property on="SpectralStability_\nPeriodicTime" class="DigNum (strict)"() -> ("Value"=w1485:dbl[unit])  [unwired: 2 in, 2 out]
            n717 = Divide(x="SpectralStability_Duration", y=w1485) -> (x/y=w1486:dbl)
            n718 = Round Toward +Infinity(x=w1486) -> (ceil(x): smallest int >= x=w1484:dbl)
            n719 = Increment(x=w1484) -> (x+1=w1483:dbl)
          }
        }
        n720 = Get Date/Time In Seconds() -> (seconds since 1Jan1904=w1469:timestamp)
        n721 = property on="Tab Control" class="TabCtl (strict)"() -> ("Value"=w1470:T1)  [unwired: 2 in, 2 out]
        n722 = Bundle By Name(cluster=w1480, "QueueAction"=DeviceQueue_Action."Measure_SpectralStability", "Time Stamp"=w1469, "TabControl"=w1470, "Numeric 1"=w1467) -> (w1481:T11)
        n723 = property on="SS_StepsLeft" class="DigNum (strict)"("Value"=w1467) -> ()  [unwired: 2 in, 2 out]
        n724 = Enqueue Element(queue=w1478, element=w1481) -> (queue out=w1476:refnum<queue>)  [unwired: 2 in, 2 out]
        n725 = Bundle By Name(cluster=w1475, "QueueAction"=DataQueue_Action."Measure_SpectralStability", "TabControl"=w1470, "Time Stamp"=w1469, "Numeric Control"=w1467) -> (w1472:T8)
        n726 = Enqueue Element(queue=w1473, element=w1472) -> (queue out=w1471:refnum<queue>)  [unwired: 2 in, 2 out]
      }
      event "Automatically \nadjust count": Value Change {
        n727 = event-data() -> ("NewVal"=w1494:bool)  [unwired: 1 in, 5 out]
        n728 = Select(t=u8 2, s=w1494, f=u8 0) -> (s? t:f=w1488:u8)
        n729 = property on="Spectra Count" class="DigNum (strict)"("DisabledEnum"=w1488) -> ()  [unwired: 2 in, 2 out]
      }
      event "Duration/Times": Value Change {
        n730 = event-data() -> ("NewVal"=w1500:bool)  [unwired: 1 in, 5 out]
        n731 = case shown="False" w1500 {
          tunnel: [FALSE TRUE] -> w1499
          tunnel: [TRUE FALSE] -> w1498
          frame False {
          }
          frame True {
          }
        }
        n732 = property on="SpectralStability_Duration" class="DigNum (strict)"("Visible"=w1499) -> ()  [unwired: 2 in, 2 out]
        n733 = property on="SpectralStability_\nMeasurementNumber" class="DigNum (strict)"("Visible"=w1498) -> ()  [unwired: 2 in, 2 out]
      }
      event "Tab Control": Value Change {
        w1505 = FALSE ("SpectralStability_Preview")
        n734 = event-data() -> ("NewVal"=w1508:T1)  [unwired: 1 in]
        n735 = case shown="\"Spectral Stability\"" w1508 {
          tunnel: w1510 -> [w1513 w1526 w1541]
          tunnel: [w1513 w1515 w1532] -> w1507
          tunnel: w1509 -> [w1512 w1525 w1540]
          tunnel: w1508 -> [_ w1524 w1539]
          tunnel: [w1512 w1514 w1531] -> w1506
          frame Default {
          }
          frame "Measure" {
            w1528 = T11 {"QueueAction"=enum."TimeOut", "Numeric 1"=0.0, "Numeric 2"=0.0, "Boolean 1"=FALSE, "Boolean 2"=FALSE, "Spin Program"=[], "Spin Prg v07"=[], "Time Stamp"=timestamp(0 s since 1904-01-01), "TabControl"=enum."Measure"}  # Device Queue
            n736 = property on="Measure_IntegrationTime" class="DigNum (strict)"() -> ("Value"=w1523:dbl[unit])  [unwired: 2 in, 2 out]
            n737 = node(w1523) -> (w1522:dbl)
            n738 = Bundle By Name(cluster=w1528, "QueueAction"=DeviceQueue_Action."Spectrometer_SetIntegrationTime", "Numeric 1"=w1522, "TabControl"=w1524) -> (w1519:T11)
            n739 = property on="Measure_FramesSpectrometer" class="DigNum (strict)"() -> ("Value"=w1517:dbl)  [unwired: 2 in, 2 out]
            n740 = Enqueue Element(queue=w1526, element=w1519, error in (no error)=w1525) -> (queue out=w1521:refnum<queue>, error out=w1520:errorcluster)  [unwired: 1 in, 1 out]
            n741 = Bundle By Name(cluster=w1519, "QueueAction"=DeviceQueue_Action."Spectrometer_SetFrames", "Numeric 1"=w1517) -> (w1516:T11)
            n742 = Enqueue Element(queue=w1521, element=w1516, error in (no error)=w1520) -> (queue out=w1515:refnum<queue>, error out=w1514:errorcluster)  [unwired: 1 in, 1 out]
          }
          frame "Spectral Stability" {
            w1543 = T11 {"QueueAction"=enum."TimeOut", "Numeric 1"=0.0, "Numeric 2"=0.0, "Boolean 1"=FALSE, "Boolean 2"=FALSE, "Spin Program"=[], "Spin Prg v07"=[], "Time Stamp"=timestamp(0 s since 1904-01-01), "TabControl"=enum."Measure"}  # Device Queue
            n743 = property on="SpectralStability_IntegrationTime" class="DigNum (strict)"() -> ("Value"=w1530:dbl[unit])  [unwired: 2 in, 2 out]
            n744 = node(w1530) -> (w1538:dbl)
            n745 = property on="SpectralStability_FramesSpectrometer" class="DigNum (strict)"() -> ("Value"=w1529:dbl)  [unwired: 2 in, 2 out]
            n746 = Bundle By Name(cluster=w1543, "QueueAction"=DeviceQueue_Action."Spectrometer_SetIntegrationTime", "Numeric 1"=w1538, "TabControl"=w1539) -> (w1535:T11)
            n747 = Enqueue Element(queue=w1541, element=w1535, error in (no error)=w1540) -> (queue out=w1537:refnum<queue>, error out=w1536:errorcluster)  [unwired: 1 in, 1 out]
            n748 = Bundle By Name(cluster=w1535, "QueueAction"=DeviceQueue_Action."Spectrometer_SetFrames", "Numeric 1"=w1529) -> (w1533:T11)
            n749 = Enqueue Element(queue=w1537, element=w1533, error in (no error)=w1536) -> (queue out=w1532:refnum<queue>, error out=w1531:errorcluster)  [unwired: 1 in, 1 out]
          }
        }
        n750 = property on="SpectralStability_Preview" class="Bool (strict)"("Value"=w1505) -> ()  [unwired: 2 in, 2 out]
        n751 = property on="Measure_Preview" class="Bool (strict)"("Value"=w1505) -> ()  [unwired: 2 in, 2 out]
      }
      event "TrimSpec", "WlUp", "WlLow": Value Change {
        w1553 = T8 {"QueueAction"=enum."TimeOut", "Data"=[], "Data_Raw"=[], "Data_Dark"=[], "Data_Ref"=[], "Device Information"=[], "Numeric Control"=0.0, "Boolean"=FALSE, "Wavelength"=[], "Time"=[], "Time Stamp"=timestamp(0 s since 1904-01-01), "Numeric Control 2"=0.0, "TabControl"=enum."Measure", "Numeric Control 3"=0.0}  # DataQueue
        n752 = event-data() -> ()  [unwired: 1 in, 6 out]
        n753 = node("WlLow") -> (w1547:dbl)
        n754 = node("WlUp") -> (w1546:dbl)
        n755 = Bundle By Name(cluster=w1553, "QueueAction"=DataQueue_Action."Change_TrimSettings", "Numeric Control"=w1547, "Numeric Control 2"=w1546, "Boolean"="TrimSpec") -> (w1554:T8)
        n756 = Enqueue Element(queue=w1552, element=w1554) -> (queue out=w1551:refnum<queue>)  [unwired: 2 in, 2 out]
      }
      event "Motor_ShortStop": Value Change {
        w1562 = T11 {"QueueAction"=enum."TimeOut", "Numeric 1"=0.0, "Numeric 2"=0.0, "Boolean 1"=FALSE, "Boolean 2"=FALSE, "Spin Program"=[], "Spin Prg v07"=[], "Time Stamp"=timestamp(0 s since 1904-01-01), "TabControl"=enum."Measure"}  # Device Queue
        n757 = event-data() -> ()  [unwired: 1 in, 6 out]
        n758 = Bundle By Name(cluster=w1562, "QueueAction"=DeviceQueue_Action."Arduino_ShortStop") -> (w1561:T11)
        n759 = Enqueue Element At Opposite End(queue=w1560, element=w1561, error in (no error)=w1557) -> (queue out=w1559:refnum<queue>, error out=w1556:errorcluster)  [unwired: 1 in, 1 out]
      }
    }
  }
  n760 = while {
    tunnel: w1 -> [w1566]
    stop <- w1564 stop-if-true
    # "Save And Open Preset"
    n761 = event shown="[2] \"MeasureSavePreset\": Value Change" {
      selector: w1566 -> [_ _ _ _]
      dyn-events: _ -> [_ _ _ _]
      timeout: -1 -> [_ _ _ _]
      tunnel: [_ TRUE _ _] -> w1564
      event Timeout {
        n762 = event-data() -> ()  [unwired: 1 in, 1 out]
      }
      event User Event {
        n763 = event-data() -> ()  [unwired: 1 in, 5 out]
      }
      event "MeasureSavePreset": Value Change {
        w1608 = T20 {"Measure_IntegrationTime"=0.0, "Measure_FramesSpec"=0.0, "Frames_ForRef/Dark"=0.0, "Program Spin Coater"=[], "TabControlSpinType"=0, "Seconds2Spin_Norm"=0.0, "SecondsAftSpin_Norm"=0.0, "CalcFrames_Norm"=FALSE, "PeriodicTime"=0.0, "DurationAfter"=0.0, "SpinAtEnd"=FALSE, "Seconds2Spin_Short"=0.0, "SpinTime"=0.0, "CalculateFrames_Short"=FALSE, "TimeDetect"=0.0, "WavelengthDetect"=0.0, "Threshold"=0.0, "WlLow"=0.0, "WlUp"=0.0, "TrimSpec"=FALSE}  # PresetCluster
        # "Deletes, that action is aborted"
        n764 = event-data() -> ()  [unwired: 1 in, 1 out]
        n765 = property on="Measure_IntegrationTime" class="DigNum (strict)"() -> ("Value"=w1600:dbl[unit])  [unwired: 2 in, 2 out]
        n766 = property on="Measure_FramesSpectrometer" class="DigNum (strict)"() -> ("Value"=w1588:dbl)  [unwired: 2 in, 2 out]
        n767 = property on="Frames for Ref/Dark" class="DigNum (strict)"() -> ("Value"=w1587:dbl)  [unwired: 2 in, 2 out]
        n768 = property on="Program Spin Coater" class="Arr (strict)"() -> ("Value"=w1586:T2)  [unwired: 2 in, 2 out]
        n769 = property on="Tab Control SpinType" class="TabCtl (strict)"() -> ("Value"=w1601:T4)  [unwired: 2 in, 2 out]
        n770 = property on="Seconds to Spin_Normal" class="DigNum (strict)"() -> ("Value"=w1599:dbl[unit])  [unwired: 2 in, 2 out]
        n771 = property on="Seconds after Spin" class="DigNum (strict)"() -> ("Value"=w1598:dbl[unit])  [unwired: 2 in, 2 out]
        n772 = property on="Calculate Frames_Normal" class="Bool (strict)"() -> ("Value"=w1582:bool)  [unwired: 2 in, 2 out]
        n773 = property on="periodic time" class="DigNum (strict)"() -> ("Value"=w1597:dbl[unit])  [unwired: 2 in, 2 out]
        n774 = property on="Duration after" class="DigNum (strict)"() -> ("Value"=w1596:dbl[unit])  [unwired: 2 in, 2 out]
        n775 = property on="Spin at end" class="Bool (strict)"() -> ("Value"=w1579:bool)  [unwired: 2 in, 2 out]
        n776 = property on="Seconds to Spin_Short" class="DigNum (strict)"() -> ("Value"=w1595:dbl[unit])  [unwired: 2 in, 2 out]
        n777 = property on="Spin Time" class="DigNum (strict)"() -> ("Value"=w1594:dbl[unit])  [unwired: 2 in, 2 out]
        n778 = property on="Calculate Frames_Short" class="Bool (strict)"() -> ("Value"=w1576:bool)  [unwired: 2 in, 2 out]
        n779 = property on="Time Detect" class="DigNum (strict)"() -> ("Value"=w1593:dbl[unit])  [unwired: 2 in, 2 out]
        n780 = property on="Wavelenght Detect" class="DigNum (strict)"() -> ("Value"=w1592:dbl[unit])  [unwired: 2 in, 2 out]
        n781 = property on="Threshold" class="DigNum (strict)"() -> ("Value"=w1573:dbl)  [unwired: 2 in, 2 out]
        n782 = property on="WlLow" class="DigNum (strict)"() -> ("Value"=w1591:dbl[unit])  [unwired: 2 in, 2 out]
        n783 = property on="WlUp" class="DigNum (strict)"() -> ("Value"=w1590:dbl[unit])  [unwired: 2 in, 2 out]
        n784 = property on="TrimSpec" class="Bool (strict)"() -> ("Value"=w1570:bool)  [unwired: 2 in, 2 out]
        n785 = Current VI's Path() -> (path=w1610:path)
        n786 = To Unsigned Long Integer(number=w1601) -> (unsigned 32bit integer=w1585:u32)
        n787 = node(w1592) -> (w1574:dbl)
        n788 = node(w1591) -> (w1572:dbl)
        n789 = node(w1590) -> (w1571:dbl)
        n790 = node(w1600) -> (w1589:dbl)
        n791 = node(w1599) -> (w1584:dbl)
        n792 = node(w1598) -> (w1583:dbl)
        n793 = node(w1597) -> (w1581:dbl)
        n794 = node(w1596) -> (w1580:dbl)
        n795 = node(w1595) -> (w1578:dbl)
        n796 = node(w1594) -> (w1577:dbl)
        n797 = node(w1593) -> (w1575:dbl)
        n798 = Strip Path(path=w1610) -> (stripped path=w1611:path)  [unwired: 1 out]
        n799 = Build Path(base path=w1611, name or relative path=path "Presets" ("start path")) -> (appended path=w1612:path)
        n800 = call "File Dialog2"("start path"=w1612, "prompt"="Save In-Situ Preset", "button label"="Save" ("prompt"), "pattern (all files)"="*.xml", "pattern label"="In-Situ-XML") -> ("selected path"=w1615:path, "cancelled"=w1613:bool, "error out"=w1609:errorcluster)  [unwired: 7 in, 1 out]
        n801 = call <vilib>:"Clear Errors.vi"("error in (no error)"=w1609, "specific error code to clear (0: all)"=43) -> ("error out"=w1614:errorcluster)  [unwired: 4 in, 1 out]
        n802 = Bundle By Name(cluster=w1608, "Measure_IntegrationTime"=w1589, "Measure_FramesSpec"=w1588, "Frames_ForRef/Dark"=w1587, "Program Spin Coater"=w1586, "TabControlSpinType"=w1585, "Seconds2Spin_Norm"=w1584, "SecondsAftSpin_Norm"=w1583, "CalcFrames_Norm"=w1582, "PeriodicTime"=w1581, "DurationAfter"=w1580, "SpinAtEnd"=w1579, "Seconds2Spin_Short"=w1578, "SpinTime"=w1577, "CalculateFrames_Short"=w1576, "TimeDetect"=w1575, "WavelengthDetect"=w1574, "Threshold"=w1573, "WlLow"=w1572, "WlUp"=w1571, "TrimSpec"=w1570) -> (w1569:T20)
        n803 = Flatten To XML(6:w1569) -> (2:w1568:string)
        n804 = case shown="False" w1613 {
          tunnel: w1614 -> [w1624 w1633]
          tunnel: w1615 -> [w1620 _]
          tunnel: [w1621 w1633] -> _
          tunnel: w1568 -> [w1616 _]
          frame False {
            n805 = Open/Create/Replace File(file path (use dialog)=w1620, error in=w1624, operation (0:open)=T13."replace or create with confirmation") -> (refnum out=w1622:refnum<file>, cancelled=w1623:bool, error out=w1619:errorcluster)  [unwired: 3 in]
            n806 = call <vilib>:"Clear Errors.vi"("error in (no error)"=w1619, "specific error code to clear (0: all)"=43) -> ("error out"=w1618:errorcluster)  [unwired: 4 in, 1 out]
            n807 = case shown="False" w1623 {
              tunnel: w1618 -> [w1631 w1632]
              tunnel: w1622 -> [w1630 _]
              tunnel: [w1627 w1632] -> w1621
              tunnel: w1616 -> [w1626 _]
              frame False {
                n808 = Close File(refnum=w1630, error in=w1631) -> (path=w1629:path, error out=w1628:errorcluster)
                n809 = call-poly <vilib>:"Write to XML File.vi"("error in (no error)"=w1628, "XML Input"=w1626, "XML File Path"=w1629) -> ("error out"=w1627:errorcluster)  [unwired: 6 in, 2 out]
              }
              frame True {
              }
            }
          }
          frame True {
          }
        }
      }
      event "MeasureOpenPreset": Value Change {
        n810 = event-data() -> ()  [unwired: 1 in, 1 out]
        n811 = Current VI's Path() -> (path=w1641:path)
        n812 = Strip Path(path=w1641) -> (stripped path=w1642:path)  [unwired: 1 out]
        n813 = Build Path(base path=w1642, name or relative path=path "Presets" ("start path")) -> (appended path=w1639:path)
        n814 = call "File Dialog"("start path"=w1639, "prompt"="Open In-Situ Preset", "button label"="Open" ("prompt"), "pattern (all files)"="*.xml", "pattern label"="In-Situ-XML") -> ("selected path"=w1635:path, "cancelled"=w1636:bool, "error out"=w1637:errorcluster)  [unwired: 7 in, 1 out]
        n815 = call <vilib>:"Clear Errors.vi"("error in (no error)"=w1637, "specific error code to clear (0: all)"=43) -> ("error out"=w1634:errorcluster)  [unwired: 4 in, 1 out]
        n816 = case shown="False" w1636 {
          tunnel: w1635 -> [w1683 _]
          tunnel: w1634 -> [w1680 _]
          frame False {
            w1681 = T20 {"Measure_IntegrationTime"=0.0, "Measure_FramesSpec"=0.0, "Frames_ForRef/Dark"=0.0, "Program Spin Coater"=[], "TabControlSpinType"=0, "Seconds2Spin_Norm"=0.0, "SecondsAftSpin_Norm"=0.0, "CalcFrames_Norm"=FALSE, "PeriodicTime"=0.0, "DurationAfter"=0.0, "SpinAtEnd"=FALSE, "Seconds2Spin_Short"=0.0, "SpinTime"=0.0, "CalculateFrames_Short"=FALSE, "TimeDetect"=0.0, "WavelengthDetect"=0.0, "Threshold"=0.0, "WlLow"=0.0, "WlUp"=0.0, "TrimSpec"=FALSE}  # PresetCluster
            n817 = call-poly <vilib>:"Read From XML File.vi"("error in (no error)"=w1680, "XML File Path"=w1683) -> ("error out"=w1679:errorcluster, "XML Elements"=w1682:string)  [unwired: 7 in, 1 out]
            n818 = Unflatten From XML(xml string=w1682, type=w1681, error in (no error)=w1679) -> (value=w1678:T20)  [unwired: 1 out]
            n819 = Unbundle By Name(w1678) -> ("Measure_IntegrationTime"=w1676:dbl, "Measure_FramesSpec"=w1675:dbl, "Frames_ForRef/Dark"=w1674:dbl, "Program Spin Coater"=w1673:T2, "TabControlSpinType"=w1672:u32, "Seconds2Spin_Norm"=w1671:dbl, "SecondsAftSpin_Norm"=w1670:dbl, "CalcFrames_Norm"=w1667:bool, "PeriodicTime"=w1666:dbl, "DurationAfter"=w1664:dbl, "SpinAtEnd"=w1662:bool, "Seconds2Spin_Short"=w1661:dbl, "SpinTime"=w1660:dbl, "CalculateFrames_Short"=w1657:bool, "TimeDetect"=w1656:dbl, "WavelengthDetect"=w1655:dbl, "Threshold"=w1652:dbl, "WlLow"=w1651:dbl, "WlUp"=w1649:dbl, "TrimSpec"=w1647:bool)
            n820 = node(w1655) -> (w1653:dbl[unit])
            n821 = node(w1649) -> (w1648:dbl[unit])
            n822 = node(w1660) -> (w1658:dbl[unit])
            n823 = node(w1651) -> (w1650:dbl[unit])
            n824 = node(w1676) -> (w1677:dbl[unit])
            n825 = node(w1664) -> (w1663:dbl[unit])
            n826 = node(w1671) -> (w1669:dbl[unit])
            n827 = node(w1656) -> (w1654:dbl[unit])
            n828 = node(w1661) -> (w1659:dbl[unit])
            n829 = node(w1666) -> (w1665:dbl[unit])
            n830 = node(w1670) -> (w1668:dbl[unit])
            n831 = property on="Measure_IntegrationTime" class="DigNum (strict)"("Val(Sgnl)"=w1677) -> ()  [unwired: 2 in, 2 out]
            n832 = property on="Measure_FramesSpectrometer" class="DigNum (strict)"("Val(Sgnl)"=w1675) -> ()  [unwired: 2 in, 2 out]
            n833 = property on="Frames for Ref/Dark" class="DigNum (strict)"("Val(Sgnl)"=w1674) -> ()  [unwired: 2 in, 2 out]
            n834 = property on="Program Spin Coater" class="Arr (strict)"("Val(Sgnl)"=w1673) -> ()  [unwired: 2 in, 2 out]
            n835 = property on="Tab Control SpinType" class="TabCtl (strict)"("Val(Sgnl)"=w1672) -> ()  [unwired: 2 in, 2 out]
            n836 = property on="Seconds to Spin_Normal" class="DigNum (strict)"("Val(Sgnl)"=w1669) -> ()  [unwired: 2 in, 2 out]
            n837 = property on="Seconds after Spin" class="DigNum (strict)"("Val(Sgnl)"=w1668) -> ()  [unwired: 2 in, 2 out]
            n838 = property on="Calculate Frames_Normal" class="Bool (strict)"("Val(Sgnl)"=w1667) -> ()  [unwired: 2 in, 2 out]
            n839 = property on="periodic time" class="DigNum (strict)"("Val(Sgnl)"=w1665) -> ()  [unwired: 2 in, 2 out]
            n840 = property on="Duration after" class="DigNum (strict)"("Val(Sgnl)"=w1663) -> ()  [unwired: 2 in, 2 out]
            n841 = property on="Spin at end" class="Bool (strict)"("Val(Sgnl)"=w1662) -> ()  [unwired: 2 in, 2 out]
            n842 = property on="Seconds to Spin_Short" class="DigNum (strict)"("Val(Sgnl)"=w1659) -> ()  [unwired: 2 in, 2 out]
            n843 = property on="Spin Time" class="DigNum (strict)"("Val(Sgnl)"=w1658) -> ()  [unwired: 2 in, 2 out]
            n844 = property on="Calculate Frames_Short" class="Bool (strict)"("Val(Sgnl)"=w1657) -> ()  [unwired: 2 in, 2 out]
            n845 = property on="Time Detect" class="DigNum (strict)"("Val(Sgnl)"=w1654) -> ()  [unwired: 2 in, 2 out]
            n846 = property on="Wavelenght Detect" class="DigNum (strict)"("Val(Sgnl)"=w1653) -> ()  [unwired: 2 in, 2 out]
            n847 = property on="Threshold" class="DigNum (strict)"("Val(Sgnl)"=w1652) -> ()  [unwired: 2 in, 2 out]
            n848 = property on="WlLow" class="DigNum (strict)"("Val(Sgnl)"=w1650) -> ()  [unwired: 2 in, 2 out]
            n849 = property on="WlUp" class="DigNum (strict)"("Val(Sgnl)"=w1648) -> ()  [unwired: 2 in, 2 out]
            n850 = property on="TrimSpec" class="Bool (strict)"("Val(Sgnl)"=w1647) -> ()  [unwired: 2 in, 2 out]
          }
          frame True {
          }
        }
      }
    }
  }
  n851 = while {
    shift-right: [w1688] -> _
    shift-left: w5 -> [w1692]
    shift-right: [w1689] -> w14
    shift-left: w16 -> [w1691]
    shift-right: [w1686] -> w13
    shift-left: w12 -> [w1687]
    shift-right: [w1684] -> _
    shift-left: w15 -> [w1685]
    stop <- w1690 stop-if-true
    # "Consumer Devices"
    n852 = case shown="No Error" w1692 {
      selector: w1692 -> [w1705 w2599]
      tunnel: w1691 -> [w1706 w2600]
      tunnel: [w1702 _] -> w1690
      tunnel: [w1701 w2600] -> w1689
      tunnel: [w1699 w2596] -> w1688
      tunnel: w1687 -> [w1697 w2594]
      tunnel: [w1698 w2594] -> w1686
      tunnel: w1685 -> [w1696 w2595]
      tunnel: [w1695 w2595] -> w1684
      frame No Error {
        n853 = Dequeue Element(queue=w1706, timeout in ms (-1)=10, error in (no error)=w1705) -> (queue out=w1704:refnum<queue>, element=w1694:T11, error out=w1700:errorcluster)  [unwired: 1 out]
        n854 = Unbundle By Name(w1694) -> ("QueueAction"=w1703:T12)
        n855 = case shown="\"Abort\"" w1703 {
          tunnel: w1704 -> [w1711 w1732 w1773 w1796 w1807 w1862 w1881 w1906 w1917 w1940 w1947 w1966 w2031 w2088 w2119 w2138 w2153 w2163 w2175 w2176 w2198 w2222 w2229 w2236 w2248 w2254 w2260 w2272 w2279 w2286 w2295 w2341 w2436 w2539 w2555 w2565]
          tunnel: [_ _ w1775 _ _ _ _ _ _ _ _ _ _ _ _ _ _ _ _ _ _ _ _ _ _ _ _ _ _ _ _ _ _ _ _ _] -> w1702
          tunnel: [w1711 w1732 w1758 w1783 w1803 w1862 w1881 w1906 w1918 w1940 w1947 w1966 w2031 w2088 w2119 w2138 w2153 w2163 w2175 w2176 w2198 w2222 w2229 w2236 w2248 w2254 w2260 w2272 w2279 w2286 w2295 w2303 w2362 w2499 w2546 w2568] -> w1701
          tunnel: w1700 -> [w1710 w1731 w1757 w1795 w1818 w1863 w1880 w1905 w1913 w1943 w1951 w1963 w2019 w2098 w2117 w2128 w2144 w2160 w2171 w2183 w2201 w2216 w2226 w2234 w2243 w2251 w2257 w2263 w2275 w2282 w2288 w2297 w2400 w2503 w2554 w2564]
          tunnel: [w1710 w1731 w1756 w1777 w1806 w1857 w1879 w1904 w1911 w1941 w1948 w1954 w1973 w2092 w2116 w2123 w2140 w2158 w2165 w2186 w2200 w2213 w2225 w2232 w2242 w2250 w2256 w2262 w2274 w2281 w2287 w2304 w2361 w2492 w2545 w2569] -> w1699
          tunnel: [w1708 w1729 w1755 w1800 w1804 w1859 w1872 w1886 w1922 w1939 w1946 w1957 w2025 w2100 w2120 w2132 w2147 w2154 w2167 w2188 w2199 w2221 w2231 w2240 w2246 w2255 w2261 w2271 w2278 w2285 w2290 w2312 w2409 w2514 w2553 w2585] -> w1698
          tunnel: w1697 -> [w1708 w1729 w1755 w1800 w1805 w1859 w1871 w1895 w1923 w1939 w1946 w1958 w2026 w2100 w2120 w2135 w2150 w2154 w2169 w2188 w2199 w2221 w2231 w2240 w2246 w2255 w2261 w2271 w2278 w2285 w2291 w2312 w2409 w2514 w2553 w2585]
          tunnel: w1696 -> [w1709 w1730 w1754 w1799 w1815 w1861 w1878 w1903 w1916 w1938 w1950 w1959 w2010 w2091 w2113 w2131 w2146 w2157 w2164 w2185 w2194 w2215 w2230 w2239 w2245 w2253 w2259 w2270 w2277 w2284 w2289 w2344 w2439 w2542 w2552 w2584]
          tunnel: [w1709 w1730 w1754 w1799 w1809 w1860 w1878 w1903 w1915 w1936 w1945 w1959 w2010 w2089 w2114 w2130 w2145 w2155 w2164 w2187 w2192 w2212 w2230 w2239 w2245 w2253 w2259 w2270 w2277 w2284 w2289 w2344 w2439 w2542 w2552 w2584] -> w1695
          tunnel: w1694 -> [_ w1725 _ _ w1802 _ w1870 w1897 w1909 _ _ w1965 w2030 w2095 w2121 _ _ w2161 _ _ _ w2220 w2224 w2238 w2247 _ _ w2268 _ _ _ _ w2385 _ w2543 w2559]
          frame "TimeOut", Default {
            n856 = property on="Action" class="Str"("Value"="TimeOut" ("Action")) -> ()  [unwired: 2 in, 2 out]
          }
          frame "Wait" {
            n857 = flat-sequence {
              tunnel: [w1743] -> w1726
              tunnel: w1725 -> [w1743]
              tunnel: [w1742] -> w1723
              frame #0 {
                n858 = Tick Count (ms)() -> (millisecond timer value=w1742:u32)
              }
            }
            n859 = Unbundle By Name(w1726) -> ("Numeric 1"=w1717:dbl)
            n860 = property on="SS:PeriodicTime" class="DigNum (strict)"() -> ("Value"=w1719:dbl[unit])  [unwired: 2 in, 2 out]
            n861 = Multiply(x=w1717, y=1000.0) -> (x*y=w1721:dbl)
            n862 = node(w1717) -> (w1718:dbl[unit])
            n863 = property on="SS_StepsLeft" class="DigNum (strict)"() -> ("Value"=w1716:dbl)  [unwired: 2 in, 2 out]
            n864 = Round Toward -Infinity(1:w1717) -> (0:w1720:dbl)
            n865 = Subtract(x=w1719, y=w1718) -> (x-y=w1713:dbl[unit])
            n866 = Decrement(x=w1716) -> (x-1=w1715:dbl)
            n867 = Multiply(x=w1715, y=w1719) -> (x*y=w1714:dbl[unit])
            n868 = Add(x=w1714, y=w1713) -> (x+y=w1712:dbl[unit])
            n869 = for {
              N: w1720 -> [_]
              tunnel: 1000.0 ("y") -> [w1744]
              tunnel: [w1752] -> w1724
              tunnel: w1712 -> [w1749]
              i -> [w1747]
              stop <- w1752 stop-if-true
              n870 = Increment(x=w1747) -> (x+1=w1745:i32)
              n871 = Multiply(x=w1744, y=w1745) -> (x*y=w1746:dbl)
              n872 = node(w1746) -> (w1748:dbl[unit])
              n873 = property on="Stop Button" class="Bool (strict)"() -> ("Value"=w1752:bool)  [unwired: 2 in, 2 out]
              n874 = Wait (ms)(milliseconds to wait=w1744) -> (millisecond timer value=w1750:u32)
              n875 = Subtract(x=w1749, y=w1748) -> (x-y=w1751:dbl[unit])
              n876 = flat-sequence {
                tunnel: w1751 -> [w1753]
                tunnel: w1750 -> [_]
                frame #0 {
                  n877 = property on="SS_TimePrediction" class="DigNum (strict)"("Value"=w1753) -> ()  [unwired: 2 in, 2 out]
                }
              }
            }
            n878 = property on="Action" class="Str"("Value"="Wait" ("Action")) -> ()  [unwired: 2 in, 2 out]
            n879 = case shown="False" w1724 {
              tunnel: w1723 -> [w1738 _]
              tunnel: w1721 -> [w1733 _]
              frame False {
                n880 = flat-sequence {
                  tunnel: [w1741] -> w1739
                  frame #0 {
                    n881 = Tick Count (ms)() -> (millisecond timer value=w1741:u32)
                  }
                }
                n882 = Subtract(x=w1739, y=w1738) -> (x-y=w1737:u32)
                n883 = To Double Precision Float(number=w1737) -> (double precision float=w1734:dbl)
                n884 = Subtract(x=w1733, y=w1734) -> (x-y=w1735:dbl)
                n885 = Greater Than 0?(x=w1735) -> (x > 0?=w1736:bool)
                n886 = case shown="True" w1736 {
                  tunnel: w1735 -> [_ w1740]
                  frame False {
                  }
                  frame True {
                    n887 = Wait (ms)(milliseconds to wait=w1740) -> ()  [unwired: 1 out]
                  }
                }
              }
              frame True {
                # "If Aborted, do nothing"
              }
            }
          }
          frame "Close_Program" {
            w1774 = T11 {"QueueAction"=enum."TimeOut", "Numeric 1"=0.0, "Numeric 2"=0.0, "Boolean 1"=FALSE, "Boolean 2"=FALSE, "Spin Program"=[], "Spin Prg v07"=[], "Time Stamp"=timestamp(0 s since 1904-01-01), "TabControl"=enum."Measure"}  # Device Queue
            n888 = Bundle By Name(cluster=w1774, "QueueAction"=DeviceQueue_Action."Spectrometer_Close") -> (w1769:T11)
            n889 = Bundle By Name(cluster=w1769, "QueueAction"=DeviceQueue_Action."Laser_Close") -> (w1767:T11)
            n890 = Bundle By Name(cluster=w1767, "QueueAction"=DeviceQueue_Action."Arduino_Close") -> (w1761:T11)
            n891 = Enqueue Element(queue=w1773, element=w1769, error in (no error)=w1757) -> (queue out=w1771:refnum<queue>, error out=w1766:errorcluster)  [unwired: 1 in, 1 out]
            n892 = Bundle By Name(cluster=w1761, "QueueAction"=DeviceQueue_Action."Close_Program") -> (w1759:T11)
            n893 = Enqueue Element(queue=w1771, element=w1767, error in (no error)=w1766) -> (queue out=w1765:refnum<queue>, error out=w1764:errorcluster)  [unwired: 1 in, 1 out]
            n894 = Enqueue Element(queue=w1765, element=w1761, error in (no error)=w1764) -> (queue out=w1763:refnum<queue>, error out=w1762:errorcluster)  [unwired: 1 in, 1 out]
            n895 = Enqueue Element(queue=w1763, element=w1759, error in (no error)=w1762) -> (queue out=w1758:refnum<queue>, error out=w1756:errorcluster)  [unwired: 1 in, 1 out]
            n896 = First Call?() -> (First Call?: T/F=w1776:bool)
            n897 = Not(x=w1776) -> (.not. x?=w1775:bool)
          }
          frame "Abort" {
            w1798 = T11 {"QueueAction"=enum."TimeOut", "Numeric 1"=0.0, "Numeric 2"=0.0, "Boolean 1"=FALSE, "Boolean 2"=FALSE, "Spin Program"=[], "Spin Prg v07"=[], "Time Stamp"=timestamp(0 s since 1904-01-01), "TabControl"=enum."Measure"}  # Device Queue
            n898 = Flush Queue(queue=w1796, error in (no error)=w1795) -> (queue out=w1794:refnum<queue>, error out=w1793:errorcluster)  [unwired: 1 out]
            n899 = Bundle By Name(cluster=w1798, "QueueAction"=DeviceQueue_Action."Spectrometer_StopMeasurement") -> (w1790:T11)
            n900 = Bundle By Name(cluster=w1790, "QueueAction"=DeviceQueue_Action."Arduino_StopSpin") -> (w1786:T11)
            n901 = Enqueue Element(queue=w1794, element=w1790, error in (no error)=w1793) -> (queue out=w1792:refnum<queue>, error out=w1791:errorcluster)  [unwired: 1 in, 1 out]
            n902 = Bundle By Name(cluster=w1786, "QueueAction"=DeviceQueue_Action."Measure_Stop") -> (w1781:T11)
            n903 = Enqueue Element(queue=w1792, element=w1786, error in (no error)=w1791) -> (queue out=w1788:refnum<queue>, error out=w1787:errorcluster)  [unwired: 1 in, 1 out]
            n904 = Bundle By Name(cluster=w1781, "QueueAction"=DeviceQueue_Action."Spectrometer_SetTriggerMode", "Numeric 1"=0.0) -> (w1778:T11)
            n905 = Enqueue Element(queue=w1788, element=w1781, error in (no error)=w1787) -> (queue out=w1784:refnum<queue>, error out=w1782:errorcluster)  [unwired: 1 in, 1 out]
            n906 = Enqueue Element(queue=w1784, element=w1778, error in (no error)=w1782) -> (queue out=w1783:refnum<queue>, error out=w1777:errorcluster)  [unwired: 1 in, 1 out]
          }
          frame "Spectrometer_Init" {
            n907 = call-dynamic "Init.vi"("error in (no error)"=w1818, "Variant"=0, "Avantes in"=refnum<class "Avantes.lvclass"> refnum ("Avantes.lvclass")) -> ("error out"=w1817:errorcluster, "Avantes out"=w1816:refnum<class "Avantes.lvclass">)  [unwired: 7 in]
            n908 = call-dynamic "IsInit.vi"("error in (no error)"=w1817, "Avantes in"=w1816) -> ("error out"=w1813:errorcluster, "Is Init?"=w1812:bool, "Avantes out"=w1814:refnum<class "Avantes.lvclass">)  [unwired: 7 in]
            n909 = Unbundle By Name(w1802) -> ("TabControl"=w1801:T10)
            n910 = property on="Spectromter" class="Bool (strict)"("Value"=w1812) -> ()  [unwired: 2 in, 2 out]
            n911 = property on="Init_Spectrometer" class="Bool (strict)"("Value"=w1812) -> ()  [unwired: 2 in, 2 out]
            n912 = call-dynamic "Set_ExposurePerFrame.vi"("error in (no error)"=w1813, "Exposure per Frame"=1, "Avantes in"=w1814) -> ("error out"=w1808:errorcluster, "Avantes out"=w1811:refnum<class "Avantes.lvclass">)  [unwired: 7 in]
            n913 = case shown="True" w1812 {
              tunnel: w1811 -> [_ w1841]
              tunnel: w1808 -> [w1824 w1839]
              tunnel: [refnum<class "Abstract_CCD.lvclass"> refnum ("Abstract_CCD.lvclass") w1840] -> w1810
              tunnel: w1807 -> [w1822 w1851]
              tunnel: [w1824 w1844] -> w1806
              tunnel: w1805 -> [w1823 w1836]
              tunnel: [w1823 w1834] -> w1804
              tunnel: [w1822 w1832] -> w1803
              tunnel: w1802 -> [_ w1829]
              tunnel: w1801 -> [_ w1828]
              frame False {
              }
              frame True {
                w1842 = T8 {"QueueAction"=enum."TimeOut", "Data"=[], "Data_Raw"=[], "Data_Dark"=[], "Data_Ref"=[], "Device Information"=[], "Numeric Control"=0.0, "Boolean"=FALSE, "Wavelength"=[], "Time"=[], "Time Stamp"=timestamp(0 s since 1904-01-01), "Numeric Control 2"=0.0, "TabControl"=enum."Measure", "Numeric Control 3"=0.0}  # DataQueue
                n914 = case shown="\"Spectral Stability\"" w1828 {
                  tunnel: [w1853 w1855] -> w1827
                  tunnel: [w1852 w1854] -> w1826
                  frame "Measure", Default {
                    n915 = property on="Measure_IntegrationTime" class="DigNum (strict)"() -> ("Value"=w1853:dbl[unit])  [unwired: 2 in, 2 out]
                    n916 = property on="Measure_FramesSpectrometer" class="DigNum (strict)"() -> ("Value"=w1852:dbl)  [unwired: 2 in, 2 out]
                  }
                  frame "Spectral Stability" {
                    n917 = property on="SpectralStability_FramesSpectrometer" class="DigNum (strict)"() -> ("Value"=w1854:dbl)  [unwired: 2 in, 2 out]
                    n918 = property on="SpectralStability_IntegrationTime" class="DigNum (strict)"() -> ("Value"=w1855:dbl[unit])  [unwired: 2 in, 2 out]
                  }
                }
                n919 = call-dynamic "Get_WavelengthAxis.vi"("error in (no error)"=w1839, "Avantes in"=w1841) -> ("error out"=w1838:errorcluster, "lambda"=w1833:dbl[unit][], "Avantes out"=w1840:refnum<class "Avantes.lvclass">)  [unwired: 7 in]
                n920 = Unbundle(w1838) -> ("status"=w1837:bool)  [unwired: 2 out]
                n921 = property on="Error_Spectromter" class="Bool (strict)"("Value"=w1837) -> ()  [unwired: 2 in, 2 out]
                n922 = property on="Calculate Frames_Normal" class="Bool (strict)"() -> ("Value"=w1830:bool)  [unwired: 2 in, 2 out]
                n923 = Bundle By Name(cluster=w1842, "QueueAction"=DataQueue_Action."Set_Wavelength", "Wavelength"=w1833) -> (w1843:T8)
                n924 = node(w1827) -> (w1849:dbl)
                n925 = Bundle By Name(cluster=w1829, "QueueAction"=DeviceQueue_Action."Spectrometer_SetIntegrationTime", "Numeric 1"=w1849, "Boolean 1"=w1830) -> (w1847:T11)
                n926 = Enqueue Element(queue=w1836, element=w1843) -> (queue out=w1834:refnum<queue>)  [unwired: 2 in, 2 out]
                n927 = Bundle By Name(cluster=w1847, "QueueAction"=DeviceQueue_Action."Spectrometer_SetFrames", "Numeric 1"=w1826) -> (w1846:T11)
                n928 = Enqueue Element(queue=w1851, element=w1847, error in (no error)=w1839) -> (queue out=w1848:refnum<queue>, error out=w1845:errorcluster)  [unwired: 1 in, 1 out]
                n929 = Enqueue Element(queue=w1848, element=w1846, error in (no error)=w1845) -> (queue out=w1832:refnum<queue>, error out=w1844:errorcluster)  [unwired: 1 in, 1 out]
              }
            }
            n930 = Bundle By Name(cluster=w1815, "Abstract_CCD.lvclass"=w1810) -> (w1809:T6)
          }
          frame "Spectrometer_Close" {
            n931 = property on="Spectromter" class="Bool (strict)"("Value"=FALSE ("Spectromter")) -> ()  [unwired: 2 in, 2 out]
            n932 = Unbundle By Name(w1861) -> ("Abstract_CCD.lvclass"=w1864:refnum<class "Abstract_CCD.lvclass">)
            n933 = flat-sequence {
              tunnel: [refnum<class "Abstract_CCD.lvclass"> refnum ("Abstract_CCD.lvclass")] -> w1858
              tunnel: w1857 -> [_]
              frame #0 {
              }
            }
            n934 = call-dynamic "Close.vi"("error in (no error)"=w1863, "Abstract_CCD in"=w1864) -> ("error out"=w1857:errorcluster)  [unwired: 8 in, 1 out]
            n935 = Bundle By Name(cluster=w1861, "Abstract_CCD.lvclass"=w1858) -> (w1860:T6)
          }
          frame "Spectrometer_Measure" {
            w1883 = T8 {"QueueAction"=enum."TimeOut", "Data"=[], "Data_Raw"=[], "Data_Dark"=[], "Data_Ref"=[], "Device Information"=[], "Numeric Control"=0.0, "Boolean"=FALSE, "Wavelength"=[], "Time"=[], "Time Stamp"=timestamp(0 s since 1904-01-01), "Numeric Control 2"=0.0, "TabControl"=enum."Measure", "Numeric Control 3"=0.0}  # DataQueue
            n936 = Unbundle By Name(w1878) -> ("Abstract_CCD.lvclass"=w1882:refnum<class "Abstract_CCD.lvclass">)
            n937 = Unbundle By Name(w1870) -> ("Time Stamp"=w1867:timestamp, "TabControl"=w1868:T10)
            n938 = Get Date/Time In Seconds() -> (seconds since 1Jan1904=w1866:timestamp)
            n939 = Subtract(x=w1866, y=w1867) -> (x-y=w1869:dbl)
            n940 = call-dynamic "Measure.vi"("error in (no error)"=w1880, "Abstract_CCD in"=w1882) -> ("error out"=w1879:errorcluster, "Data Raw"=w1875:T14, "Data"=w1876:T14, "Darkspec"=w1874:T14, "Time"=w1873:dbl[])  [unwired: 3 in, 2 out]
            n941 = Bundle By Name(cluster=w1883, "QueueAction"=DataQueue_Action."Spectrometer_Measure", "Data"=w1876, "Data_Raw"=w1875, "Data_Dark"=w1874, "Time"=w1873, "Time Stamp"=w1867, "Numeric Control 2"=w1869, "TabControl"=w1868) -> (w1884:T8)
            n942 = Enqueue Element(queue=w1871, element=w1884) -> (queue out=w1872:refnum<queue>)  [unwired: 2 in, 2 out]
          }
          frame "Spectrometer_MeasureAdvanced" {
            w1894 = T8 {"QueueAction"=enum."TimeOut", "Data"=[], "Data_Raw"=[], "Data_Dark"=[], "Data_Ref"=[], "Device Information"=[], "Numeric Control"=0.0, "Boolean"=FALSE, "Wavelength"=[], "Time"=[], "Time Stamp"=timestamp(0 s since 1904-01-01), "Numeric Control 2"=0.0, "TabControl"=enum."Measure", "Numeric Control 3"=0.0}  # DataQueue
            w1908 = T8 {"QueueAction"=enum."TimeOut", "Data"=[], "Data_Raw"=[], "Data_Dark"=[], "Data_Ref"=[], "Device Information"=[], "Numeric Control"=0.0, "Boolean"=FALSE, "Wavelength"=[], "Time"=[], "Time Stamp"=timestamp(0 s since 1904-01-01), "Numeric Control 2"=0.0, "TabControl"=enum."Measure", "Numeric Control 3"=0.0}  # DataQueue
            n943 = Unbundle By Name(w1903) -> ("Abstract_CCD.lvclass"=w1907:refnum<class "Abstract_CCD.lvclass">)
            n944 = Unbundle By Name(w1897) -> ("Time Stamp"=w1896:timestamp)
            n945 = call-dynamic "Measure.vi"("error in (no error)"=w1905, "Abstract_CCD in"=w1907) -> ("error out"=w1904:errorcluster, "Data Raw"=w1900:T14, "Data"=w1901:T14, "Darkspec"=w1899:T14, "Time"=w1898:dbl[])  [unwired: 3 in, 2 out]
            n946 = Bundle By Name(cluster=w1894, "QueueAction"=DataQueue_Action."Measure_SpectrumAdvanced") -> (w1892:T8)
            n947 = Bundle By Name(cluster=w1908, "QueueAction"=DataQueue_Action."Spectrometer_Measure", "Data"=w1901, "Data_Raw"=w1900, "Data_Dark"=w1899, "Time"=w1898, "Time Stamp"=w1896) -> (w1889:T8)
            n948 = Enqueue Element(queue=w1895, element=w1892) -> (queue out=w1891:refnum<queue>)  [unwired: 2 in, 2 out]
            n949 = Enqueue Element(queue=w1891, element=w1889) -> (queue out=w1890:refnum<queue>)  [unwired: 2 in, 2 out]
            n950 = Bundle By Name(cluster=w1889, "QueueAction"=DataQueue_Action."Stop_Measurement") -> (w1887:T8)
            n951 = property on="Action" class="Str"("Value"="Measure Spectra A" ("Action")) -> ()  [unwired: 2 in, 2 out]
            n952 = Enqueue Element(queue=w1890, element=w1887) -> (queue out=w1886:refnum<queue>)  [unwired: 2 in, 2 out]
          }
          frame "Spectrometer_Preview" {
            w1924 = T8 {"QueueAction"=enum."TimeOut", "Data"=[], "Data_Raw"=[], "Data_Dark"=[], "Data_Ref"=[], "Device Information"=[], "Numeric Control"=0.0, "Boolean"=FALSE, "Wavelength"=[], "Time"=[], "Time Stamp"=timestamp(0 s since 1904-01-01), "Numeric Control 2"=0.0, "TabControl"=enum."Measure", "Numeric Control 3"=0.0}  # DataQueue
            n953 = Unbundle By Name(w1916) -> ("Abstract_CCD.lvclass"=w1914:refnum<class "Abstract_CCD.lvclass">)
            n954 = Unbundle By Name(w1909) -> ("TabControl"=w1910:T10)
            n955 = call-dynamic "Measure.vi"("error in (no error)"=w1913, "Abstract_CCD in"=w1914) -> ("error out"=w1911:errorcluster, "Data Raw"=w1921:T14, "Abstract_CCD out"=w1912:refnum<class "Abstract_CCD.lvclass">)  [unwired: 3 in, 4 out]
            n956 = case shown="\"Measure\"" w1910 {
              tunnel: [FALSE ("Value") w1928 w1929] -> w1919
              tunnel: w1911 -> [_ w1927 _]
              frame Default {
              }
              frame "Measure" {
                n957 = property on="Measure_Preview" class="Bool (strict)"(error in=w1927) -> ("Value"=w1928:bool)  [unwired: 1 in, 2 out]
              }
              frame "Spectral Stability" {
                n958 = property on="SpectralStability_Preview" class="Bool (strict)"() -> ("Value"=w1929:bool)  [unwired: 2 in, 2 out]
              }
            }
            n959 = case shown="True" w1919 {
              tunnel: [w1930 w1933] -> w1918
              tunnel: w1917 -> [w1930 w1932]
              tunnel: w1909 -> [_ w1931]
              frame False {
              }
              frame True {
                n960 = Bundle By Name(cluster=w1931, "QueueAction"=DeviceQueue_Action."Spectrometer_Preview") -> (w1934:T11)
                n961 = Enqueue Element(queue=w1932, element=w1934) -> (queue out=w1933:refnum<queue>)  [unwired: 2 in, 2 out]
              }
            }
            n962 = Bundle By Name(cluster=w1924, "Data_Raw"=w1921, "QueueAction"=DataQueue_Action."Spectrometer_Preview", "TabControl"=w1910) -> (w1925:T8)
            n963 = Enqueue Element(queue=w1923, element=w1925) -> (queue out=w1922:refnum<queue>)  [unwired: 2 in, 2 out]
            n964 = Bundle By Name(cluster=w1916, "Abstract_CCD.lvclass"=w1912) -> (w1915:T6)
          }
          frame "Spectrometer_StartMeasurement" {
            n965 = Unbundle By Name(w1938) -> ("Abstract_CCD.lvclass"=w1942:refnum<class "Abstract_CCD.lvclass">)
            n966 = call-dynamic "StartMeasure.vi"("error in (no error)"=w1943, "Frames"=-1, "Abstract_CCD in"=w1942) -> ("error out"=w1941:errorcluster, "Abstract_CCD out"=w1937:refnum<class "Abstract_CCD.lvclass">)  [unwired: 7 in]
            n967 = Bundle By Name(cluster=w1938, "Abstract_CCD.lvclass"=w1937) -> (w1936:T6)
          }
          frame "Spectrometer_StopMeasurement" {
            n968 = Unbundle By Name(w1950) -> ("Abstract_CCD.lvclass"=w1952:refnum<class "Abstract_CCD.lvclass">)
            n969 = call-dynamic "StopMeasurement.vi"("error in (no error)"=w1951, "Abstract_CCD in"=w1952) -> ("error out"=w1948:errorcluster, "Abstract_CCD out"=w1949:refnum<class "Abstract_CCD.lvclass">)  [unwired: 8 in]
            n970 = Bundle By Name(cluster=w1950, "Abstract_CCD.lvclass"=w1949) -> (w1945:T6)
          }
          frame "Spectrometer_GetData" {
            w1962 = T8 {"QueueAction"=enum."TimeOut", "Data"=[], "Data_Raw"=[], "Data_Dark"=[], "Data_Ref"=[], "Device Information"=[], "Numeric Control"=0.0, "Boolean"=FALSE, "Wavelength"=[], "Time"=[], "Time Stamp"=timestamp(0 s since 1904-01-01), "Numeric Control 2"=0.0, "TabControl"=enum."Measure", "Numeric Control 3"=0.0}  # DataQueue
            n971 = Unbundle By Name(w1959) -> ("Abstract_CCD.lvclass"=w1964:refnum<class "Abstract_CCD.lvclass">)
            n972 = Unbundle By Name(w1965) -> ("Numeric 1"=w1956:dbl)
            n973 = call-dynamic "Measure_GetData.vi"("error in (no error)"=w1963, "SpectraCount"=w1956, "Abstract_CCD in"=w1964) -> ("error out"=w1954:errorcluster, "Data_Raw"=w1953:T14, "Time"=w1955:dbl[])  [unwired: 5 in, 1 out]
            n974 = Bundle By Name(cluster=w1962, "QueueAction"=DataQueue_Action."Spectrometer_Measure", "Data_Raw"=w1953, "Time"=w1955) -> (w1961:T8)
            n975 = Enqueue Element(queue=w1958, element=w1961) -> (queue out=w1957:refnum<queue>)  [unwired: 2 in, 2 out]
          }
          frame "Spectrometer_GetData_Short" {
            w2013 = 0 ("index (page)")
            w2008 = nan
            w2029 = T8 {"QueueAction"=enum."TimeOut", "Data"=[], "Data_Raw"=[], "Data_Dark"=[], "Data_Ref"=[], "Device Information"=[], "Numeric Control"=0.0, "Boolean"=FALSE, "Wavelength"=[], "Time"=[], "Time Stamp"=timestamp(0 s since 1904-01-01), "Numeric Control 2"=0.0, "TabControl"=enum."Measure", "Numeric Control 3"=0.0}  # DataQueue
            # "Frames"
            # "Start Time + Offset"
            n976 = Unbundle By Name(w2010) -> ("Abstract_CCD.lvclass"=w2018:refnum<class "Abstract_CCD.lvclass">)
            n977 = local read "Seconds to Spin_Short"() -> (w1993:dbl[unit])
            n978 = Unbundle By Name(w2030) -> ("Numeric 2"=w1984:dbl)
            n979 = call <vilib>:"High Resolution Relative Seconds.vi"() -> ("relative seconds"=w2024:dbl)
            n980 = node("Time Detect") -> (w2023:dbl)
            n981 = To Long Integer(number=w1984) -> (32bit integer=w1979:i32)
            n982 = node(w1993) -> (w2022:dbl)
            n983 = call-dynamic "Measure_GetData_SpectraOutput.vi"("error in (no error)"=w2019, "Abstract_CCD in"=w2018) -> ("error out"=w2021:errorcluster, "Spectra"=w2014:dbl[], "Abstract_CCD out"=w2020:refnum<class "Abstract_CCD.lvclass">, "Time"=w2005:dbl)  [unwired: 6 in]
            n984 = Compound Arithmetic op=ADD(w2024, w2022, w2023) -> (w2011:dbl)
            n985 = Initialize Array(w2008, w1979) -> (w2007:dbl[])
            n986 = Array Size(array=w2014) -> (size(s)=w2017:i32)
            n987 = Initialize Array(w2008, w1979, 1 ("index"), w2017) -> (w2015:dbl[][][])
            n988 = Replace Array Subset(array=w2007, new element=w2005, index=0) -> (w2004:dbl[])
            n989 = Replace Array Subset(array=w2015, new element=w2014, index (dim 0)=w2013, index (dim 1)=w2013) -> (w2012:dbl[][][])  [unwired: 1 in]
            n990 = while {
              shift-right: [w2084] -> w1989
              shift-left: w2021 -> [w2085]
              shift-right: [w2081] -> w1990
              shift-left: w2012 -> [w2083]
              tunnel: w2011 -> [w2080]
              shift-right: [w2077] -> w1991
              shift-left: w2004 -> [w2079]
              tunnel: [w2074] -> w1992
              tunnel: [w2072] -> w1987
              shift-right: [w2071] -> w1988
              shift-left: w2020 -> [w2086]
              i -> [w2073]
              stop <- w2075 stop-if-true
              # "Wait for correct Time"
              n991 = call <vilib>:"High Resolution Relative Seconds.vi"() -> ("relative seconds"=w2076:dbl)
              n992 = call-dynamic "Measure_GetData_SpectraOutput.vi"("error in (no error)"=w2085, "Abstract_CCD in"=w2086) -> ("error out"=w2084:errorcluster, "Spectra"=w2074:dbl[], "Abstract_CCD out"=w2071:refnum<class "Abstract_CCD.lvclass">, "Time"=w2078:dbl)  [unwired: 6 in]
              n993 = Greater?(x=w2076, y=w2080) -> (0:w2075:bool)
              n994 = Increment(x=w2073) -> (x+1=w2072:i32)
              n995 = Replace Array Subset(array=w2079, new element=w2078, index=w2072) -> (w2077:dbl[])
              n996 = Replace Array Subset(array=w2083, new element=w2074, index (dim 0)=w2072, index (dim 1)=0 ("disabled index (row)")) -> (w2081:dbl[][][])  [unwired: 1 in]
            }
            n997 = local read "WL-Det\nPos"() -> (w1986:i32)
            n998 = Increment(x=w1987) -> (x+1=w1972:i32)
            n999 = Index Array(array=w1992, index=w1986) -> (element=w1985:dbl)
            n1000 = while {
              shift-right: [w2064] -> w1981
              shift-left: w1991 -> [w2066]
              shift-right: [w2062] -> w1982
              shift-left: w1990 -> [w2063]
              shift-right: [w2054] -> w1971
              shift-left: w1989 -> [w2070]
              tunnel: w1972 -> [w2068]
              tunnel: w1986 -> [w2056]
              tunnel: w1979 -> [w2053]
              tunnel: [w2048] -> w1977
              tunnel: [w2047] -> w1968
              shift-right: [w2049] -> w1980
              shift-left: w1988 -> [w2069]
              i -> [w2067]
              stop <- w2050 stop-if-true
              # "Wait for threshold"
              n1001 = call-dynamic "Measure_GetData_SpectraOutput.vi"("error in (no error)"=w2070, "Abstract_CCD in"=w2069) -> ("error out"=w2054:errorcluster, "Spectra"=w2057:dbl[], "Abstract_CCD out"=w2049:refnum<class "Abstract_CCD.lvclass">, "Time"=w2065:dbl)  [unwired: 6 in]
              n1002 = Add(x=w2068, y=w2067) -> (x+y=w2048:i32)
              n1003 = Index Array(array=w2057, index=w2056) -> (element=w2058:dbl)
              n1004 = Replace Array Subset(array=w2066, new element=w2065, index=w2048) -> (w2064:dbl[])
              n1005 = Replace Array Subset(array=w2063, new element=w2057, index (dim 0)=w2048, index (dim 1)=0 ("disabled index (row)")) -> (w2062:dbl[][][])  [unwired: 1 in]
              n1006 = Divide(x=w2058, y="Reference\nValue") -> (x/y=w2059:dbl)
              n1007 = Less?(x=w2059, y="Threshold") -> (x < y?=w2052:bool)
              n1008 = Equal?(x=w2053, y=w2048) -> (x = y?=w2051:bool)
              n1009 = call <vilib>:"High Resolution Relative Seconds.vi"() -> ("relative seconds"=w2047:dbl)
              n1010 = Or(x=w2051, y=w2052) -> (x .or. y?=w2050:bool)
            }
            n1011 = local write "Reference\nValue"(w1985) -> ()
            n1012 = Unbundle By Name(w2010) -> ("SpinCoater.lvclass"=w1983:refnum<class "SpinCoater.lvclass">)
            n1013 = Subtract(x=w1979, y=w1977) -> (x-y=w1978:i32)
            n1014 = Increment(x=w1977) -> (x+1=w1975:i32)
            n1015 = call-dynamic "Stop_Short.vi"("error in (no error)"=w1971, "SpinCoater in"=w1983) -> ("error out"=w1970:errorcluster)  [unwired: 8 in, 1 out]
            n1016 = for {
              N: w1978 -> [_]
              shift-right: [w2042] -> w1976
              shift-left: w1981 -> [w2041]
              shift-right: [w2038] -> w1974
              shift-left: w1982 -> [w2039]
              tunnel: w1975 -> [w2044]
              shift-right: [w2034] -> w1973
              shift-left: w1971 -> [w2046]
              shift-right: [w2033] -> _
              shift-left: w1980 -> [w2045]
              i -> [w2043]
              n1017 = call-dynamic "Measure_GetData_SpectraOutput.vi"("error in (no error)"=w2046, "Abstract_CCD in"=w2045) -> ("error out"=w2034:errorcluster, "Spectra"=w2035:dbl[], "Abstract_CCD out"=w2033:refnum<class "Abstract_CCD.lvclass">, "Time"=w2040:dbl)  [unwired: 6 in]
              n1018 = Add(x=w2043, y=w2044) -> (x+y=w2037:i32)
              n1019 = Replace Array Subset(array=w2041, new element=w2040, index=w2037) -> (w2042:dbl[])
              n1020 = Replace Array Subset(array=w2039, new element=w2035, index (dim 0)=w2037, index (dim 1)=0 ("disabled index (row)")) -> (w2038:dbl[][][])  [unwired: 1 in]
            }
            n1021 = flat-sequence {
              tunnel: w1970 -> [_]
              tunnel: [w2032] -> w1969
              frame #0 {
                n1022 = call <vilib>:"High Resolution Relative Seconds.vi"() -> ("relative seconds"=w2032:dbl)
              }
            }
            n1023 = Subtract(x=w1968, y=w1969) -> (x-y=→"x-y":dbl)
            n1024 = Array Size(array=w1974) -> (size(s)=w2002:i32[])
            n1025 = Index Array(array=w2002, index #1=0 ("index"), index #2=1 ("index"), index #3=2 ("index")) -> (element #1=w1999:i32, element #2=w2000:i32, element #3=w2001:i32)
            n1026 = Bundle By Name(cluster=T15 {"Image"=[], "Frame Size"={"F"=0, "Y"=0, "X"=0}} ("Cluster"), "Image"=w1974, "Frame Size.F"=w1999, "Frame Size.Y"=w2000, "Frame Size.X"=w2001) -> (w1995:T15)
            n1027 = Build Array(w1995) -> (w1994:T14)
            n1028 = Bundle By Name(cluster=w2029, "QueueAction"=DataQueue_Action."Spectrometer_Measure", "Data_Raw"=w1994, "Time"=w1976) -> (w2028:T8)
            n1029 = Enqueue Element(queue=w2026, element=w2028) -> (queue out=w2025:refnum<queue>)  [unwired: 2 in, 2 out]
          }
          frame "Spectrometer_SetIntegrationTime" {
            n1030 = Unbundle By Name(w2095) -> ("Numeric 1"=w2097:dbl)
            n1031 = Unbundle By Name(w2091) -> ("Abstract_CCD.lvclass"=w2099:refnum<class "Abstract_CCD.lvclass">)
            n1032 = Unbundle By Name(w2095) -> ("TabControl"=w2087:T10, "Boolean 1"=w2094:bool)
            n1033 = node(w2097) -> (w2096:dbl[unit])
            n1034 = call-dynamic "Set_ExposureTime.vi"("error in (no error)"=w2098, "Exposure Time"=w2096, "Abstract_CCD in"=w2099) -> ("error out"=w2102:errorcluster, "Abstract_CCD out"=w2101:refnum<class "Abstract_CCD.lvclass">)  [unwired: 7 in]
            n1035 = call-dynamic "Get_FrameRate.vi"("error in (no error)"=w2102, "Abstract_CCD in"=w2101) -> ("error out"=w2092:errorcluster, "Frame Rate"=w2093:dbl[unit], "Abstract_CCD out"=w2090:refnum<class "Abstract_CCD.lvclass">)  [unwired: 7 in]
            n1036 = Bundle By Name(cluster=w2091, "Abstract_CCD.lvclass"=w2090) -> (w2089:T6)
            n1037 = case shown="\"Measure\"" w2087 {
              tunnel: w2094 -> [_ _ w2105]
              tunnel: w2093 -> [_ w2103 w2104]
              frame Default {
              }
              frame "Spectral Stability" {
                "SpectralStability_FrameRate" <- w2103
              }
              frame "Measure" {
                n1038 = case shown="True" w2105 {
                  tunnel: w2104 -> [_ w2109]
                  frame False {
                  }
                  frame True {
                    n1039 = property on="Program Spin Coater" class="Arr (strict)"() -> ("Value"=w2106:T2)  [unwired: 2 in, 2 out]
                    n1040 = property on="Seconds to Spin_Normal" class="DigNum (strict)"() -> ("Value"=w2111:dbl[unit])  [unwired: 2 in, 2 out]
                    n1041 = property on="Seconds after Spin" class="DigNum (strict)"() -> ("Value"=w2110:dbl[unit])  [unwired: 2 in, 2 out]
                    n1042 = call "CalculateFrames_v03.vi"("Program Spin Coater"=w2106, "Seconds End"=w2110, "Seconds Start"=w2111, "Frame Rate"=w2109) -> ("Time"=w2108:dbl, "Frames"=w2107:i32)  [unwired: 6 in]
                    n1043 = property on="Frames" class="DigNum (strict)"("Value"=w2107) -> ()  [unwired: 2 in, 2 out]
                    n1044 = property on="Overall Time" class="DigNum (strict)"("Value"=w2108) -> ()  [unwired: 2 in, 2 out]
                  }
                }
                "Measure_FrameRate" <- w2104
              }
            }
          }
          frame "Spectrometer_SetFrames" {
            n1045 = Unbundle By Name(w2113) -> ("Abstract_CCD.lvclass"=w2118:refnum<class "Abstract_CCD.lvclass">)
            n1046 = Unbundle By Name(w2121) -> ("Numeric 1"=w2115:dbl)
            n1047 = call-dynamic "Set_Frames.vi"("error in (no error)"=w2117, "Frames"=w2115, "Abstract_CCD in"=w2118) -> ("error out"=w2116:errorcluster, "Abstract_CCD out"=w2112:refnum<class "Abstract_CCD.lvclass">)  [unwired: 7 in]
            n1048 = Bundle By Name(cluster=w2113, "Abstract_CCD.lvclass"=w2112) -> (w2114:T6)
          }
          frame "Spectrometer_SetDarkspec" {
            w2136 = T8 {"QueueAction"=enum."TimeOut", "Data"=[], "Data_Raw"=[], "Data_Dark"=[], "Data_Ref"=[], "Device Information"=[], "Numeric Control"=0.0, "Boolean"=FALSE, "Wavelength"=[], "Time"=[], "Time Stamp"=timestamp(0 s since 1904-01-01), "Numeric Control 2"=0.0, "TabControl"=enum."Measure", "Numeric Control 3"=0.0}  # DataQueue
            n1049 = Unbundle By Name(w2131) -> ("Abstract_CCD.lvclass"=w2129:refnum<class "Abstract_CCD.lvclass">)
            n1050 = call-dynamic "Measure.vi"("error in (no error)"=w2128, "Abstract_CCD in"=w2129) -> ("error out"=w2126:errorcluster, "Data Raw"=w2133:T14, "Abstract_CCD out"=w2127:refnum<class "Abstract_CCD.lvclass">)  [unwired: 3 in, 4 out]
            n1051 = Bundle By Name(cluster=w2136, "QueueAction"=DataQueue_Action."Set_Dark", "Data_Dark"=w2133) -> (w2137:T8)
            n1052 = Enqueue Element(queue=w2135, element=w2137) -> (queue out=w2132:refnum<queue>)  [unwired: 2 in, 2 out]
            n1053 = Bundle By Name(cluster=w2131, "Abstract_CCD.lvclass"=w2127) -> (w2130:T6)
            n1054 = property on="Measure:\nRecord_Darkspec" class="Bool (strict)"(error in=w2126, "Value"=FALSE ("Record_Darkspec")) -> (error out=w2124:errorcluster)  [unwired: 1 in, 1 out]
            n1055 = property on="SpectralStability:\nRecord_Darkspec" class="Bool (strict)"(error in=w2124, "Value"=FALSE ("SpectralStability:\nRecord_Darkspec")) -> (error out=w2123:errorcluster)  [unwired: 1 in, 1 out]
          }
          frame "Spectrometer_SetReference" {
            w2151 = T8 {"QueueAction"=enum."TimeOut", "Data"=[], "Data_Raw"=[], "Data_Dark"=[], "Data_Ref"=[], "Device Information"=[], "Numeric Control"=0.0, "Boolean"=FALSE, "Wavelength"=[], "Time"=[], "Time Stamp"=timestamp(0 s since 1904-01-01), "Numeric Control 2"=0.0, "TabControl"=enum."Measure", "Numeric Control 3"=0.0}  # DataQueue
            n1056 = Unbundle By Name(w2146) -> ("Abstract_CCD.lvclass"=w2143:refnum<class "Abstract_CCD.lvclass">)
            n1057 = call-dynamic "Measure.vi"("error in (no error)"=w2144, "Abstract_CCD in"=w2143) -> ("error out"=w2141:errorcluster, "Data Raw"=w2148:T14, "Abstract_CCD out"=w2142:refnum<class "Abstract_CCD.lvclass">)  [unwired: 3 in, 4 out]
            n1058 = Bundle By Name(cluster=w2151, "QueueAction"=DataQueue_Action."Set_Ref", "Data_Ref"=w2148) -> (w2152:T8)
            n1059 = Enqueue Element(queue=w2150, element=w2152) -> (queue out=w2147:refnum<queue>)  [unwired: 2 in, 2 out]
            n1060 = Bundle By Name(cluster=w2146, "Abstract_CCD.lvclass"=w2142) -> (w2145:T6)
            n1061 = property on="Record RefSpec" class="Bool (strict)"(error in=w2141, "Value"=FALSE ("Record RefSpec")) -> (error out=w2140:errorcluster)  [unwired: 1 in, 1 out]
          }
          frame "Spectrometer_SetTriggerMode" {
            n1062 = Unbundle By Name(w2157) -> ("Abstract_CCD.lvclass"=w2162:refnum<class "Abstract_CCD.lvclass">)
            n1063 = Unbundle By Name(w2161) -> ("Numeric 1"=w2159:dbl)
            n1064 = call-dynamic "Set_TriggerMode.vi"("error in (no error)"=w2160, "Trigger Mode"=w2159, "Abstract_CCD in"=w2162) -> ("error out"=w2158:errorcluster, "Abstract_CCD out"=w2156:refnum<class "Abstract_CCD.lvclass">)  [unwired: 7 in]
            n1065 = Bundle By Name(cluster=w2157, "Abstract_CCD.lvclass"=w2156) -> (w2155:T6)
          }
          frame "Spectrometer_DeviceInformation" {
            w2170 = T8 {"QueueAction"=enum."TimeOut", "Data"=[], "Data_Raw"=[], "Data_Dark"=[], "Data_Ref"=[], "Device Information"=[], "Numeric Control"=0.0, "Boolean"=FALSE, "Wavelength"=[], "Time"=[], "Time Stamp"=timestamp(0 s since 1904-01-01), "Numeric Control 2"=0.0, "TabControl"=enum."Measure", "Numeric Control 3"=0.0}  # DataQueue
            n1066 = Unbundle By Name(w2164) -> ("Abstract_CCD.lvclass"=w2172:refnum<class "Abstract_CCD.lvclass">)
            n1067 = call-dynamic "Get_DeviceInformation.vi"("error in (no error)"=w2171, "Abstract_CCD in"=w2172) -> ("error out"=w2166:errorcluster, "Array"=w2173:string[])  [unwired: 7 in, 1 out]
            n1068 = Bundle By Name(cluster=w2170, "QueueAction"=DataQueue_Action."Transfer_Settings", "Device Information"=w2173) -> (w2168:T8)
            n1069 = Enqueue Element(queue=w2169, element=w2168, error in (no error)=w2166) -> (queue out=w2167:refnum<queue>, error out=w2165:errorcluster)  [unwired: 1 in, 1 out]
          }
          frame "Arduino_Init" {
            n1070 = Unbundle By Name(w2185) -> ("SpinCoater.lvclass"=w2184:refnum<class "SpinCoater.lvclass">)
            n1071 = call-dynamic "Init.vi"("error in (no error)"=w2183, "Variant"="Port Arduino", "SpinCoater in"=w2184) -> ("error out"=w2180:errorcluster, "SpinCoater out"=w2181:refnum<class "SpinCoater.lvclass">)  [unwired: 7 in]
            n1072 = call-dynamic "IsInit.vi"("error in (no error)"=w2180, "SpinCoater in"=w2181) -> ("error out"=w2177:errorcluster, "Init"=w2178:bool, "SpinCoater out"=w2179:refnum<class "SpinCoater.lvclass">)  [unwired: 7 in]
            n1073 = property on="Arduino" class="Bool (strict)"("Value"=w2178) -> ()  [unwired: 2 in, 2 out]
            n1074 = case shown="False" w2178 {
              tunnel: [w2189 w2191] -> w2186
              tunnel: w2177 -> [w2189 w2191]
              frame False {
              }
              frame True {
                n1075 = property on="Program Spin Coater" class="Arr (strict)"() -> ("Value"=w2190:T2)  [unwired: 2 in, 2 out]
                n1076 = property on="Program Spin Coater" class="Arr (strict)"("Val(Sgnl)"=w2190) -> ()  [unwired: 2 in, 2 out]
              }
            }
            n1077 = Bundle By Name(cluster=w2185, "SpinCoater.lvclass"=w2179) -> (w2187:T6)
          }
          frame "Arduino_Close" {
            n1078 = Unbundle By Name(w2194) -> ("SpinCoater.lvclass"=w2202:refnum<class "SpinCoater.lvclass">)
            n1079 = property on="Arduino" class="Bool (strict)"() -> (error out=w2196:errorcluster, "Value"=w2195:bool)  [unwired: 2 in, 1 out]
            n1080 = property on="Arduino" class="Bool (strict)"(error in=w2196, "Value"=FALSE ("Arduino")) -> ()  [unwired: 1 in, 2 out]
            n1081 = case shown="False" w2195 {
              tunnel: w2202 -> [w2203 w2208]
              tunnel: w2201 -> [w2204 w2207]
              tunnel: [w2204 w2206] -> w2200
              tunnel: [w2203 w2205] -> w2193
              frame False {
              }
              frame True {
                n1082 = call-dynamic "Close.vi"("error in (no error)"=w2207, "SpinCoater in"=w2208) -> ("error out"=w2206:errorcluster, "SpinCoater out"=w2205:refnum<class "SpinCoater.lvclass">)  [unwired: 8 in]
              }
            }
            n1083 = Bundle By Name(cluster=w2194, "SpinCoater.lvclass"=w2193) -> (w2192:T6)
          }
          frame "Arduino_LoadProgram" {
            n1084 = Unbundle By Name(w2220) -> ("Spin Prg v07"=w2211:T2, "Numeric 1"=w2219:dbl, "Numeric 2"=w2210:dbl)
            n1085 = Unbundle By Name(w2215) -> ("SpinCoater.lvclass"=w2218:refnum<class "SpinCoater.lvclass">)
            n1086 = node(w2219) -> (w2217:dbl[unit])
            n1087 = node(w2210) -> (w2209:dbl[unit])
            n1088 = call-dynamic "Program_Load_v03.vi"("Time Spin"=w2209, "error in (no error)"=w2216, "Time Start"=w2217, "Program Spin Coater"=w2211, "SpinCoater in"=w2218) -> ("error out"=w2213:errorcluster, "SpinCoater out"=w2214:refnum<class "SpinCoater.lvclass">)  [unwired: 5 in]
            n1089 = Bundle By Name(cluster=w2215, "SpinCoater.lvclass"=w2214) -> (w2212:T6)
          }
          frame "Arduino_StartProgram" {
            n1090 = Unbundle By Name(w2230) -> ("SpinCoater.lvclass"=w2227:refnum<class "SpinCoater.lvclass">)
            n1091 = Unbundle By Name(w2224) -> ("Numeric 1"=w2223:dbl)
            n1092 = call-dynamic "Program_Run.vi"("error in (no error)"=w2226, "Numeric"=w2223, "SpinCoater in"=w2227) -> ("error out"=w2225:errorcluster)  [unwired: 7 in, 1 out]
            n1093 = property on="Action" class="Str"("Value"="Measuring" ("Action")) -> ()  [unwired: 2 in, 2 out]
          }
          frame "Arduino_SetSpeed" {
            n1094 = Unbundle By Name(w2239) -> ("SpinCoater.lvclass"=w2235:refnum<class "SpinCoater.lvclass">)
            n1095 = Unbundle By Name(w2238) -> ("Numeric 1"=w2237:dbl)
            n1096 = To Unsigned Long Integer(number=w2237) -> (unsigned 32bit integer=w2233:u32)
            n1097 = call-dynamic "Debug_SetSpeed.vi"("error in (no error)"=w2234, "Speed"=w2233, "SpinCoater in"=w2235) -> ("error out"=w2232:errorcluster)  [unwired: 7 in, 1 out]
          }
          frame "Arduino_SetMillis" {
            n1098 = Unbundle By Name(w2245) -> ("SpinCoater.lvclass"=w2244:refnum<class "SpinCoater.lvclass">)
            n1099 = Unbundle By Name(w2247) -> ("Numeric 1"=w2249:dbl)
            n1100 = To Unsigned Long Integer(number=w2249) -> (unsigned 32bit integer=w2241:u32)
            n1101 = call-dynamic "Debug_SetMillis.vi"("error in (no error)"=w2243, "Milliseconds"=w2241, "SpinCoater in"=w2244) -> ("error out"=w2242:errorcluster)  [unwired: 7 in, 1 out]
          }
          frame "Arduino_StopSpin" {
            n1102 = Unbundle By Name(w2253) -> ("SpinCoater.lvclass"=w2252:refnum<class "SpinCoater.lvclass">)
            n1103 = call-dynamic "Stop_Spin.vi"("error in (no error)"=w2251, "SpinCoater in"=w2252) -> ("error out"=w2250:errorcluster)  [unwired: 8 in, 1 out]
          }
          frame "Arduino_ShortStop" {
            n1104 = Unbundle By Name(w2259) -> ("SpinCoater.lvclass"=w2258:refnum<class "SpinCoater.lvclass">)
            n1105 = call-dynamic "Stop_Short.vi"("error in (no error)"=w2257, "SpinCoater in"=w2258) -> ("error out"=w2256:errorcluster)  [unwired: 8 in, 1 out]
          }
          frame "Arduino_Shutter_SetPosition" {
            n1106 = Unbundle By Name(w2268) -> ("Numeric 1"=w2267:dbl)
            n1107 = Unbundle By Name(w2270) -> ("SpinCoater.lvclass"=w2269:refnum<class "SpinCoater.lvclass">)
            n1108 = Number To Decimal String(number=w2267) -> (decimal integer string=w2266:string)  [unwired: 1 in]
            n1109 = Concatenate Strings("!shu_M" ("string"), w2266) -> (w2264:string)
            n1110 = call-dynamic "Send_String.vi"("error in (no error)"=w2263, "String"=w2264, "SpinCoater in"=w2269) -> ("error out"=w2262:errorcluster)  [unwired: 6 in, 2 out]
          }
          frame "Arduino_Shutter_Close" {
            n1111 = Unbundle By Name(w2277) -> ("SpinCoater.lvclass"=w2276:refnum<class "SpinCoater.lvclass">)
            n1112 = call-dynamic "Send_String.vi"("error in (no error)"=w2275, "String"="!shuOFF" ("string"), "SpinCoater in"=w2276) -> ("error out"=w2274:errorcluster)  [unwired: 6 in, 2 out]
          }
          frame "Arduino_Shutter_Open" {
            n1113 = Unbundle By Name(w2284) -> ("SpinCoater.lvclass"=w2283:refnum<class "SpinCoater.lvclass">)
            n1114 = call-dynamic "Send_String.vi"("error in (no error)"=w2282, "String"="!shuON" ("string"), "SpinCoater in"=w2283) -> ("error out"=w2281:errorcluster)  [unwired: 6 in, 2 out]
          }
          frame "Measure_Stop" {
            w2293 = T8 {"QueueAction"=enum."TimeOut", "Data"=[], "Data_Raw"=[], "Data_Dark"=[], "Data_Ref"=[], "Device Information"=[], "Numeric Control"=0.0, "Boolean"=FALSE, "Wavelength"=[], "Time"=[], "Time Stamp"=timestamp(0 s since 1904-01-01), "Numeric Control 2"=0.0, "TabControl"=enum."Measure", "Numeric Control 3"=0.0}  # DataQueue
            n1115 = Bundle By Name(cluster=w2293, "QueueAction"=DataQueue_Action."Stop_Measurement") -> (w2294:T8)
            n1116 = Enqueue Element(queue=w2291, element=w2294, error in (no error)=w2288) -> (queue out=w2290:refnum<queue>, error out=w2287:errorcluster)  [unwired: 1 in, 1 out]
          }
          frame "Measure_InSitu" {
            w2335 = T11 {"QueueAction"=enum."TimeOut", "Numeric 1"=0.0, "Numeric 2"=0.0, "Boolean 1"=FALSE, "Boolean 2"=FALSE, "Spin Program"=[], "Spin Prg v07"=[], "Time Stamp"=timestamp(0 s since 1904-01-01), "TabControl"=enum."Measure"}  # Device Queue
            w2342 = T11 {"QueueAction"=enum."TimeOut", "Numeric 1"=0.0, "Numeric 2"=0.0, "Boolean 1"=FALSE, "Boolean 2"=FALSE, "Spin Program"=[], "Spin Prg v07"=[], "Time Stamp"=timestamp(0 s since 1904-01-01), "TabControl"=enum."Measure"}  # Device Queue
            n1117 = Bundle By Name(cluster=w2342, "QueueAction"=DeviceQueue_Action."Spectrometer_SetTriggerMode", "Numeric 1"=1.0) -> (w2340:T11)
            n1118 = Bundle By Name(cluster=w2335, "QueueAction"=DeviceQueue_Action."Spectrometer_DeviceInformation") -> (w2332:T11)
            n1119 = Bundle By Name(cluster=w2332, "QueueAction"=DeviceQueue_Action."Spectrometer_StartMeasurement") -> (w2328:T11)
            n1120 = Enqueue Element(queue=w2341, element=w2340, error in (no error)=w2297) -> (queue out=w2337:refnum<queue>, error out=w2338:errorcluster)  [unwired: 1 in, 1 out]
            n1121 = property on="Frames" class="DigNum (strict)"() -> ("Value"=w2298:i32)  [unwired: 2 in, 2 out]
            n1122 = Bundle By Name(cluster=w2328, "QueueAction"=DeviceQueue_Action."Arduino_StartProgram") -> (w2323:T11)
            n1123 = Enqueue Element(queue=w2337, element=w2332, error in (no error)=w2338) -> (queue out=w2334:refnum<queue>, error out=w2333:errorcluster)  [unwired: 1 in, 1 out]
            n1124 = Bundle By Name(cluster=w2323, "QueueAction"=DeviceQueue_Action."Spectrometer_GetData", "Numeric 1"="Dividider Get Spectra") -> (w2318:T11)
            n1125 = Divide(x=w2298, y="Dividider Get Spectra") -> (x/y=w2330:dbl)
            n1126 = Round Toward +Infinity(x=w2330) -> (ceil(x): smallest int >= x=w2329:dbl)
            n1127 = Enqueue Element(queue=w2334, element=w2328, error in (no error)=w2333) -> (queue out=w2327:refnum<queue>, error out=w2326:errorcluster)  [unwired: 1 in, 1 out]
            n1128 = Enqueue Element(queue=w2327, element=w2323, error in (no error)=w2326) -> (queue out=w2324:refnum<queue>, error out=w2321:errorcluster)  [unwired: 1 in, 1 out]
            n1129 = for {
              N: w2329 -> [_]
              shift-right: [w2345] -> w2320
              shift-left: w2324 -> [w2349]
              tunnel: w2318 -> [w2346]
              shift-right: [w2347] -> w2319
              shift-left: w2321 -> [w2348]
              n1130 = Enqueue Element(queue=w2349, element=w2346, error in (no error)=w2348) -> (queue out=w2345:refnum<queue>, error out=w2347:errorcluster)  [unwired: 1 in, 1 out]
            }
            n1131 = Bundle By Name(cluster=w2318, "QueueAction"=DeviceQueue_Action."Spectrometer_StopMeasurement") -> (w2314:T11)
            n1132 = property on="Measure_FramesSpectrometer" class="DigNum (strict)"() -> ("Value"=w2300:dbl)  [unwired: 2 in, 2 out]
            n1133 = Bundle By Name(cluster=w2314, "QueueAction"=DeviceQueue_Action."Measure_Stop") -> (w2307:T11)
            n1134 = Enqueue Element(queue=w2320, element=w2314, error in (no error)=w2319) -> (queue out=w2315:refnum<queue>, error out=w2316:errorcluster)  [unwired: 1 in, 1 out]
            n1135 = Bundle By Name(cluster=w2307, "QueueAction"=DeviceQueue_Action."Spectrometer_SetTriggerMode", "Numeric 1"=0.0) -> (w2302:T11)
            n1136 = Enqueue Element(queue=w2315, element=w2307, error in (no error)=w2316) -> (queue out=w2310:refnum<queue>, error out=w2311:errorcluster)  [unwired: 1 in, 1 out]
            n1137 = Bundle By Name(cluster=w2302, "QueueAction"=DeviceQueue_Action."Spectrometer_SetFrames", "Numeric 1"=w2300) -> (w2299:T11)
            n1138 = Enqueue Element(queue=w2310, element=w2302, error in (no error)=w2311) -> (queue out=w2309:refnum<queue>, error out=w2308:errorcluster)  [unwired: 1 in, 1 out]
            n1139 = Enqueue Element(queue=w2309, element=w2299, error in (no error)=w2308) -> (queue out=w2303:refnum<queue>, error out=w2304:errorcluster)  [unwired: 1 in, 1 out]
          }
          frame "Measure_InSituAdvanced" {
            w2437 = T11 {"QueueAction"=enum."TimeOut", "Numeric 1"=0.0, "Numeric 2"=0.0, "Boolean 1"=FALSE, "Boolean 2"=FALSE, "Spin Program"=[], "Spin Prg v07"=[], "Time Stamp"=timestamp(0 s since 1904-01-01), "TabControl"=enum."Measure"}  # Device Queue
            n1140 = property on="Dividider Get Spectra" class="DigNum (strict)"() -> ("Value"=w2399:u32)  [unwired: 2 in, 2 out]
            n1141 = Bundle By Name(cluster=w2437, "QueueAction"=DeviceQueue_Action."Spectrometer_SetTriggerMode", "Numeric 1"=1.0) -> (w2397:T11)
            n1142 = Bundle By Name(cluster=w2397, "QueueAction"=DeviceQueue_Action."Spectrometer_DeviceInformation") -> (w2429:T11)
            n1143 = Bundle By Name(cluster=w2429, "QueueAction"=DeviceQueue_Action."Spectrometer_StartMeasurement") -> (w2425:T11)
            n1144 = Enqueue Element(queue=w2436, element=w2397, error in (no error)=w2400) -> (queue out=w2433:refnum<queue>, error out=w2434:errorcluster)  [unwired: 1 in, 1 out]
            n1145 = Bundle By Name(cluster=w2425, "QueueAction"=DeviceQueue_Action."Arduino_StartProgram", "Numeric 1"=1.0) -> (w2420:T11)
            n1146 = property on="Frames" class="DigNum (strict)"() -> ("Value"=w2401:i32)  [unwired: 2 in, 2 out]
            n1147 = Unbundle By Name(w2385) -> ("Time Stamp"=w2384:timestamp)
            n1148 = Enqueue Element(queue=w2433, element=w2429, error in (no error)=w2434) -> (queue out=w2431:refnum<queue>, error out=w2430:errorcluster)  [unwired: 1 in, 1 out]
            n1149 = Divide(x=w2401, y=w2399) -> (x/y=w2427:dbl)
            n1150 = Bundle By Name(cluster=w2420, "QueueAction"=DeviceQueue_Action."Spectrometer_GetData", "Numeric 1"=w2399) -> (w2415:T11)
            n1151 = Round Toward +Infinity(x=w2427) -> (ceil(x): smallest int >= x=w2426:dbl)
            n1152 = Enqueue Element(queue=w2431, element=w2425, error in (no error)=w2430) -> (queue out=w2424:refnum<queue>, error out=w2423:errorcluster)  [unwired: 1 in, 1 out]
            n1153 = Enqueue Element(queue=w2424, element=w2420, error in (no error)=w2423) -> (queue out=w2421:refnum<queue>, error out=w2418:errorcluster)  [unwired: 1 in, 1 out]
            n1154 = Bundle By Name(cluster=w2415, "QueueAction"=DeviceQueue_Action."Spectrometer_StopMeasurement") -> (w2411:T11)
            n1155 = for {
              N: w2426 -> [_]
              shift-right: [w2487] -> w2417
              shift-left: w2421 -> [w2491]
              tunnel: w2415 -> [w2488]
              shift-right: [w2489] -> w2416
              shift-left: w2418 -> [w2490]
              n1156 = Enqueue Element(queue=w2491, element=w2488, error in (no error)=w2490) -> (queue out=w2487:refnum<queue>, error out=w2489:errorcluster)  [unwired: 1 in, 1 out]
            }
            n1157 = property on="periodic time" class="DigNum (strict)"() -> ("Value"=w2396:dbl[unit])  [unwired: 2 in, 2 out]
            n1158 = Bundle By Name(cluster=w2411, "QueueAction"=DeviceQueue_Action."Measure_Stop") -> (w2404:T11)
            n1159 = node(w2396) -> (w2368:dbl)
            n1160 = property on="Duration after" class="DigNum (strict)"() -> ("Value"=w2395:dbl[unit])  [unwired: 2 in, 2 out]
            n1161 = property on="periodic time" class="DigNum (strict)"() -> ("Value"=w2394:dbl[unit])  [unwired: 2 in, 2 out]
            n1162 = Bundle By Name(cluster=w2404, "QueueAction"=DeviceQueue_Action."Spectrometer_SetTriggerMode", "Numeric 1"=0.0) -> (w2359:T11)
            n1163 = Enqueue Element(queue=w2417, element=w2411, error in (no error)=w2416) -> (queue out=w2412:refnum<queue>, error out=w2413:errorcluster)  [unwired: 1 in, 1 out]
            n1164 = node(w2395) -> (w2389:dbl)
            n1165 = node(w2394) -> (w2388:dbl)
            n1166 = Bundle By Name(cluster=w2359, "QueueAction"=DeviceQueue_Action."Wait", "Numeric 1"=w2368) -> (w2370:T11)
            n1167 = Enqueue Element(queue=w2412, element=w2404, error in (no error)=w2413) -> (queue out=w2407:refnum<queue>, error out=w2408:errorcluster)  [unwired: 1 in, 1 out]
            n1168 = Not Equal To 0?(x=w2388) -> (x != 0?=w2392:bool)
            n1169 = Not Equal To 0?(x=w2389) -> (x != 0?=w2393:bool)
            n1170 = Bundle By Name(cluster=w2370, "QueueAction"=DeviceQueue_Action."Spectrometer_MeasureAdvanced", "Time Stamp"=w2384) -> (w2369:T11)
            n1171 = Divide(x=w2389, y=w2388) -> (x/y=w2390:dbl)
            n1172 = Enqueue Element(queue=w2407, element=w2359, error in (no error)=w2408) -> (queue out=w2406:refnum<queue>, error out=w2405:errorcluster)  [unwired: 1 in, 1 out]
            n1173 = And(x=w2393, y=w2392) -> (x .and. y?=w2391:bool)
            n1174 = Round Toward +Infinity(x=w2390) -> (ceil(x): smallest int >= x=w2387:dbl)
            n1175 = Bundle By Name(cluster=w2369, "QueueAction"=DeviceQueue_Action."Arduino_SetSpeed", "Numeric 1"=1500.0) -> (w2379:T11)
            n1176 = property on="Frames for Ref/Dark" class="DigNum (strict)"() -> ("Value"=w2358:dbl)  [unwired: 2 in, 2 out]
            n1177 = property on="Measure_FrameRate" class="DigNum (strict)"() -> ("Value"=w2376:dbl[unit])  [unwired: 2 in, 2 out]
            n1178 = Bundle By Name(cluster=w2379, "Numeric 1"=0.0) -> (w2372:T11)
            n1179 = Divide(x=w2358, y=w2376) -> (x/y=w2377:dbl[unit])
            n1180 = node(w2377) -> (w2367:dbl)
            n1181 = Subtract(x=w2368, y=w2367) -> (x-y=w2366:dbl)
            n1182 = Bundle By Name(cluster=w2370, "Numeric 1"=w2366) -> (w2365:T11)
            n1183 = property on="Measure_FramesSpectrometer" class="DigNum (strict)"() -> ("Value"=w2351:dbl)  [unwired: 2 in, 2 out]
            n1184 = Bundle By Name(cluster=w2370, "Numeric 1"=1.0) -> (w2373:T11)
            n1185 = Round Toward +Infinity(x=w2367) -> (ceil(x): smallest int >= x=w2378:dbl)
            n1186 = Add(x=w2378, y=2.0) -> (x+y=w2374:dbl)
            n1187 = Bundle By Name(cluster=w2373, "Numeric 1"=w2374) -> (w2353:T11)
            n1188 = case shown="True" w2391 {
              tunnel: w2406 -> [w2441 w2443]
              tunnel: w2405 -> [w2440 w2446]
              tunnel: w2387 -> [_ w2459]
              tunnel: w2369 -> [_ w2458]
              tunnel: w2365 -> [_ w2454]
              tunnel: w2379 -> [_ w2453]
              tunnel: w2373 -> [_ w2452]
              tunnel: w2369 -> [_ w2451]
              tunnel: w2353 -> [_ w2450]
              tunnel: w2372 -> [_ w2449]
              tunnel: [w2440 w2448] -> w2357
              tunnel: [w2441 w2447] -> w2354
              tunnel: w2370 -> [_ w2442]
              frame False {
              }
              frame True {
                n1189 = Enqueue Element(queue=w2443, element=w2442, error in (no error)=w2446) -> (queue out=w2444:refnum<queue>, error out=w2445:errorcluster)  [unwired: 1 in, 1 out]
                n1190 = for {
                  N: w2459 -> [_]
                  shift-right: [w2480] -> w2456
                  shift-left: w2444 -> [w2486]
                  shift-right: [w2479] -> w2455
                  shift-left: w2445 -> [w2485]
                  tunnel: w2458 -> [w2484]
                  tunnel: w2454 -> [w2481]
                  n1191 = Enqueue Element(queue=w2486, element=w2484, error in (no error)=w2485) -> (queue out=w2482:refnum<queue>, error out=w2483:errorcluster)  [unwired: 1 in, 1 out]
                  n1192 = Enqueue Element(queue=w2482, element=w2481, error in (no error)=w2483) -> (queue out=w2480:refnum<queue>, error out=w2479:errorcluster)  [unwired: 1 in, 1 out]
                }
                n1193 = case shown="True" "Spin at end" {
                  tunnel: w2456 -> [w2461 w2478]
                  tunnel: w2455 -> [w2460 w2477]
                  tunnel: w2453 -> [_ w2472]
                  tunnel: w2452 -> [_ w2471]
                  tunnel: w2451 -> [_ w2470]
                  tunnel: w2450 -> [_ w2465]
                  tunnel: w2449 -> [_ w2464]
                  tunnel: [w2460 w2463] -> w2448
                  tunnel: [w2461 w2462] -> w2447
                  frame False {
                  }
                  frame True {
                    n1194 = Enqueue Element(queue=w2478, element=w2472, error in (no error)=w2477) -> (queue out=w2476:refnum<queue>, error out=w2475:errorcluster)  [unwired: 1 in, 1 out]
                    n1195 = Enqueue Element(queue=w2476, element=w2471, error in (no error)=w2475) -> (queue out=w2474:refnum<queue>, error out=w2473:errorcluster)  [unwired: 1 in, 1 out]
                    n1196 = Enqueue Element(queue=w2474, element=w2470, error in (no error)=w2473) -> (queue out=w2469:refnum<queue>, error out=w2468:errorcluster)  [unwired: 1 in, 1 out]
                    n1197 = Enqueue Element(queue=w2469, element=w2465, error in (no error)=w2468) -> (queue out=w2466:refnum<queue>, error out=w2467:errorcluster)  [unwired: 1 in, 1 out]
                    n1198 = Enqueue Element(queue=w2466, element=w2464, error in (no error)=w2467) -> (queue out=w2462:refnum<queue>, error out=w2463:errorcluster)  [unwired: 1 in, 1 out]
                  }
                }
              }
            }
            n1199 = Bundle By Name(cluster=w2353, "QueueAction"=DeviceQueue_Action."Arduino_Shutter_Close") -> (w2364:T11)
            n1200 = Bundle By Name(cluster=w2353, "QueueAction"=DeviceQueue_Action."Spectrometer_SetFrames", "Numeric 1"=w2351) -> (w2352:T11)
            n1201 = Enqueue Element(queue=w2354, element=w2352, error in (no error)=w2357) -> (queue out=w2355:refnum<queue>, error out=w2356:errorcluster)  [unwired: 1 in, 1 out]
            n1202 = Enqueue Element(queue=w2355, element=w2364, error in (no error)=w2356) -> (queue out=w2362:refnum<queue>, error out=w2361:errorcluster)  [unwired: 1 in, 1 out]
            "Nr After Spin" <- u16 0 ("Nr After Spin")
          }
          frame "Measure_InSituAdvanced_Short" {
            w2540 = T11 {"QueueAction"=enum."TimeOut", "Numeric 1"=0.0, "Numeric 2"=0.0, "Boolean 1"=FALSE, "Boolean 2"=FALSE, "Spin Program"=[], "Spin Prg v07"=[], "Time Stamp"=timestamp(0 s since 1904-01-01), "TabControl"=enum."Measure"}  # Device Queue
            n1203 = property on="Nr After Spin" class="DigNum (strict)"("Value"=u16 0 ("Nr After Spin")) -> ()  [unwired: 2 in, 2 out]
            n1204 = Bundle By Name(cluster=w2540, "QueueAction"=DeviceQueue_Action."Spectrometer_SetTriggerMode", "Numeric 1"=1.0) -> (w2502:T11)
            n1205 = Bundle By Name(cluster=w2502, "QueueAction"=DeviceQueue_Action."Spectrometer_DeviceInformation") -> (w2532:T11)
            n1206 = property on="Frames" class="DigNum (strict)"() -> ("Value"=w2493:i32)  [unwired: 2 in, 2 out]
            n1207 = Bundle By Name(cluster=w2532, "QueueAction"=DeviceQueue_Action."Spectrometer_StartMeasurement") -> (w2530:T11)
            n1208 = Enqueue Element(queue=w2539, element=w2502, error in (no error)=w2503) -> (queue out=w2536:refnum<queue>, error out=w2537:errorcluster)  [unwired: 1 in, 1 out]
            n1209 = Bundle By Name(cluster=w2530, "QueueAction"=DeviceQueue_Action."Arduino_StartProgram", "Numeric 1"=2.0) -> (w2525:T11)
            n1210 = Enqueue Element(queue=w2536, element=w2532, error in (no error)=w2537) -> (queue out=w2534:refnum<queue>, error out=w2533:errorcluster)  [unwired: 1 in, 1 out]
            n1211 = Bundle By Name(cluster=w2525, "QueueAction"=DeviceQueue_Action."Spectrometer_GetData_Short", "Numeric 2"=w2493) -> (w2520:T11)
            n1212 = Enqueue Element(queue=w2534, element=w2530, error in (no error)=w2533) -> (queue out=w2529:refnum<queue>, error out=w2528:errorcluster)  [unwired: 1 in, 1 out]
            n1213 = Enqueue Element(queue=w2529, element=w2525, error in (no error)=w2528) -> (queue out=w2526:refnum<queue>, error out=w2523:errorcluster)  [unwired: 1 in, 1 out]
            n1214 = Bundle By Name(cluster=w2520, "QueueAction"=DeviceQueue_Action."Spectrometer_StopMeasurement") -> (w2516:T11)
            n1215 = property on="Measure_FramesSpectrometer" class="DigNum (strict)"() -> ("Value"=w2504:dbl)  [unwired: 2 in, 2 out]
            n1216 = Enqueue Element(queue=w2526, element=w2520, error in (no error)=w2523) -> (queue out=w2522:refnum<queue>, error out=w2521:errorcluster)  [unwired: 1 in, 1 out]
            n1217 = Bundle By Name(cluster=w2516, "QueueAction"=DeviceQueue_Action."Measure_Stop") -> (w2509:T11)
            n1218 = Bundle By Name(cluster=w2509, "QueueAction"=DeviceQueue_Action."Spectrometer_SetTriggerMode", "Numeric 1"=0.0) -> (w2506:T11)
            n1219 = Enqueue Element(queue=w2522, element=w2516, error in (no error)=w2521) -> (queue out=w2517:refnum<queue>, error out=w2518:errorcluster)  [unwired: 1 in, 1 out]
            n1220 = Bundle By Name(cluster=w2506, "QueueAction"=DeviceQueue_Action."Spectrometer_SetFrames", "Numeric 1"=w2504) -> (w2498:T11)
            n1221 = Enqueue Element(queue=w2517, element=w2509, error in (no error)=w2518) -> (queue out=w2512:refnum<queue>, error out=w2513:errorcluster)  [unwired: 1 in, 1 out]
            n1222 = Enqueue Element(queue=w2512, element=w2506, error in (no error)=w2513) -> (queue out=w2511:refnum<queue>, error out=w2510:errorcluster)  [unwired: 1 in, 1 out]
            n1223 = Enqueue Element(queue=w2511, element=w2498, error in (no error)=w2510) -> (queue out=w2497:refnum<queue>, error out=w2496:errorcluster)  [unwired: 1 in, 1 out]
            n1224 = Bundle By Name(cluster=w2498, "QueueAction"=DeviceQueue_Action."Arduino_Shutter_Close") -> (w2501:T11)
            n1225 = Enqueue Element(queue=w2497, element=w2501, error in (no error)=w2496) -> (queue out=w2499:refnum<queue>, error out=w2492:errorcluster)  [unwired: 1 in, 1 out]
          }
          frame "Measure_Spectrum" {
            n1226 = Unbundle By Name(w2543) -> ("Time Stamp"=w2544:timestamp)
            n1227 = Bundle By Name(cluster=w2543, "QueueAction"=DeviceQueue_Action."Spectrometer_Measure", "Time Stamp"=w2544) -> (w2549:T11)
            n1228 = Bundle By Name(cluster=w2549, "QueueAction"=DeviceQueue_Action."Measure_Stop") -> (w2547:T11)
            n1229 = Enqueue Element(queue=w2555, element=w2549, error in (no error)=w2554) -> (queue out=w2550:refnum<queue>, error out=w2551:errorcluster)  [unwired: 1 in, 1 out]
            n1230 = Enqueue Element(queue=w2550, element=w2547, error in (no error)=w2551) -> (queue out=w2546:refnum<queue>, error out=w2545:errorcluster)  [unwired: 1 in, 1 out]
          }
          frame "Measure_SpectralStability" {
            n1231 = Bundle By Name(cluster=w2559, "QueueAction"=DeviceQueue_Action."Spectrometer_DeviceInformation") -> (w2562:T11)
            n1232 = property on="SpectralStability_\nFrameRate" class="DigNum (strict)"() -> ("Value"=w2582:dbl[unit])  [unwired: 2 in, 2 out]
            n1233 = property on="SpectralStability_\nFramesSpectrometer" class="DigNum (strict)"() -> ("Value"=w2583:dbl)  [unwired: 2 in, 2 out]
            n1234 = Bundle By Name(cluster=w2562, "QueueAction"=DeviceQueue_Action."Spectrometer_Measure") -> (w2561:T11)
            n1235 = Enqueue Element(queue=w2565, element=w2562, error in (no error)=w2564) -> (queue out=w2567:refnum<queue>, error out=w2566:errorcluster)  [unwired: 1 in, 1 out]
            n1236 = Divide(x=w2583, y=w2582) -> (x/y=w2577:dbl[unit])
            n1237 = Unbundle By Name(w2559) -> ("Numeric 1"=w2558:dbl)
            n1238 = Subtract(x="SpectralStability_\nPeriodicTime", y=w2577) -> (x-y=w2576:dbl[unit])
            n1239 = Enqueue Element(queue=w2567, element=w2561, error in (no error)=w2566) -> (queue out=w2581:refnum<queue>, error out=w2580:errorcluster)  [unwired: 1 in, 1 out]
            n1240 = node(w2576) -> (w2575:dbl)
            n1241 = Decrement(x=w2558) -> (x-1=w2557:dbl)
            n1242 = Bundle By Name(cluster=w2561, "QueueAction"=DeviceQueue_Action."Wait", "Numeric 1"=w2575) -> (w2571:T11)
            n1243 = for {
              N: w2557 -> [_]
              shift-right: [w2587] -> w2574
              shift-left: w2581 -> [w2593]
              shift-right: [w2586] -> w2573
              shift-left: w2580 -> [w2592]
              tunnel: w2571 -> [w2589]
              tunnel: w2561 -> [w2588]
              n1244 = Enqueue Element(queue=w2593, element=w2589, error in (no error)=w2592) -> (queue out=w2591:refnum<queue>, error out=w2590:errorcluster)  [unwired: 1 in, 1 out]
              n1245 = Enqueue Element(queue=w2591, element=w2588, error in (no error)=w2590) -> (queue out=w2587:refnum<queue>, error out=w2586:errorcluster)  [unwired: 1 in, 1 out]
            }
            n1246 = Bundle By Name(cluster=w2571, "QueueAction"=DeviceQueue_Action."Measure_Stop") -> (w2570:T11)
            n1247 = Enqueue Element(queue=w2574, element=w2570, error in (no error)=w2573) -> (queue out=w2568:refnum<queue>, error out=w2569:errorcluster)  [unwired: 1 in, 1 out]
          }
        }
      }
      frame Error {
        w2598 = T19 4 items=["no dialog", "OK message", "continue or stop message", "OK message + warnings", "continue/stop + warnings"] ("type of dialog (OK msg:1)")
        n1248 = call <vilib>:"General Error Handler.vi"("type of dialog (OK msg:1)"=w2598, "error in (no error)"=w2599) -> ("error out"=w2597:errorcluster)  [unwired: 9 in, 4 out]
        n1249 = call <vilib>:"Clear Errors.vi"("error in (no error)"=w2597) -> ("error out"=w2596:errorcluster)  [unwired: 5 in, 1 out]
      }
    }
  }
  n1250 = disable-structure shown="Disabled" {
    frame Disabled {
      w2602 = T11 {"QueueAction"=enum."TimeOut", "Numeric 1"=0.0, "Numeric 2"=0.0, "Boolean 1"=FALSE, "Boolean 2"=FALSE, "Spin Program"=[], "Spin Prg v07"=[], "Time Stamp"=timestamp(0 s since 1904-01-01), "TabControl"=enum."Measure"}  # Device Queue
      n1251 = Bundle By Name(cluster=w2602, "QueueAction"=DeviceQueue_Action."Arduino_SetSpeed") -> (w2603:T11)  [unwired: 1 in]
      n1252 = Enqueue Element(element=w2603) -> ()  [unwired: 3 in, 3 out]
    }
    frame Enabled {
    }
  }
  n1253 = Release Queue(queue=w13) -> ()  [unwired: 2 in, 3 out]
  n1254 = Release Queue(queue=w14) -> ()  [unwired: 2 in, 3 out]
